vi "G_LCM.vi"() -> ()   [LabVIEW 2015]
panel:
  out "VISION_LANE_PT":T1={"hash"=5997167734802894298, "sys time"=0, "size"=0, "x"=[], "y"=[]} {"hash" format="%016x"}
  out "queue velo":refnum<queue>
  out "queue velo raw":refnum<queue>
  out "SLAM":T2={"hash"=8611666821338907869, "sys time"=0, "dt"=0.0, "x"=0.0, "y"=0.0, "speed"=0.0, "heading"=0.0, "yaw_rate"=0.0} {"hash" format="%016x"}
  out "VISION_STOPLINE":T3={"hash"=-9133130956553482184, "sys time"=0, "stopline_exist"=FALSE, "stopline_distance"=0.0} {"hash" format="%016x"}
  out "VISION_LANE":T4={"hash"=2187367745111948818, "sys time"=0, "left_lane_exist"=FALSE, "right_lane_exist"=FALSE, "left_lane_dot"=0.0, "right_lane_dot"=0.0} {"hash" format="%016x"}
  out "AVM":cluster{"hash":i64, "sys time":i64}={"hash"=-4935458055730020940, "sys time"=0} {"hash" format="%x"}
  out "queue ibeo":refnum<queue>
  out "CON_T 2":T5={"hash"=6240213546654873975, "sys time"=0, "Auto"=FALSE, "Run"=FALSE, "Solenoid"=FALSE, "T lim"=FALSE, "brk_enc"=0, "B PWM"=0, "T PWM"=0, "ref_vel"=0.0, "ref_bkr_enc"=0.0, "ref_apv"=0.0, "ref_steer"=0.0, "net address"=0} {"net address" format="%08x"; "hash" format="%016x"}
  out "VELO_384":T6={"hash"=-1208058655852198207, "sys time"=0, "Timestamp"=0, "Rot_ang"=[], "Ver_ang"=[], "Dist"=[], "Ver_off"=[], "Intensity"=[], "pos x"=0.0, "pos y"=0.0, "Heading"=0.0} {"hash" format="%016x"}
  out "VELO_RAW":T7={"hash"=6418264790525055119, "sys time"=0, "type"=0, "raw"=""} {"hash" format="%x"}
  out "ERROR_T":T8={"hash"=-3262420976274766845, "sys time"=0, "n"=0, "error"=[]} {"hash" format="%016x"}
  out "LCM Prius":T9={"connection ID"=refnum, "net address"=0, "port"=7667}
  out "ibeo":bool
  out "CON_INPUT_T 2":T10={"hash"=-1383086933477118758, "sys time"=0, "ref_vel"=0.0, "ref_steer"=0.0, "alert"=0} {"hash" format="%016x"}
  out "RGB_T":T11={"hash"=-8920902524919788889, "sys time"=0, "width"=0, "height"=0, "size"=0, "data"=[]} {"hash" format="%016x"}
  out "Mobileye name":string
  out "Mobileye_RAW_SNAP":T12={"hash"=-8920902524919788889, "sys time"=0, "size"=0, "data"=[]} {"hash" format="%016x"}
  out "car name":string
  out "CAN_CAR_RAW_T":T13={"hash"=-386282380061490012, "sys time"=0, "car time"=0, "ID"=0, "data"=[]} {"hash" format="%016x"}
  out "CAN_EYE_RAW_T":T14={"hash"=-386282380061490012, "sys time"=0, "mobileye time"=0, "ID"=0, "data"=[]} {"ID" format="%x"; "hash" format="%016x"}
  out "EURECAR_VISION":T15={"hash"=-7865610496642411282, "sys time"=0, "status"=0, "TS_num"=0, "TS_type"=[], "TS_loc_x"=[], "TS_loc_y"=[]} {"hash" format="%016x"}
  out "APP_GPS_DATA":T16={"hash"=3737605006820705978, "sys time"=0, "s_lat"=0.0, "s_lon"=0.0, "d_lat"=0.0, "d_lon"=0.0, "Message"=0} {"d_lon" format="%#_12g"; "d_lat" format="%#_12g"; "s_lon" format="%#_12g"; "s_lat" format="%#_12g"; "hash" format="%016x"}
  out "SDT_GPS_DATA":T17={"hash"=8129228807638357924, "sys time"=0, "lat"=0.0, "lon"=0.0} {"hash" format="%016x"}
  out "PATH_T":T18={"hash"=-968933064704923210, "sys time"=0, "n"=0, "pathxy"=[]} {"hash" format="%016x"}
  in  "recv data idx":string
  out "LANE_T":T19={"hash"=-8920902524919788889, "sys time"=0, "n"=0, "data1"=[], "data2"=[], "lat"=[], "lon"=[]} {"hash" format="%016x"}
  out "ALT_T":T20={"hash"=181950922177085156, "sys time"=0, "u time"=0, "alt"=0.0} {"hash" format="%016x"}
  out "CAN_T":T21={"hash"=4925705798588944810, "sys time"=0, "time"=0.0, "yaw_rate"=0.0, "mdps torque"=0.0, "mdps str_ang"=0.0, "VS_CAN"=0.0, "lat_accel"=0.0, "mcp"=0.0, "accel pedal value"=0.0, "tps"=0.0, "odometer"=0.0, "battery voltage"=0.0, "WHL_SPD_RR"=0.0, "WHL_SPD_RL"=0.0, "WHL_SPD_FR"=0.0, "WHL_SPD_FL"=0.0} {"time" format="%#_25g"; "hash" format="%016x"}
  out "VELO_PT_T":T22={"hash"=3444748642197318535, "sys time"=0, "Timestamp"=0, "Rotational angle"=[11547, 11564, 11580, 11596, 11614, 11630, 11647, 11663, 11678, 11696, 11714, 11730], "dist"=[[0, 0, 0, 0, 0, 0, 0, 0, 0, 0, 0, 0, 0, 0, 0, 0, 0, 0, 2933, 2909, 2901, 2913, 2913, 3042, 2913, 2924, 2867, 0, 0, 3082, 0, 4173], [0, 0, 0, 0, 0, 0, 0, 0, 0, 0, 0, 0, 0, 0, 0, 0, 0, 0, 2928, 2906, 2896, 2920, 2914, 3037, 2923, 2919, 2866, 3067, 4160, 4168, 4176, 4183], [0, 0, 0, 0, 0, 0, 0, 0, 0, 0, 0, 0, 0, 0, 0, 0, 0, 0, 2932, 2908, 2900, 2924, 2915, 3046, 2948, 2892, 0, 3056, 4173, 3080, 4176, 4182], [0, 0, 0, 0, 0, 0, 0, 0, 0, 0, 0, 0, 0, 0, 0, 0, 0, 0, 2917, 2916, 2898, 2921, 2926, 3049, 2926, 2890, 2869, 3063, 4175, 4177, 4185, 4181], [0, 0, 0, 0, 0, 0, 0, 0, 0, 0, 0, 0, 0, 0, 0, 0, 0, 0, 2932, 2895, 2917, 2923, 2920, 3056, 2902, 2894, 2873, 0, 3064, 4190, 4187, 4187], [0, 0, 0, 0, 0, 0, 0, 0, 0, 0, 0, 0, 0, 0, 0, 0, 0, 0, 2928, 2908, 2934, 2922, 2922, 3058, 2907, 2902, 2876, 0, 3071, 3087, 4190, 4195], [0, 0, 0, 0, 0, 0, 0, 0, 0, 0, 0, 0, 0, 0, 0, 0, 0, 0, 2921, 2910, 2917, 2920, 2915, 3061, 2903, 2909, 2882, 2984, 3076, 4179, 4197, 4197], [0, 0, 0, 0, 0, 0, 0, 0, 0, 0, 0, 0, 0, 0, 0, 0, 0, 0, 2956, 2909, 3073, 2933, 2944, 3064, 2923, 2914, 2884, 2986, 3083, 4186, 4202, 4204], [0, 0, 0, 0, 0, 0, 0, 0, 0, 0, 0, 0, 0, 0, 0, 0, 0, 0, 2933, 2919, 3070, 2902, 0, 3071, 2917, 2927, 2886, 2991, 3050, 4194, 4205, 4201], [0, 0, 0, 0, 0, 0, 0, 0, 0, 0, 0, 0, 0, 0, 0, 0, 0, 0, 2947, 2918, 3081, 0, 0, 3069, 2930, 2935, 2891, 2994, 0, 4196, 4211, 4216], [0, 0, 0, 0, 0, 0, 0, 0, 0, 0, 0, 0, 0, 0, 0, 0, 0, 0, 2943, 0, 3084, 0, 3048, 3072, 2942, 2929, 2892, 2999, 3049, 4193, 4213, 3113], [0, 0, 0, 0, 0, 0, 0, 0, 0, 0, 0, 0, 0, 0, 0, 0, 0, 0, 2938, 0, 3085, 3045, 3031, 3077, 2942, 2917, 2896, 2999, 3057, 4194, 4217, 3113]], "Intensity"=[[3, 1, 2, 5, 3, 4, 3, 1, 19, 11, 17, 13, 26, 10, 2, 1, 2, 2, 1, 2, 3, 0, 6, 3, 44, 40, 14, 1, 12, 1, 19, 2], [3, 1, 2, 5, 3, 4, 3, 1, 17, 11, 18, 13, 26, 12, 2, 1, 2, 2, 1, 3, 2, 0, 7, 3, 40, 19, 6, 0, 1, 1, 8, 3], [3, 1, 2, 5, 3, 4, 3, 1, 16, 11, 18, 15, 22, 10, 2, 1, 2, 2, 1, 3, 2, 0, 5, 3, 30, 18, 36, 0, 0, 0, 8, 2], [3, 1, 2, 5, 3, 4, 3, 1, 16, 11, 19, 13, 22, 12, 2, 1, 2, 2, 4, 1, 2, 0, 5, 3, 12, 31, 21, 0, 0, 1, 8, 2], [3, 1, 2, 5, 4, 4, 3, 1, 14, 10, 16, 12, 22, 12, 2, 1, 2, 2, 1, 2, 0, 0, 3, 3, 23, 35, 25, 33, 0, 0, 8, 2], [3, 1, 2, 3, 4, 4, 3, 1, 13, 8, 15, 11, 22, 10, 2, 1, 2, 2, 1, 2, 0, 1, 5, 3, 34, 9, 25, 49, 0, 0, 6, 2], [3, 1, 2, 3, 4, 4, 3, 1, 13, 8, 14, 9, 18, 12, 2, 1, 2, 2, 1, 1, 1, 0, 4, 3, 30, 21, 25, 30, 0, 1, 7, 2], [3, 1, 2, 5, 3, 4, 3, 1, 13, 7, 9, 8, 18, 10, 2, 1, 2, 2, 1, 1, 1, 0, 2, 3, 13, 25, 27, 33, 0, 2, 7, 2], [3, 1, 2, 3, 3, 4, 3, 1, 9, 5, 8, 6, 15, 8, 2, 1, 2, 2, 1, 2, 1, 0, 28, 3, 26, 14, 25, 39, 2, 2, 7, 2], [3, 1, 2, 3, 3, 3, 3, 1, 6, 5, 7, 5, 15, 8, 2, 1, 2, 2, 1, 0, 1, 1, 64, 3, 38, 15, 27, 44, 42, 2, 7, 1], [3, 1, 2, 3, 3, 3, 3, 1, 6, 5, 4, 5, 15, 8, 2, 1, 2, 2, 1, 2, 1, 1, 8, 3, 34, 15, 23, 42, 5, 2, 7, 0], [3, 1, 2, 5, 3, 3, 3, 1, 6, 5, 4, 5, 15, 8, 2, 1, 2, 2, 1, 2, 1, 0, 2, 3, 40, 18, 23, 42, 3, 2, 7, 0]], "pos_x"=0.0, "pos_y"=0.0, "pos_h"=0.0} {"hash" format="%x"}
  out "LCM 2 RIO":T9={"connection ID"=refnum, "net address"=0, "port"=7667}
  out "CON_INPUT_T":T23={"hash"=5270366413063349492, "sys time"=0, "ref_vel"=0.0, "ref_steer"=0.0} {"hash" format="%016x"}
  in  "recv data":string
  out "IBEO_2202_T":T24={"hash"=-5191723151767681935, "sys time"=0, "Header"={"Size of prev messages"=0, "Size of this messages"=8534, "Reserved"=0, "DeviceID"=0, "Data type"=8706, "NTP time"=30358766255088}, "Scan header"={"Scan number"=22632, "scanner status"=811, "Sync phase offset"=0, "Scan start time NTP"=30358508796168, "Scan end time NTP"=30358603880928, "Angle ticks per rotation"=11520, "Start angle"=0.8726646259971648, "End angle"=-0.8726646259971648, "Scan points"=849, "pos_x"=0.0, "pos_y"=0.0, "pos_h"=0.0, "Mounting position x"=3.5, "Mounting position y"=0.0, "Mounting position z"=0.45, "Reserved"=5}, "Scan points"=[{"flags"=0, "Echo"=0, "Radial distance"=20.2, "Horizontal angle"=0.8552113334772213, "Vertical angle"=-0.020943951023931952, "Echo pulse width"=92, "Reserved"=0}, {"flags"=0, "Echo"=0, "Radial distance"=20.05, "Horizontal angle"=0.8552113334772213, "Vertical angle"=-0.006981317007977317, "Echo pulse width"=48, "Reserved"=0}, {"flags"=0, "Echo"=0, "Radial distance"=20.21, "Horizontal angle"=0.8464846872172498, "Vertical angle"=-0.020943951023931952, "Echo pulse width"=80, "Reserved"=0}, {"flags"=0, "Echo"=0, "Radial distance"=20.03, "Horizontal angle"=0.8464846872172498, "Vertical angle"=-0.006981317007977317, "Echo pulse width"=120, "Reserved"=0}, {"flags"=0, "Echo"=0, "Radial distance"=20.400000000000002, "Horizontal angle"=0.8377580409572781, "Vertical angle"=-0.020943951023931952, "Echo pulse width"=136, "Reserved"=0}, {"flags"=0, "Echo"=0, "Radial distance"=20.080000000000002, "Horizontal angle"=0.8377580409572781, "Vertical angle"=-0.006981317007977317, "Echo pulse width"=132, "Reserved"=0}, {"flags"=0, "Echo"=0, "Radial distance"=20.67, "Horizontal angle"=0.8290313946973066, "Vertical angle"=-0.020943951023931952, "Echo pulse width"=124, "Reserved"=0}, {"flags"=0, "Echo"=0, "Radial distance"=20.37, "Horizontal angle"=0.8290313946973066, "Vertical angle"=-0.006981317007977317, "Echo pulse width"=144, "Reserved"=0}, {"flags"=5, "Echo"=0, "Radial distance"=20.830000000000002, "Horizontal angle"=0.8203047484373349, "Vertical angle"=-0.020943951023931952, "Echo pulse width"=72, "Reserved"=0}, {"flags"=4, "Echo"=1, "Radial distance"=21.87, "Horizontal angle"=0.8203047484373349, "Vertical angle"=-0.020943951023931952, "Echo pulse width"=124, "Reserved"=0}, {"flags"=4, "Echo"=0, "Radial distance"=21.88, "Horizontal angle"=0.8115781021773633, "Vertical angle"=-0.020943951023931952, "Echo pulse width"=132, "Reserved"=0}, {"flags"=4, "Echo"=0, "Radial distance"=21.78, "Horizontal angle"=0.8028514559173915, "Vertical angle"=-0.020943951023931952, "Echo pulse width"=156, "Reserved"=0}, {"flags"=4, "Echo"=0, "Radial distance"=21.76, "Horizontal angle"=0.7941248096574199, "Vertical angle"=-0.020943951023931952, "Echo pulse width"=176, "Reserved"=0}, {"flags"=1, "Echo"=0, "Radial distance"=23.37, "Horizontal angle"=0.7941248096574199, "Vertical angle"=-0.006981317007977317, "Echo pulse width"=100, "Reserved"=1}, {"flags"=0, "Echo"=1, "Radial distance"=48.230000000000004, "Horizontal angle"=0.7941248096574199, "Vertical angle"=-0.006981317007977317, "Echo pulse width"=120, "Reserved"=2}, {"flags"=4, "Echo"=0, "Radial distance"=21.76, "Horizontal angle"=0.7853981633974483, "Vertical angle"=-0.020943951023931952, "Echo pulse width"=172, "Reserved"=0}, {"flags"=1, "Echo"=0, "Radial distance"=23.25, "Horizontal angle"=0.7853981633974483, "Vertical angle"=-0.006981317007977317, "Echo pulse width"=144, "Reserved"=1}, {"flags"=0, "Echo"=1, "Radial distance"=48.02, "Horizontal angle"=0.7853981633974483, "Vertical angle"=-0.006981317007977317, "Echo pulse width"=108, "Reserved"=2}, {"flags"=0, "Echo"=0, "Radial distance"=16.740000000000002, "Horizontal angle"=0.7766715171374766, "Vertical angle"=-0.020943951023931952, "Echo pulse width"=156, "Reserved"=3}, {"flags"=0, "Echo"=0, "Radial distance"=16.77, "Horizontal angle"=0.7766715171374766, "Vertical angle"=-0.006981317007977317, "Echo pulse width"=152, "Reserved"=3}, {"flags"=5, "Echo"=0, "Radial distance"=5.44, "Horizontal angle"=0.767944870877505, "Vertical angle"=-0.020943951023931952, "Echo pulse width"=136, "Reserved"=0}, {"flags"=4, "Echo"=1, "Radial distance"=21.87, "Horizontal angle"=0.767944870877505, "Vertical angle"=-0.020943951023931952, "Echo pulse width"=164, "Reserved"=0}, {"flags"=1, "Echo"=0, "Radial distance"=23.17, "Horizontal angle"=0.767944870877505, "Vertical angle"=-0.006981317007977317, "Echo pulse width"=148, "Reserved"=1}, {"flags"=0, "Echo"=1, "Radial distance"=48.18, "Horizontal angle"=0.767944870877505, "Vertical angle"=-0.006981317007977317, "Echo pulse width"=108, "Reserved"=4}, {"flags"=4, "Echo"=0, "Radial distance"=22.03, "Horizontal angle"=0.7592182246175333, "Vertical angle"=-0.020943951023931952, "Echo pulse width"=164, "Reserved"=0}, {"flags"=0, "Echo"=0, "Radial distance"=23.3, "Horizontal angle"=0.7592182246175333, "Vertical angle"=-0.006981317007977317, "Echo pulse width"=168, "Reserved"=1}, {"flags"=5, "Echo"=0, "Radial distance"=5.21, "Horizontal angle"=0.7504915783575618, "Vertical angle"=-0.020943951023931952, "Echo pulse width"=144, "Reserved"=0}, {"flags"=4, "Echo"=1, "Radial distance"=22.27, "Horizontal angle"=0.7504915783575618, "Vertical angle"=-0.020943951023931952, "Echo pulse width"=164, "Reserved"=0}, {"flags"=0, "Echo"=0, "Radial distance"=23.34, "Horizontal angle"=0.7504915783575618, "Vertical angle"=-0.006981317007977317, "Echo pulse width"=172, "Reserved"=1}, {"flags"=5, "Echo"=0, "Radial distance"=20.36, "Horizontal angle"=0.74176493209759, "Vertical angle"=-0.020943951023931952, "Echo pulse width"=68, "Reserved"=0}, {"flags"=4, "Echo"=1, "Radial distance"=22.42, "Horizontal angle"=0.74176493209759, "Vertical angle"=-0.020943951023931952, "Echo pulse width"=152, "Reserved"=0}, {"flags"=0, "Echo"=0, "Radial distance"=23.38, "Horizontal angle"=0.74176493209759, "Vertical angle"=-0.006981317007977317, "Echo pulse width"=168, "Reserved"=1}, {"flags"=5, "Echo"=0, "Radial distance"=5.5600000000000005, "Horizontal angle"=0.7330382858376184, "Vertical angle"=-0.020943951023931952, "Echo pulse width"=168, "Reserved"=0}, {"flags"=4, "Echo"=1, "Radial distance"=22.62, "Horizontal angle"=0.7330382858376184, "Vertical angle"=-0.020943951023931952, "Echo pulse width"=152, "Reserved"=0}, {"flags"=1, "Echo"=0, "Radial distance"=23.37, "Horizontal angle"=0.7330382858376184, "Vertical angle"=-0.006981317007977317, "Echo pulse width"=156, "Reserved"=1}, {"flags"=0, "Echo"=1, "Radial distance"=48.21, "Horizontal angle"=0.7330382858376184, "Vertical angle"=-0.006981317007977317, "Echo pulse width"=72, "Reserved"=5}, {"flags"=5, "Echo"=0, "Radial distance"=5.58, "Horizontal angle"=0.7243116395776468, "Vertical angle"=-0.020943951023931952, "Echo pulse width"=136, "Reserved"=0}, {"flags"=5, "Echo"=1, "Radial distance"=20.88, "Horizontal angle"=0.7243116395776468, "Vertical angle"=-0.020943951023931952, "Echo pulse width"=64, "Reserved"=0}, {"flags"=4, "Echo"=2, "Radial distance"=22.77, "Horizontal angle"=0.7243116395776468, "Vertical angle"=-0.020943951023931952, "Echo pulse width"=148, "Reserved"=0}, {"flags"=0, "Echo"=0, "Radial distance"=23.62, "Horizontal angle"=0.7243116395776468, "Vertical angle"=-0.006981317007977317, "Echo pulse width"=172, "Reserved"=1}, {"flags"=5, "Echo"=0, "Radial distance"=5.63, "Horizontal angle"=0.7155849933176751, "Vertical angle"=-0.020943951023931952, "Echo pulse width"=196, "Reserved"=0}, {"flags"=4, "Echo"=1, "Radial distance"=22.69, "Horizontal angle"=0.7155849933176751, "Vertical angle"=-0.020943951023931952, "Echo pulse width"=212, "Reserved"=0}, {"flags"=0, "Echo"=0, "Radial distance"=23.82, "Horizontal angle"=0.7155849933176751, "Vertical angle"=-0.006981317007977317, "Echo pulse width"=160, "Reserved"=1}, {"flags"=5, "Echo"=0, "Radial distance"=5.67, "Horizontal angle"=0.7068583470577035, "Vertical angle"=-0.020943951023931952, "Echo pulse width"=172, "Reserved"=0}, {"flags"=4, "Echo"=1, "Radial distance"=23.16, "Horizontal angle"=0.7068583470577035, "Vertical angle"=-0.020943951023931952, "Echo pulse width"=176, "Reserved"=0}, {"flags"=0, "Echo"=0, "Radial distance"=23.62, "Horizontal angle"=0.7068583470577035, "Vertical angle"=-0.006981317007977317, "Echo pulse width"=164, "Reserved"=1}, {"flags"=5, "Echo"=0, "Radial distance"=5.53, "Horizontal angle"=0.6981317007977318, "Vertical angle"=-0.020943951023931952, "Echo pulse width"=208, "Reserved"=0}, {"flags"=0, "Echo"=1, "Radial distance"=23.35, "Horizontal angle"=0.6981317007977318, "Vertical angle"=-0.020943951023931952, "Echo pulse width"=160, "Reserved"=1}, {"flags"=0, "Echo"=0, "Radial distance"=23.650000000000002, "Horizontal angle"=0.6981317007977318, "Vertical angle"=-0.006981317007977317, "Echo pulse width"=148, "Reserved"=1}, {"flags"=5, "Echo"=0, "Radial distance"=5.55, "Horizontal angle"=0.6894050545377601, "Vertical angle"=-0.020943951023931952, "Echo pulse width"=192, "Reserved"=0}, {"flags"=0, "Echo"=1, "Radial distance"=23.55, "Horizontal angle"=0.6894050545377601, "Vertical angle"=-0.020943951023931952, "Echo pulse width"=160, "Reserved"=1}, {"flags"=0, "Echo"=0, "Radial distance"=23.62, "Horizontal angle"=0.6894050545377601, "Vertical angle"=-0.006981317007977317, "Echo pulse width"=160, "Reserved"=1}, {"flags"=5, "Echo"=0, "Radial distance"=5.5600000000000005, "Horizontal angle"=0.6806784082777886, "Vertical angle"=-0.020943951023931952, "Echo pulse width"=236, "Reserved"=0}, {"flags"=0, "Echo"=1, "Radial distance"=23.77, "Horizontal angle"=0.6806784082777886, "Vertical angle"=-0.020943951023931952, "Echo pulse width"=144, "Reserved"=1}, {"flags"=0, "Echo"=0, "Radial distance"=23.61, "Horizontal angle"=0.6806784082777886, "Vertical angle"=-0.006981317007977317, "Echo pulse width"=156, "Reserved"=1}, {"flags"=5, "Echo"=0, "Radial distance"=5.5200000000000005, "Horizontal angle"=0.6719517620178168, "Vertical angle"=-0.020943951023931952, "Echo pulse width"=220, "Reserved"=0}, {"flags"=4, "Echo"=1, "Radial distance"=24.17, "Horizontal angle"=0.6719517620178168, "Vertical angle"=-0.020943951023931952, "Echo pulse width"=148, "Reserved"=0}, {"flags"=0, "Echo"=0, "Radial distance"=23.66, "Horizontal angle"=0.6719517620178168, "Vertical angle"=-0.006981317007977317, "Echo pulse width"=164, "Reserved"=1}, {"flags"=5, "Echo"=0, "Radial distance"=5.67, "Horizontal angle"=0.6632251157578453, "Vertical angle"=-0.020943951023931952, "Echo pulse width"=224, "Reserved"=0}, {"flags"=4, "Echo"=1, "Radial distance"=24.45, "Horizontal angle"=0.6632251157578453, "Vertical angle"=-0.020943951023931952, "Echo pulse width"=148, "Reserved"=0}, {"flags"=1, "Echo"=0, "Radial distance"=32.230000000000004, "Horizontal angle"=0.6632251157578453, "Vertical angle"=-0.006981317007977317, "Echo pulse width"=40, "Reserved"=6}, {"flags"=0, "Echo"=1, "Radial distance"=35.42, "Horizontal angle"=0.6632251157578453, "Vertical angle"=-0.006981317007977317, "Echo pulse width"=164, "Reserved"=7}, {"flags"=5, "Echo"=0, "Radial distance"=5.63, "Horizontal angle"=0.6544984694978736, "Vertical angle"=-0.020943951023931952, "Echo pulse width"=208, "Reserved"=0}, {"flags"=4, "Echo"=1, "Radial distance"=24.73, "Horizontal angle"=0.6544984694978736, "Vertical angle"=-0.020943951023931952, "Echo pulse width"=144, "Reserved"=0}, {"flags"=0, "Echo"=0, "Radial distance"=35.14, "Horizontal angle"=0.6544984694978736, "Vertical angle"=-0.006981317007977317, "Echo pulse width"=164, "Reserved"=7}, {"flags"=5, "Echo"=0, "Radial distance"=5.64, "Horizontal angle"=0.6457718232379019, "Vertical angle"=-0.020943951023931952, "Echo pulse width"=244, "Reserved"=0}, {"flags"=4, "Echo"=1, "Radial distance"=25.04, "Horizontal angle"=0.6457718232379019, "Vertical angle"=-0.020943951023931952, "Echo pulse width"=132, "Reserved"=0}, {"flags"=0, "Echo"=0, "Radial distance"=35.01, "Horizontal angle"=0.6457718232379019, "Vertical angle"=-0.006981317007977317, "Echo pulse width"=156, "Reserved"=7}, {"flags"=5, "Echo"=0, "Radial distance"=5.71, "Horizontal angle"=0.6370451769779303, "Vertical angle"=-0.020943951023931952, "Echo pulse width"=264, "Reserved"=0}, {"flags"=4, "Echo"=1, "Radial distance"=25.6, "Horizontal angle"=0.6370451769779303, "Vertical angle"=-0.020943951023931952, "Echo pulse width"=132, "Reserved"=0}, {"flags"=1, "Echo"=0, "Radial distance"=32.68, "Horizontal angle"=0.6370451769779303, "Vertical angle"=-0.006981317007977317, "Echo pulse width"=56, "Reserved"=8}, {"flags"=0, "Echo"=1, "Radial distance"=34.86, "Horizontal angle"=0.6370451769779303, "Vertical angle"=-0.006981317007977317, "Echo pulse width"=160, "Reserved"=7}, {"flags"=5, "Echo"=0, "Radial distance"=5.63, "Horizontal angle"=0.6283185307179586, "Vertical angle"=-0.020943951023931952, "Echo pulse width"=296, "Reserved"=0}, {"flags"=4, "Echo"=1, "Radial distance"=25.84, "Horizontal angle"=0.6283185307179586, "Vertical angle"=-0.020943951023931952, "Echo pulse width"=92, "Reserved"=0}, {"flags"=5, "Echo"=0, "Radial distance"=7.54, "Horizontal angle"=0.6283185307179586, "Vertical angle"=-0.006981317007977317, "Echo pulse width"=168, "Reserved"=0}, {"flags"=0, "Echo"=1, "Radial distance"=34.87, "Horizontal angle"=0.6283185307179586, "Vertical angle"=-0.006981317007977317, "Echo pulse width"=124, "Reserved"=7}, {"flags"=4, "Echo"=0, "Radial distance"=5.67, "Horizontal angle"=0.619591884457987, "Vertical angle"=-0.020943951023931952, "Echo pulse width"=272, "Reserved"=0}, {"flags"=4, "Echo"=0, "Radial distance"=7.38, "Horizontal angle"=0.619591884457987, "Vertical angle"=-0.006981317007977317, "Echo pulse width"=204, "Reserved"=0}, {"flags"=4, "Echo"=0, "Radial distance"=5.67, "Horizontal angle"=0.6108652381980153, "Vertical angle"=-0.020943951023931952, "Echo pulse width"=284, "Reserved"=0}, {"flags"=0, "Echo"=0, "Radial distance"=7.33, "Horizontal angle"=0.6108652381980153, "Vertical angle"=-0.006981317007977317, "Echo pulse width"=224, "Reserved"=9}, {"flags"=0, "Echo"=0, "Radial distance"=7.21, "Horizontal angle"=0.6065019150680295, "Vertical angle"=0.00698131700797732, "Echo pulse width"=124, "Reserved"=9}, {"flags"=0, "Echo"=0, "Radial distance"=7.08, "Horizontal angle"=0.6065019150680295, "Vertical angle"=0.020943951023931963, "Echo pulse width"=120, "Reserved"=9}, {"flags"=4, "Echo"=0, "Radial distance"=5.79, "Horizontal angle"=0.6021385919380438, "Vertical angle"=-0.020943951023931952, "Echo pulse width"=248, "Reserved"=0}, {"flags"=0, "Echo"=0, "Radial distance"=7.09, "Horizontal angle"=0.6021385919380438, "Vertical angle"=-0.006981317007977317, "Echo pulse width"=232, "Reserved"=9}, {"flags"=0, "Echo"=0, "Radial distance"=7.24, "Horizontal angle"=0.5977752688080579, "Vertical angle"=0.00698131700797732, "Echo pulse width"=72, "Reserved"=9}, {"flags"=0, "Echo"=0, "Radial distance"=6.99, "Horizontal angle"=0.5977752688080579, "Vertical angle"=0.020943951023931963, "Echo pulse width"=60, "Reserved"=9}, {"flags"=4, "Echo"=0, "Radial distance"=5.75, "Horizontal angle"=0.593411945678072, "Vertical angle"=-0.020943951023931952, "Echo pulse width"=268, "Reserved"=0}, {"flags"=0, "Echo"=0, "Radial distance"=6.84, "Horizontal angle"=0.593411945678072, "Vertical angle"=-0.006981317007977317, "Echo pulse width"=284, "Reserved"=9}, {"flags"=0, "Echo"=0, "Radial distance"=7.140000000000001, "Horizontal angle"=0.5890486225480862, "Vertical angle"=0.00698131700797732, "Echo pulse width"=160, "Reserved"=9}, {"flags"=0, "Echo"=0, "Radial distance"=6.98, "Horizontal angle"=0.5890486225480862, "Vertical angle"=0.020943951023931963, "Echo pulse width"=144, "Reserved"=9}, {"flags"=4, "Echo"=0, "Radial distance"=5.79, "Horizontal angle"=0.5846852994181004, "Vertical angle"=-0.020943951023931952, "Echo pulse width"=236, "Reserved"=0}, {"flags"=0, "Echo"=0, "Radial distance"=6.95, "Horizontal angle"=0.5846852994181004, "Vertical angle"=-0.006981317007977317, "Echo pulse width"=264, "Reserved"=9}, {"flags"=0, "Echo"=0, "Radial distance"=7.03, "Horizontal angle"=0.5803219762881145, "Vertical angle"=0.00698131700797732, "Echo pulse width"=112, "Reserved"=9}, {"flags"=0, "Echo"=0, "Radial distance"=6.8, "Horizontal angle"=0.5803219762881145, "Vertical angle"=0.020943951023931963, "Echo pulse width"=104, "Reserved"=9}, {"flags"=4, "Echo"=0, "Radial distance"=5.67, "Horizontal angle"=0.5759586531581287, "Vertical angle"=-0.020943951023931952, "Echo pulse width"=268, "Reserved"=0}, {"flags"=0, "Echo"=0, "Radial distance"=6.76, "Horizontal angle"=0.5759586531581287, "Vertical angle"=-0.006981317007977317, "Echo pulse width"=288, "Reserved"=9}, {"flags"=0, "Echo"=0, "Radial distance"=7.0200000000000005, "Horizontal angle"=0.5715953300281429, "Vertical angle"=0.00698131700797732, "Echo pulse width"=168, "Reserved"=9}, {"flags"=0, "Echo"=0, "Radial distance"=6.91, "Horizontal angle"=0.5715953300281429, "Vertical angle"=0.020943951023931963, "Echo pulse width"=156, "Reserved"=9}, {"flags"=4, "Echo"=0, "Radial distance"=5.76, "Horizontal angle"=0.5672320068981571, "Vertical angle"=-0.020943951023931952, "Echo pulse width"=216, "Reserved"=0}, {"flags"=0, "Echo"=0, "Radial distance"=6.71, "Horizontal angle"=0.5672320068981571, "Vertical angle"=-0.006981317007977317, "Echo pulse width"=264, "Reserved"=9}, {"flags"=0, "Echo"=0, "Radial distance"=7.08, "Horizontal angle"=0.5628686837681712, "Vertical angle"=0.00698131700797732, "Echo pulse width"=136, "Reserved"=9}, {"flags"=0, "Echo"=0, "Radial distance"=6.8100000000000005, "Horizontal angle"=0.5628686837681712, "Vertical angle"=0.020943951023931963, "Echo pulse width"=112, "Reserved"=9}, {"flags"=4, "Echo"=0, "Radial distance"=5.79, "Horizontal angle"=0.5585053606381855, "Vertical angle"=-0.020943951023931952, "Echo pulse width"=248, "Reserved"=0}, {"flags"=0, "Echo"=0, "Radial distance"=6.6000000000000005, "Horizontal angle"=0.5585053606381855, "Vertical angle"=-0.006981317007977317, "Echo pulse width"=256, "Reserved"=9}, {"flags"=0, "Echo"=0, "Radial distance"=6.95, "Horizontal angle"=0.5541420375081997, "Vertical angle"=0.00698131700797732, "Echo pulse width"=176, "Reserved"=9}, {"flags"=0, "Echo"=0, "Radial distance"=6.75, "Horizontal angle"=0.5541420375081997, "Vertical angle"=0.020943951023931963, "Echo pulse width"=160, "Reserved"=9}, {"flags"=4, "Echo"=0, "Radial distance"=5.8100000000000005, "Horizontal angle"=0.5497787143782138, "Vertical angle"=-0.020943951023931952, "Echo pulse width"=204, "Reserved"=0}, {"flags"=0, "Echo"=0, "Radial distance"=6.61, "Horizontal angle"=0.5497787143782138, "Vertical angle"=-0.006981317007977317, "Echo pulse width"=224, "Reserved"=9}, {"flags"=0, "Echo"=0, "Radial distance"=6.88, "Horizontal angle"=0.5454153912482279, "Vertical angle"=0.00698131700797732, "Echo pulse width"=140, "Reserved"=9}, {"flags"=0, "Echo"=0, "Radial distance"=6.65, "Horizontal angle"=0.5454153912482279, "Vertical angle"=0.020943951023931963, "Echo pulse width"=124, "Reserved"=9}, {"flags"=4, "Echo"=0, "Radial distance"=5.8, "Horizontal angle"=0.5410520681182421, "Vertical angle"=-0.020943951023931952, "Echo pulse width"=232, "Reserved"=0}, {"flags"=0, "Echo"=0, "Radial distance"=6.65, "Horizontal angle"=0.5410520681182421, "Vertical angle"=-0.006981317007977317, "Echo pulse width"=232, "Reserved"=9}, {"flags"=0, "Echo"=0, "Radial distance"=6.91, "Horizontal angle"=0.5366887449882564, "Vertical angle"=0.00698131700797732, "Echo pulse width"=192, "Reserved"=9}, {"flags"=0, "Echo"=0, "Radial distance"=6.67, "Horizontal angle"=0.5366887449882564, "Vertical angle"=0.020943951023931963, "Echo pulse width"=160, "Reserved"=9}, {"flags"=4, "Echo"=0, "Radial distance"=5.91, "Horizontal angle"=0.5323254218582705, "Vertical angle"=-0.020943951023931952, "Echo pulse width"=196, "Reserved"=0}, {"flags"=0, "Echo"=0, "Radial distance"=6.7, "Horizontal angle"=0.5323254218582705, "Vertical angle"=-0.006981317007977317, "Echo pulse width"=200, "Reserved"=9}, {"flags"=0, "Echo"=0, "Radial distance"=6.72, "Horizontal angle"=0.5279620987282847, "Vertical angle"=0.00698131700797732, "Echo pulse width"=136, "Reserved"=9}, {"flags"=0, "Echo"=0, "Radial distance"=6.66, "Horizontal angle"=0.5279620987282847, "Vertical angle"=0.020943951023931963, "Echo pulse width"=144, "Reserved"=9}, {"flags"=4, "Echo"=0, "Radial distance"=5.91, "Horizontal angle"=0.5235987755982988, "Vertical angle"=-0.020943951023931952, "Echo pulse width"=224, "Reserved"=0}, {"flags"=0, "Echo"=0, "Radial distance"=6.72, "Horizontal angle"=0.5235987755982988, "Vertical angle"=-0.006981317007977317, "Echo pulse width"=220, "Reserved"=9}, {"flags"=0, "Echo"=0, "Radial distance"=6.87, "Horizontal angle"=0.519235452468313, "Vertical angle"=0.00698131700797732, "Echo pulse width"=180, "Reserved"=9}, {"flags"=0, "Echo"=0, "Radial distance"=6.68, "Horizontal angle"=0.519235452468313, "Vertical angle"=0.020943951023931963, "Echo pulse width"=180, "Reserved"=9}, {"flags"=4, "Echo"=0, "Radial distance"=6.03, "Horizontal angle"=0.5148721293383272, "Vertical angle"=-0.020943951023931952, "Echo pulse width"=192, "Reserved"=0}, {"flags"=0, "Echo"=0, "Radial distance"=6.68, "Horizontal angle"=0.5148721293383272, "Vertical angle"=-0.006981317007977317, "Echo pulse width"=208, "Reserved"=9}, {"flags"=0, "Echo"=0, "Radial distance"=7.01, "Horizontal angle"=0.5105088062083414, "Vertical angle"=0.00698131700797732, "Echo pulse width"=176, "Reserved"=9}, {"flags"=0, "Echo"=0, "Radial distance"=6.62, "Horizontal angle"=0.5105088062083414, "Vertical angle"=0.020943951023931963, "Echo pulse width"=148, "Reserved"=9}, {"flags"=4, "Echo"=0, "Radial distance"=5.99, "Horizontal angle"=0.5061454830783556, "Vertical angle"=-0.020943951023931952, "Echo pulse width"=216, "Reserved"=0}, {"flags"=0, "Echo"=0, "Radial distance"=6.6000000000000005, "Horizontal angle"=0.5061454830783556, "Vertical angle"=-0.006981317007977317, "Echo pulse width"=220, "Reserved"=9}, {"flags"=0, "Echo"=0, "Radial distance"=6.82, "Horizontal angle"=0.5017821599483697, "Vertical angle"=0.00698131700797732, "Echo pulse width"=200, "Reserved"=9}, {"flags"=0, "Echo"=0, "Radial distance"=6.640000000000001, "Horizontal angle"=0.5017821599483697, "Vertical angle"=0.020943951023931963, "Echo pulse width"=180, "Reserved"=9}, {"flags"=4, "Echo"=0, "Radial distance"=6.09, "Horizontal angle"=0.4974188368183839, "Vertical angle"=-0.020943951023931952, "Echo pulse width"=188, "Reserved"=0}, {"flags"=0, "Echo"=0, "Radial distance"=6.66, "Horizontal angle"=0.4974188368183839, "Vertical angle"=-0.006981317007977317, "Echo pulse width"=204, "Reserved"=9}, {"flags"=0, "Echo"=0, "Radial distance"=6.79, "Horizontal angle"=0.49305551368839806, "Vertical angle"=0.00698131700797732, "Echo pulse width"=160, "Reserved"=9}, {"flags"=0, "Echo"=0, "Radial distance"=6.59, "Horizontal angle"=0.49305551368839806, "Vertical angle"=0.020943951023931963, "Echo pulse width"=160, "Reserved"=9}, {"flags"=4, "Echo"=0, "Radial distance"=6.15, "Horizontal angle"=0.4886921905584123, "Vertical angle"=-0.020943951023931952, "Echo pulse width"=216, "Reserved"=0}, {"flags"=0, "Echo"=0, "Radial distance"=6.71, "Horizontal angle"=0.4886921905584123, "Vertical angle"=-0.006981317007977317, "Echo pulse width"=200, "Reserved"=9}, {"flags"=0, "Echo"=0, "Radial distance"=6.6000000000000005, "Horizontal angle"=0.48432886742842646, "Vertical angle"=0.00698131700797732, "Echo pulse width"=184, "Reserved"=9}, {"flags"=0, "Echo"=0, "Radial distance"=6.5200000000000005, "Horizontal angle"=0.48432886742842646, "Vertical angle"=0.020943951023931963, "Echo pulse width"=176, "Reserved"=9}, {"flags"=4, "Echo"=0, "Radial distance"=6.15, "Horizontal angle"=0.4799655442984406, "Vertical angle"=-0.020943951023931952, "Echo pulse width"=196, "Reserved"=0}, {"flags"=0, "Echo"=0, "Radial distance"=6.72, "Horizontal angle"=0.4799655442984406, "Vertical angle"=-0.006981317007977317, "Echo pulse width"=184, "Reserved"=9}, {"flags"=0, "Echo"=0, "Radial distance"=6.71, "Horizontal angle"=0.47560222116845474, "Vertical angle"=0.00698131700797732, "Echo pulse width"=184, "Reserved"=9}, {"flags"=0, "Echo"=0, "Radial distance"=6.63, "Horizontal angle"=0.47560222116845474, "Vertical angle"=0.020943951023931963, "Echo pulse width"=168, "Reserved"=9}, {"flags"=4, "Echo"=0, "Radial distance"=6.15, "Horizontal angle"=0.47123889803846897, "Vertical angle"=-0.020943951023931952, "Echo pulse width"=224, "Reserved"=0}, {"flags"=0, "Echo"=0, "Radial distance"=6.68, "Horizontal angle"=0.47123889803846897, "Vertical angle"=-0.006981317007977317, "Echo pulse width"=196, "Reserved"=9}, {"flags"=0, "Echo"=0, "Radial distance"=6.6000000000000005, "Horizontal angle"=0.46687557490848314, "Vertical angle"=0.00698131700797732, "Echo pulse width"=188, "Reserved"=9}, {"flags"=0, "Echo"=0, "Radial distance"=6.6000000000000005, "Horizontal angle"=0.46687557490848314, "Vertical angle"=0.020943951023931963, "Echo pulse width"=196, "Reserved"=9}, {"flags"=4, "Echo"=0, "Radial distance"=6.13, "Horizontal angle"=0.4625122517784973, "Vertical angle"=-0.020943951023931952, "Echo pulse width"=204, "Reserved"=0}, {"flags"=0, "Echo"=0, "Radial distance"=6.63, "Horizontal angle"=0.4625122517784973, "Vertical angle"=-0.006981317007977317, "Echo pulse width"=192, "Reserved"=9}, {"flags"=0, "Echo"=0, "Radial distance"=6.57, "Horizontal angle"=0.45814892864851153, "Vertical angle"=0.00698131700797732, "Echo pulse width"=172, "Reserved"=9}, {"flags"=0, "Echo"=0, "Radial distance"=6.63, "Horizontal angle"=0.45814892864851153, "Vertical angle"=0.020943951023931963, "Echo pulse width"=180, "Reserved"=9}, {"flags"=4, "Echo"=0, "Radial distance"=6.3100000000000005, "Horizontal angle"=0.45378560551852565, "Vertical angle"=-0.020943951023931952, "Echo pulse width"=220, "Reserved"=0}, {"flags"=0, "Echo"=0, "Radial distance"=6.67, "Horizontal angle"=0.45378560551852565, "Vertical angle"=-0.006981317007977317, "Echo pulse width"=200, "Reserved"=9}, {"flags"=0, "Echo"=0, "Radial distance"=6.63, "Horizontal angle"=0.4494222823885398, "Vertical angle"=0.00698131700797732, "Echo pulse width"=192, "Reserved"=9}, {"flags"=0, "Echo"=0, "Radial distance"=6.49, "Horizontal angle"=0.4494222823885398, "Vertical angle"=0.020943951023931963, "Echo pulse width"=184, "Reserved"=9}, {"flags"=4, "Echo"=0, "Radial distance"=6.2700000000000005, "Horizontal angle"=0.445058959258554, "Vertical angle"=-0.020943951023931952, "Echo pulse width"=196, "Reserved"=0}, {"flags"=0, "Echo"=0, "Radial distance"=6.59, "Horizontal angle"=0.445058959258554, "Vertical angle"=-0.006981317007977317, "Echo pulse width"=196, "Reserved"=9}, {"flags"=0, "Echo"=0, "Radial distance"=6.53, "Horizontal angle"=0.4406956361285682, "Vertical angle"=0.00698131700797732, "Echo pulse width"=172, "Reserved"=9}, {"flags"=0, "Echo"=0, "Radial distance"=6.51, "Horizontal angle"=0.4406956361285682, "Vertical angle"=0.020943951023931963, "Echo pulse width"=172, "Reserved"=9}, {"flags"=4, "Echo"=0, "Radial distance"=6.3500000000000005, "Horizontal angle"=0.4363323129985824, "Vertical angle"=-0.020943951023931952, "Echo pulse width"=220, "Reserved"=0}, {"flags"=0, "Echo"=0, "Radial distance"=6.67, "Horizontal angle"=0.4363323129985824, "Vertical angle"=-0.006981317007977317, "Echo pulse width"=204, "Reserved"=9}, {"flags"=0, "Echo"=0, "Radial distance"=6.5600000000000005, "Horizontal angle"=0.4319689898685966, "Vertical angle"=0.00698131700797732, "Echo pulse width"=188, "Reserved"=9}, {"flags"=0, "Echo"=0, "Radial distance"=6.5200000000000005, "Horizontal angle"=0.4319689898685966, "Vertical angle"=0.020943951023931963, "Echo pulse width"=192, "Reserved"=9}, {"flags"=0, "Echo"=0, "Radial distance"=6.390000000000001, "Horizontal angle"=0.42760566673861067, "Vertical angle"=-0.020943951023931952, "Echo pulse width"=192, "Reserved"=9}, {"flags"=0, "Echo"=0, "Radial distance"=6.71, "Horizontal angle"=0.42760566673861067, "Vertical angle"=-0.006981317007977317, "Echo pulse width"=192, "Reserved"=9}, {"flags"=0, "Echo"=0, "Radial distance"=6.49, "Horizontal angle"=0.4232423436086249, "Vertical angle"=0.00698131700797732, "Echo pulse width"=168, "Reserved"=9}, {"flags"=0, "Echo"=0, "Radial distance"=6.51, "Horizontal angle"=0.4232423436086249, "Vertical angle"=0.020943951023931963, "Echo pulse width"=168, "Reserved"=9}, {"flags"=0, "Echo"=0, "Radial distance"=6.41, "Horizontal angle"=0.41887902047863906, "Vertical angle"=-0.020943951023931952, "Echo pulse width"=212, "Reserved"=9}, {"flags"=0, "Echo"=0, "Radial distance"=6.76, "Horizontal angle"=0.41887902047863906, "Vertical angle"=-0.006981317007977317, "Echo pulse width"=216, "Reserved"=9}, {"flags"=0, "Echo"=0, "Radial distance"=6.66, "Horizontal angle"=0.4145156973486533, "Vertical angle"=0.00698131700797732, "Echo pulse width"=204, "Reserved"=9}, {"flags"=0, "Echo"=0, "Radial distance"=6.49, "Horizontal angle"=0.4145156973486533, "Vertical angle"=0.020943951023931963, "Echo pulse width"=188, "Reserved"=9}, {"flags"=0, "Echo"=0, "Radial distance"=6.47, "Horizontal angle"=0.41015237421866746, "Vertical angle"=-0.020943951023931952, "Echo pulse width"=180, "Reserved"=9}, {"flags"=0, "Echo"=0, "Radial distance"=6.71, "Horizontal angle"=0.41015237421866746, "Vertical angle"=-0.006981317007977317, "Echo pulse width"=192, "Reserved"=9}, {"flags"=0, "Echo"=0, "Radial distance"=6.69, "Horizontal angle"=0.40578905108868163, "Vertical angle"=0.00698131700797732, "Echo pulse width"=176, "Reserved"=9}, {"flags"=0, "Echo"=0, "Radial distance"=6.51, "Horizontal angle"=0.40578905108868163, "Vertical angle"=0.020943951023931963, "Echo pulse width"=176, "Reserved"=9}, {"flags"=0, "Echo"=0, "Radial distance"=6.53, "Horizontal angle"=0.40142572795869574, "Vertical angle"=-0.020943951023931952, "Echo pulse width"=208, "Reserved"=9}, {"flags"=0, "Echo"=0, "Radial distance"=6.71, "Horizontal angle"=0.40142572795869574, "Vertical angle"=-0.006981317007977317, "Echo pulse width"=200, "Reserved"=9}, {"flags"=0, "Echo"=0, "Radial distance"=6.79, "Horizontal angle"=0.39706240482870997, "Vertical angle"=0.00698131700797732, "Echo pulse width"=220, "Reserved"=9}, {"flags"=0, "Echo"=0, "Radial distance"=6.72, "Horizontal angle"=0.39706240482870997, "Vertical angle"=0.020943951023931963, "Echo pulse width"=220, "Reserved"=9}, {"flags"=0, "Echo"=0, "Radial distance"=6.61, "Horizontal angle"=0.39269908169872414, "Vertical angle"=-0.020943951023931952, "Echo pulse width"=184, "Reserved"=9}, {"flags"=0, "Echo"=0, "Radial distance"=6.74, "Horizontal angle"=0.39269908169872414, "Vertical angle"=-0.006981317007977317, "Echo pulse width"=176, "Reserved"=9}, {"flags"=0, "Echo"=0, "Radial distance"=6.69, "Horizontal angle"=0.3883357585687383, "Vertical angle"=0.00698131700797732, "Echo pulse width"=172, "Reserved"=9}, {"flags"=0, "Echo"=0, "Radial distance"=6.59, "Horizontal angle"=0.3883357585687383, "Vertical angle"=0.020943951023931963, "Echo pulse width"=160, "Reserved"=9}, {"flags"=0, "Echo"=0, "Radial distance"=6.63, "Horizontal angle"=0.3839724354387525, "Vertical angle"=-0.020943951023931952, "Echo pulse width"=216, "Reserved"=9}, {"flags"=0, "Echo"=0, "Radial distance"=6.74, "Horizontal angle"=0.3839724354387525, "Vertical angle"=-0.006981317007977317, "Echo pulse width"=208, "Reserved"=9}, {"flags"=0, "Echo"=0, "Radial distance"=6.84, "Horizontal angle"=0.37960911230876665, "Vertical angle"=0.00698131700797732, "Echo pulse width"=208, "Reserved"=9}, {"flags"=0, "Echo"=0, "Radial distance"=6.640000000000001, "Horizontal angle"=0.37960911230876665, "Vertical angle"=0.020943951023931963, "Echo pulse width"=200, "Reserved"=9}, {"flags"=0, "Echo"=0, "Radial distance"=6.67, "Horizontal angle"=0.3752457891787809, "Vertical angle"=-0.020943951023931952, "Echo pulse width"=180, "Reserved"=9}, {"flags"=0, "Echo"=0, "Radial distance"=6.67, "Horizontal angle"=0.3752457891787809, "Vertical angle"=-0.006981317007977317, "Echo pulse width"=196, "Reserved"=9}, {"flags"=0, "Echo"=0, "Radial distance"=6.69, "Horizontal angle"=0.370882466048795, "Vertical angle"=0.00698131700797732, "Echo pulse width"=172, "Reserved"=9}, {"flags"=0, "Echo"=0, "Radial distance"=6.67, "Horizontal angle"=0.370882466048795, "Vertical angle"=0.020943951023931963, "Echo pulse width"=172, "Reserved"=9}, {"flags"=0, "Echo"=0, "Radial distance"=6.84, "Horizontal angle"=0.3665191429188092, "Vertical angle"=-0.020943951023931952, "Echo pulse width"=236, "Reserved"=9}, {"flags"=0, "Echo"=0, "Radial distance"=6.84, "Horizontal angle"=0.3665191429188092, "Vertical angle"=-0.006981317007977317, "Echo pulse width"=276, "Reserved"=9}, {"flags"=0, "Echo"=0, "Radial distance"=6.95, "Horizontal angle"=0.3621558197888234, "Vertical angle"=0.00698131700797732, "Echo pulse width"=220, "Reserved"=9}, {"flags"=0, "Echo"=0, "Radial distance"=6.76, "Horizontal angle"=0.3621558197888234, "Vertical angle"=0.020943951023931963, "Echo pulse width"=196, "Reserved"=9}, {"flags"=0, "Echo"=0, "Radial distance"=6.87, "Horizontal angle"=0.35779249665883756, "Vertical angle"=-0.020943951023931952, "Echo pulse width"=192, "Reserved"=9}, {"flags"=0, "Echo"=0, "Radial distance"=7.05, "Horizontal angle"=0.35779249665883756, "Vertical angle"=-0.006981317007977317, "Echo pulse width"=236, "Reserved"=9}, {"flags"=0, "Echo"=0, "Radial distance"=6.8100000000000005, "Horizontal angle"=0.3534291735288517, "Vertical angle"=0.00698131700797732, "Echo pulse width"=168, "Reserved"=9}, {"flags"=0, "Echo"=0, "Radial distance"=6.79, "Horizontal angle"=0.3534291735288517, "Vertical angle"=0.020943951023931963, "Echo pulse width"=168, "Reserved"=9}, {"flags"=0, "Echo"=0, "Radial distance"=6.95, "Horizontal angle"=0.3490658503988659, "Vertical angle"=-0.020943951023931952, "Echo pulse width"=192, "Reserved"=9}, {"flags"=0, "Echo"=0, "Radial distance"=7.04, "Horizontal angle"=0.3490658503988659, "Vertical angle"=-0.006981317007977317, "Echo pulse width"=284, "Reserved"=9}, {"flags"=0, "Echo"=0, "Radial distance"=7.07, "Horizontal angle"=0.34470252726888007, "Vertical angle"=0.00698131700797732, "Echo pulse width"=252, "Reserved"=9}, {"flags"=0, "Echo"=0, "Radial distance"=6.98, "Horizontal angle"=0.34470252726888007, "Vertical angle"=0.020943951023931963, "Echo pulse width"=212, "Reserved"=9}, {"flags"=0, "Echo"=0, "Radial distance"=7.11, "Horizontal angle"=0.3403392041388943, "Vertical angle"=-0.020943951023931952, "Echo pulse width"=176, "Reserved"=9}, {"flags"=0, "Echo"=0, "Radial distance"=7.140000000000001, "Horizontal angle"=0.3403392041388943, "Vertical angle"=-0.006981317007977317, "Echo pulse width"=252, "Reserved"=9}, {"flags"=0, "Echo"=0, "Radial distance"=7.0200000000000005, "Horizontal angle"=0.3359758810089084, "Vertical angle"=0.00698131700797732, "Echo pulse width"=196, "Reserved"=9}, {"flags"=0, "Echo"=0, "Radial distance"=6.95, "Horizontal angle"=0.3359758810089084, "Vertical angle"=0.020943951023931963, "Echo pulse width"=176, "Reserved"=9}, {"flags"=0, "Echo"=0, "Radial distance"=7.23, "Horizontal angle"=0.33161255787892263, "Vertical angle"=-0.020943951023931952, "Echo pulse width"=268, "Reserved"=9}, {"flags"=0, "Echo"=0, "Radial distance"=7.28, "Horizontal angle"=0.33161255787892263, "Vertical angle"=-0.006981317007977317, "Echo pulse width"=284, "Reserved"=9}, {"flags"=0, "Echo"=0, "Radial distance"=7.2700000000000005, "Horizontal angle"=0.3272492347489368, "Vertical angle"=0.00698131700797732, "Echo pulse width"=276, "Reserved"=9}, {"flags"=0, "Echo"=0, "Radial distance"=7.16, "Horizontal angle"=0.3272492347489368, "Vertical angle"=0.020943951023931963, "Echo pulse width"=204, "Reserved"=9}, {"flags"=0, "Echo"=0, "Radial distance"=7.59, "Horizontal angle"=0.32288591161895097, "Vertical angle"=-0.020943951023931952, "Echo pulse width"=232, "Reserved"=9}, {"flags"=0, "Echo"=0, "Radial distance"=7.69, "Horizontal angle"=0.32288591161895097, "Vertical angle"=-0.006981317007977317, "Echo pulse width"=232, "Reserved"=9}, {"flags"=0, "Echo"=0, "Radial distance"=7.53, "Horizontal angle"=0.31852258848896514, "Vertical angle"=0.00698131700797732, "Echo pulse width"=172, "Reserved"=9}, {"flags"=0, "Echo"=0, "Radial distance"=7.41, "Horizontal angle"=0.31852258848896514, "Vertical angle"=0.020943951023931963, "Echo pulse width"=184, "Reserved"=9}, {"flags"=0, "Echo"=0, "Radial distance"=7.3500000000000005, "Horizontal angle"=0.3141592653589793, "Vertical angle"=-0.020943951023931952, "Echo pulse width"=300, "Reserved"=9}, {"flags"=0, "Echo"=0, "Radial distance"=7.68, "Horizontal angle"=0.3141592653589793, "Vertical angle"=-0.006981317007977317, "Echo pulse width"=264, "Reserved"=9}, {"flags"=0, "Echo"=0, "Radial distance"=7.58, "Horizontal angle"=0.3097959422289935, "Vertical angle"=0.00698131700797732, "Echo pulse width"=204, "Reserved"=9}, {"flags"=0, "Echo"=0, "Radial distance"=7.48, "Horizontal angle"=0.3097959422289935, "Vertical angle"=0.020943951023931963, "Echo pulse width"=192, "Reserved"=9}, {"flags"=0, "Echo"=0, "Radial distance"=7.47, "Horizontal angle"=0.30543261909900765, "Vertical angle"=-0.020943951023931952, "Echo pulse width"=260, "Reserved"=9}, {"flags"=0, "Echo"=0, "Radial distance"=7.8100000000000005, "Horizontal angle"=0.30543261909900765, "Vertical angle"=-0.006981317007977317, "Echo pulse width"=232, "Reserved"=9}, {"flags"=0, "Echo"=0, "Radial distance"=7.63, "Horizontal angle"=0.3010692959690219, "Vertical angle"=0.00698131700797732, "Echo pulse width"=164, "Reserved"=9}, {"flags"=0, "Echo"=0, "Radial distance"=7.59, "Horizontal angle"=0.3010692959690219, "Vertical angle"=0.020943951023931963, "Echo pulse width"=172, "Reserved"=9}, {"flags"=0, "Echo"=0, "Radial distance"=7.55, "Horizontal angle"=0.296705972839036, "Vertical angle"=-0.020943951023931952, "Echo pulse width"=300, "Reserved"=9}, {"flags"=0, "Echo"=0, "Radial distance"=7.96, "Horizontal angle"=0.296705972839036, "Vertical angle"=-0.006981317007977317, "Echo pulse width"=264, "Reserved"=9}, {"flags"=0, "Echo"=0, "Radial distance"=7.97, "Horizontal angle"=0.2923426497090502, "Vertical angle"=0.00698131700797732, "Echo pulse width"=236, "Reserved"=9}, {"flags"=0, "Echo"=0, "Radial distance"=7.82, "Horizontal angle"=0.2923426497090502, "Vertical angle"=0.020943951023931963, "Echo pulse width"=212, "Reserved"=9}, {"flags"=0, "Echo"=0, "Radial distance"=8.45, "Horizontal angle"=0.28797932657906433, "Vertical angle"=-0.020943951023931952, "Echo pulse width"=204, "Reserved"=9}, {"flags"=0, "Echo"=0, "Radial distance"=8.17, "Horizontal angle"=0.28797932657906433, "Vertical angle"=-0.006981317007977317, "Echo pulse width"=236, "Reserved"=9}, {"flags"=0, "Echo"=0, "Radial distance"=8.15, "Horizontal angle"=0.28361600344907856, "Vertical angle"=0.00698131700797732, "Echo pulse width"=184, "Reserved"=9}, {"flags"=0, "Echo"=0, "Radial distance"=7.95, "Horizontal angle"=0.28361600344907856, "Vertical angle"=0.020943951023931963, "Echo pulse width"=172, "Reserved"=9}, {"flags"=0, "Echo"=0, "Radial distance"=8.56, "Horizontal angle"=0.2792526803190927, "Vertical angle"=-0.020943951023931952, "Echo pulse width"=232, "Reserved"=9}, {"flags"=0, "Echo"=0, "Radial distance"=8.4, "Horizontal angle"=0.2792526803190927, "Vertical angle"=-0.006981317007977317, "Echo pulse width"=264, "Reserved"=9}, {"flags"=0, "Echo"=0, "Radial distance"=8.23, "Horizontal angle"=0.2748893571891069, "Vertical angle"=0.00698131700797732, "Echo pulse width"=192, "Reserved"=9}, {"flags"=0, "Echo"=0, "Radial distance"=8.2, "Horizontal angle"=0.2748893571891069, "Vertical angle"=0.020943951023931963, "Echo pulse width"=192, "Reserved"=9}, {"flags"=0, "Echo"=0, "Radial distance"=8.700000000000001, "Horizontal angle"=0.27052603405912107, "Vertical angle"=-0.020943951023931952, "Echo pulse width"=224, "Reserved"=9}, {"flags"=0, "Echo"=0, "Radial distance"=8.61, "Horizontal angle"=0.27052603405912107, "Vertical angle"=-0.006981317007977317, "Echo pulse width"=220, "Reserved"=9}, {"flags"=0, "Echo"=0, "Radial distance"=8.49, "Horizontal angle"=0.26616271092913524, "Vertical angle"=0.00698131700797732, "Echo pulse width"=176, "Reserved"=9}, {"flags"=0, "Echo"=0, "Radial distance"=8.43, "Horizontal angle"=0.26616271092913524, "Vertical angle"=0.020943951023931963, "Echo pulse width"=176, "Reserved"=9}, {"flags"=0, "Echo"=0, "Radial distance"=8.71, "Horizontal angle"=0.2617993877991494, "Vertical angle"=-0.020943951023931952, "Echo pulse width"=260, "Reserved"=9}, {"flags"=0, "Echo"=0, "Radial distance"=8.700000000000001, "Horizontal angle"=0.2617993877991494, "Vertical angle"=-0.006981317007977317, "Echo pulse width"=248, "Reserved"=9}, {"flags"=0, "Echo"=0, "Radial distance"=8.71, "Horizontal angle"=0.2574360646691636, "Vertical angle"=0.00698131700797732, "Echo pulse width"=196, "Reserved"=9}, {"flags"=0, "Echo"=0, "Radial distance"=8.68, "Horizontal angle"=0.2574360646691636, "Vertical angle"=0.020943951023931963, "Echo pulse width"=216, "Reserved"=9}, {"flags"=0, "Echo"=0, "Radial distance"=9.11, "Horizontal angle"=0.2530727415391778, "Vertical angle"=-0.020943951023931952, "Echo pulse width"=208, "Reserved"=9}, {"flags"=0, "Echo"=0, "Radial distance"=8.94, "Horizontal angle"=0.2530727415391778, "Vertical angle"=-0.006981317007977317, "Echo pulse width"=200, "Reserved"=9}, {"flags"=0, "Echo"=0, "Radial distance"=8.85, "Horizontal angle"=0.24870941840919195, "Vertical angle"=0.00698131700797732, "Echo pulse width"=176, "Reserved"=9}, {"flags"=0, "Echo"=0, "Radial distance"=8.870000000000001, "Horizontal angle"=0.24870941840919195, "Vertical angle"=0.020943951023931963, "Echo pulse width"=172, "Reserved"=9}, {"flags"=0, "Echo"=0, "Radial distance"=9.19, "Horizontal angle"=0.24434609527920614, "Vertical angle"=-0.020943951023931952, "Echo pulse width"=256, "Reserved"=9}, {"flags"=0, "Echo"=0, "Radial distance"=9.36, "Horizontal angle"=0.24434609527920614, "Vertical angle"=-0.006981317007977317, "Echo pulse width"=280, "Reserved"=9}, {"flags"=0, "Echo"=0, "Radial distance"=9.24, "Horizontal angle"=0.2399827721492203, "Vertical angle"=0.00698131700797732, "Echo pulse width"=208, "Reserved"=9}, {"flags"=0, "Echo"=0, "Radial distance"=9.200000000000001, "Horizontal angle"=0.2399827721492203, "Vertical angle"=0.020943951023931963, "Echo pulse width"=204, "Reserved"=9}, {"flags"=0, "Echo"=0, "Radial distance"=9.42, "Horizontal angle"=0.23561944901923448, "Vertical angle"=-0.020943951023931952, "Echo pulse width"=224, "Reserved"=9}, {"flags"=0, "Echo"=0, "Radial distance"=9.59, "Horizontal angle"=0.23561944901923448, "Vertical angle"=-0.006981317007977317, "Echo pulse width"=264, "Reserved"=9}, {"flags"=0, "Echo"=0, "Radial distance"=9.49, "Horizontal angle"=0.23125612588924865, "Vertical angle"=0.00698131700797732, "Echo pulse width"=176, "Reserved"=9}, {"flags"=0, "Echo"=0, "Radial distance"=9.35, "Horizontal angle"=0.23125612588924865, "Vertical angle"=0.020943951023931963, "Echo pulse width"=172, "Reserved"=9}, {"flags"=0, "Echo"=0, "Radial distance"=9.67, "Horizontal angle"=0.22689280275926282, "Vertical angle"=-0.020943951023931952, "Echo pulse width"=260, "Reserved"=9}, {"flags"=0, "Echo"=0, "Radial distance"=10.0, "Horizontal angle"=0.22689280275926282, "Vertical angle"=-0.006981317007977317, "Echo pulse width"=284, "Reserved"=9}, {"flags"=0, "Echo"=0, "Radial distance"=9.91, "Horizontal angle"=0.222529479629277, "Vertical angle"=0.00698131700797732, "Echo pulse width"=248, "Reserved"=9}, {"flags"=0, "Echo"=0, "Radial distance"=9.76, "Horizontal angle"=0.222529479629277, "Vertical angle"=0.020943951023931963, "Echo pulse width"=204, "Reserved"=9}, {"flags"=0, "Echo"=0, "Radial distance"=10.02, "Horizontal angle"=0.2181661564992912, "Vertical angle"=-0.020943951023931952, "Echo pulse width"=228, "Reserved"=9}, {"flags"=0, "Echo"=0, "Radial distance"=10.35, "Horizontal angle"=0.2181661564992912, "Vertical angle"=-0.006981317007977317, "Echo pulse width"=264, "Reserved"=9}, {"flags"=0, "Echo"=0, "Radial distance"=10.17, "Horizontal angle"=0.21380283336930533, "Vertical angle"=0.00698131700797732, "Echo pulse width"=180, "Reserved"=9}, {"flags"=0, "Echo"=0, "Radial distance"=10.07, "Horizontal angle"=0.21380283336930533, "Vertical angle"=0.020943951023931963, "Echo pulse width"=176, "Reserved"=9}, {"flags"=0, "Echo"=0, "Radial distance"=9.950000000000001, "Horizontal angle"=0.20943951023931953, "Vertical angle"=-0.020943951023931952, "Echo pulse width"=288, "Reserved"=9}, {"flags"=0, "Echo"=0, "Radial distance"=10.4, "Horizontal angle"=0.20943951023931953, "Vertical angle"=-0.006981317007977317, "Echo pulse width"=316, "Reserved"=9}, {"flags"=0, "Echo"=0, "Radial distance"=10.55, "Horizontal angle"=0.20507618710933373, "Vertical angle"=0.00698131700797732, "Echo pulse width"=268, "Reserved"=9}, {"flags"=0, "Echo"=0, "Radial distance"=10.32, "Horizontal angle"=0.20507618710933373, "Vertical angle"=0.020943951023931963, "Echo pulse width"=204, "Reserved"=9}, {"flags"=0, "Echo"=0, "Radial distance"=10.44, "Horizontal angle"=0.20071286397934787, "Vertical angle"=-0.020943951023931952, "Echo pulse width"=216, "Reserved"=9}, {"flags"=0, "Echo"=0, "Radial distance"=10.75, "Horizontal angle"=0.20071286397934787, "Vertical angle"=-0.006981317007977317, "Echo pulse width"=280, "Reserved"=9}, {"flags"=0, "Echo"=0, "Radial distance"=10.85, "Horizontal angle"=0.19634954084936207, "Vertical angle"=0.00698131700797732, "Echo pulse width"=176, "Reserved"=9}, {"flags"=0, "Echo"=0, "Radial distance"=10.8, "Horizontal angle"=0.19634954084936207, "Vertical angle"=0.020943951023931963, "Echo pulse width"=192, "Reserved"=9}, {"flags"=4, "Echo"=0, "Radial distance"=10.11, "Horizontal angle"=0.19198621771937624, "Vertical angle"=-0.020943951023931952, "Echo pulse width"=324, "Reserved"=0}, {"flags"=0, "Echo"=0, "Radial distance"=11.28, "Horizontal angle"=0.19198621771937624, "Vertical angle"=-0.006981317007977317, "Echo pulse width"=260, "Reserved"=9}, {"flags"=0, "Echo"=0, "Radial distance"=11.23, "Horizontal angle"=0.18762289458939044, "Vertical angle"=0.00698131700797732, "Echo pulse width"=220, "Reserved"=9}, {"flags"=0, "Echo"=0, "Radial distance"=11.120000000000001, "Horizontal angle"=0.18762289458939044, "Vertical angle"=0.020943951023931963, "Echo pulse width"=200, "Reserved"=9}, {"flags"=4, "Echo"=0, "Radial distance"=10.43, "Horizontal angle"=0.1832595714594046, "Vertical angle"=-0.020943951023931952, "Echo pulse width"=296, "Reserved"=0}, {"flags"=0, "Echo"=0, "Radial distance"=11.39, "Horizontal angle"=0.1832595714594046, "Vertical angle"=-0.006981317007977317, "Echo pulse width"=260, "Reserved"=9}, {"flags"=0, "Echo"=0, "Radial distance"=11.370000000000001, "Horizontal angle"=0.17889624832941878, "Vertical angle"=0.00698131700797732, "Echo pulse width"=172, "Reserved"=9}, {"flags"=0, "Echo"=0, "Radial distance"=11.51, "Horizontal angle"=0.17889624832941878, "Vertical angle"=0.020943951023931963, "Echo pulse width"=176, "Reserved"=9}, {"flags"=4, "Echo"=0, "Radial distance"=10.49, "Horizontal angle"=0.17453292519943295, "Vertical angle"=-0.020943951023931952, "Echo pulse width"=372, "Reserved"=0}, {"flags"=0, "Echo"=0, "Radial distance"=11.92, "Horizontal angle"=0.17453292519943295, "Vertical angle"=-0.006981317007977317, "Echo pulse width"=296, "Reserved"=9}, {"flags"=0, "Echo"=0, "Radial distance"=11.88, "Horizontal angle"=0.17016960206944715, "Vertical angle"=0.00698131700797732, "Echo pulse width"=208, "Reserved"=9}, {"flags"=0, "Echo"=0, "Radial distance"=12.040000000000001, "Horizontal angle"=0.17016960206944715, "Vertical angle"=0.020943951023931963, "Echo pulse width"=216, "Reserved"=9}, {"flags"=4, "Echo"=0, "Radial distance"=10.950000000000001, "Horizontal angle"=0.16580627893946132, "Vertical angle"=-0.020943951023931952, "Echo pulse width"=308, "Reserved"=0}, {"flags"=0, "Echo"=0, "Radial distance"=12.5, "Horizontal angle"=0.16580627893946132, "Vertical angle"=-0.006981317007977317, "Echo pulse width"=200, "Reserved"=9}, {"flags"=0, "Echo"=0, "Radial distance"=12.41, "Horizontal angle"=0.16144295580947549, "Vertical angle"=0.00698131700797732, "Echo pulse width"=172, "Reserved"=9}, {"flags"=0, "Echo"=0, "Radial distance"=12.71, "Horizontal angle"=0.16144295580947549, "Vertical angle"=0.020943951023931963, "Echo pulse width"=180, "Reserved"=9}, {"flags"=4, "Echo"=0, "Radial distance"=11.27, "Horizontal angle"=0.15707963267948966, "Vertical angle"=-0.020943951023931952, "Echo pulse width"=312, "Reserved"=0}, {"flags"=4, "Echo"=0, "Radial distance"=13.26, "Horizontal angle"=0.15707963267948966, "Vertical angle"=-0.006981317007977317, "Echo pulse width"=244, "Reserved"=0}, {"flags"=2, "Echo"=0, "Radial distance"=13.08, "Horizontal angle"=0.15271630954950383, "Vertical angle"=0.00698131700797732, "Echo pulse width"=212, "Reserved"=0}, {"flags"=3, "Echo"=0, "Radial distance"=13.27, "Horizontal angle"=0.15271630954950383, "Vertical angle"=0.020943951023931963, "Echo pulse width"=156, "Reserved"=0}, {"flags"=0, "Echo"=1, "Radial distance"=19.92, "Horizontal angle"=0.15271630954950383, "Vertical angle"=0.020943951023931963, "Echo pulse width"=176, "Reserved"=10}, {"flags"=4, "Echo"=0, "Radial distance"=11.790000000000001, "Horizontal angle"=0.148352986419518, "Vertical angle"=-0.020943951023931952, "Echo pulse width"=264, "Reserved"=0}, {"flags"=5, "Echo"=0, "Radial distance"=13.88, "Horizontal angle"=0.148352986419518, "Vertical angle"=-0.006981317007977317, "Echo pulse width"=168, "Reserved"=0}, {"flags"=5, "Echo"=1, "Radial distance"=15.94, "Horizontal angle"=0.148352986419518, "Vertical angle"=-0.006981317007977317, "Echo pulse width"=108, "Reserved"=0}, {"flags"=4, "Echo"=2, "Radial distance"=18.05, "Horizontal angle"=0.148352986419518, "Vertical angle"=-0.006981317007977317, "Echo pulse width"=340, "Reserved"=0}, {"flags"=0, "Echo"=0, "Radial distance"=19.580000000000002, "Horizontal angle"=0.14398966328953217, "Vertical angle"=0.00698131700797732, "Echo pulse width"=204, "Reserved"=10}, {"flags"=0, "Echo"=0, "Radial distance"=19.73, "Horizontal angle"=0.14398966328953217, "Vertical angle"=0.020943951023931963, "Echo pulse width"=188, "Reserved"=10}, {"flags"=4, "Echo"=0, "Radial distance"=12.19, "Horizontal angle"=0.13962634015954636, "Vertical angle"=-0.020943951023931952, "Echo pulse width"=296, "Reserved"=0}, {"flags"=3, "Echo"=0, "Radial distance"=13.52, "Horizontal angle"=0.13962634015954636, "Vertical angle"=-0.006981317007977317, "Echo pulse width"=128, "Reserved"=0}, {"flags"=5, "Echo"=1, "Radial distance"=15.610000000000001, "Horizontal angle"=0.13962634015954636, "Vertical angle"=-0.006981317007977317, "Echo pulse width"=392, "Reserved"=0}, {"flags"=0, "Echo"=2, "Radial distance"=19.61, "Horizontal angle"=0.13962634015954636, "Vertical angle"=-0.006981317007977317, "Echo pulse width"=148, "Reserved"=10}, {"flags"=0, "Echo"=0, "Radial distance"=19.56, "Horizontal angle"=0.13526301702956053, "Vertical angle"=0.00698131700797732, "Echo pulse width"=208, "Reserved"=10}, {"flags"=0, "Echo"=0, "Radial distance"=19.76, "Horizontal angle"=0.13526301702956053, "Vertical angle"=0.020943951023931963, "Echo pulse width"=192, "Reserved"=10}, {"flags"=4, "Echo"=0, "Radial distance"=12.83, "Horizontal angle"=0.1308996938995747, "Vertical angle"=-0.020943951023931952, "Echo pulse width"=288, "Reserved"=0}, {"flags"=5, "Echo"=0, "Radial distance"=14.97, "Horizontal angle"=0.1308996938995747, "Vertical angle"=-0.006981317007977317, "Echo pulse width"=400, "Reserved"=0}, {"flags"=0, "Echo"=1, "Radial distance"=19.35, "Horizontal angle"=0.1308996938995747, "Vertical angle"=-0.006981317007977317, "Echo pulse width"=204, "Reserved"=10}, {"flags"=0, "Echo"=0, "Radial distance"=19.59, "Horizontal angle"=0.1265363707695889, "Vertical angle"=0.00698131700797732, "Echo pulse width"=196, "Reserved"=10}, {"flags"=0, "Echo"=0, "Radial distance"=19.8, "Horizontal angle"=0.1265363707695889, "Vertical angle"=0.020943951023931963, "Echo pulse width"=200, "Reserved"=10}, {"flags"=4, "Echo"=0, "Radial distance"=13.39, "Horizontal angle"=0.12217304763960307, "Vertical angle"=-0.020943951023931952, "Echo pulse width"=292, "Reserved"=0}, {"flags"=5, "Echo"=0, "Radial distance"=15.700000000000001, "Horizontal angle"=0.12217304763960307, "Vertical angle"=-0.006981317007977317, "Echo pulse width"=172, "Reserved"=0}, {"flags"=4, "Echo"=1, "Radial distance"=17.69, "Horizontal angle"=0.12217304763960307, "Vertical angle"=-0.006981317007977317, "Echo pulse width"=380, "Reserved"=0}, {"flags"=0, "Echo"=0, "Radial distance"=19.75, "Horizontal angle"=0.11780972450961724, "Vertical angle"=0.00698131700797732, "Echo pulse width"=216, "Reserved"=10}, {"flags"=0, "Echo"=0, "Radial distance"=19.84, "Horizontal angle"=0.11780972450961724, "Vertical angle"=0.020943951023931963, "Echo pulse width"=200, "Reserved"=10}, {"flags"=5, "Echo"=0, "Radial distance"=13.99, "Horizontal angle"=0.11344640137963141, "Vertical angle"=-0.020943951023931952, "Echo pulse width"=152, "Reserved"=0}, {"flags"=4, "Echo"=1, "Radial distance"=15.35, "Horizontal angle"=0.11344640137963141, "Vertical angle"=-0.020943951023931952, "Echo pulse width"=120, "Reserved"=0}, {"flags"=4, "Echo"=0, "Radial distance"=16.45, "Horizontal angle"=0.11344640137963141, "Vertical angle"=-0.006981317007977317, "Echo pulse width"=500, "Reserved"=0}, {"flags"=0, "Echo"=0, "Radial distance"=19.71, "Horizontal angle"=0.1090830782496456, "Vertical angle"=0.00698131700797732, "Echo pulse width"=196, "Reserved"=10}, {"flags"=0, "Echo"=0, "Radial distance"=20.0, "Horizontal angle"=0.1090830782496456, "Vertical angle"=0.020943951023931963, "Echo pulse width"=200, "Reserved"=10}, {"flags"=4, "Echo"=0, "Radial distance"=14.72, "Horizontal angle"=0.10471975511965977, "Vertical angle"=-0.020943951023931952, "Echo pulse width"=172, "Reserved"=0}, {"flags"=4, "Echo"=0, "Radial distance"=17.25, "Horizontal angle"=0.10471975511965977, "Vertical angle"=-0.006981317007977317, "Echo pulse width"=420, "Reserved"=0}, {"flags"=0, "Echo"=0, "Radial distance"=19.72, "Horizontal angle"=0.10035643198967394, "Vertical angle"=0.00698131700797732, "Echo pulse width"=188, "Reserved"=10}, {"flags"=1, "Echo"=0, "Radial distance"=20.2, "Horizontal angle"=0.10035643198967394, "Vertical angle"=0.020943951023931963, "Echo pulse width"=204, "Reserved"=10}, {"flags"=0, "Echo"=1, "Radial distance"=22.21, "Horizontal angle"=0.10035643198967394, "Vertical angle"=0.020943951023931963, "Echo pulse width"=20, "Reserved"=11}, {"flags"=4, "Echo"=0, "Radial distance"=15.6, "Horizontal angle"=0.09599310885968812, "Vertical angle"=-0.020943951023931952, "Echo pulse width"=172, "Reserved"=0}, {"flags"=5, "Echo"=0, "Radial distance"=17.62, "Horizontal angle"=0.09599310885968812, "Vertical angle"=-0.006981317007977317, "Echo pulse width"=164, "Reserved"=0}, {"flags"=0, "Echo"=1, "Radial distance"=19.82, "Horizontal angle"=0.09599310885968812, "Vertical angle"=-0.006981317007977317, "Echo pulse width"=208, "Reserved"=10}, {"flags"=0, "Echo"=0, "Radial distance"=19.91, "Horizontal angle"=0.0916297857297023, "Vertical angle"=0.00698131700797732, "Echo pulse width"=192, "Reserved"=10}, {"flags"=0, "Echo"=0, "Radial distance"=20.52, "Horizontal angle"=0.0916297857297023, "Vertical angle"=0.020943951023931963, "Echo pulse width"=204, "Reserved"=10}, {"flags"=4, "Echo"=0, "Radial distance"=16.31, "Horizontal angle"=0.08726646259971647, "Vertical angle"=-0.020943951023931952, "Echo pulse width"=224, "Reserved"=0}, {"flags"=4, "Echo"=0, "Radial distance"=18.650000000000002, "Horizontal angle"=0.08726646259971647, "Vertical angle"=-0.006981317007977317, "Echo pulse width"=368, "Reserved"=0}, {"flags"=4, "Echo"=0, "Radial distance"=20.92, "Horizontal angle"=0.08290313946973066, "Vertical angle"=0.00698131700797732, "Echo pulse width"=184, "Reserved"=0}, {"flags"=4, "Echo"=0, "Radial distance"=21.46, "Horizontal angle"=0.08290313946973066, "Vertical angle"=0.020943951023931963, "Echo pulse width"=212, "Reserved"=0}, {"flags"=4, "Echo"=0, "Radial distance"=15.290000000000001, "Horizontal angle"=0.07853981633974483, "Vertical angle"=-0.020943951023931952, "Echo pulse width"=436, "Reserved"=0}, {"flags"=4, "Echo"=0, "Radial distance"=18.61, "Horizontal angle"=0.07853981633974483, "Vertical angle"=-0.006981317007977317, "Echo pulse width"=508, "Reserved"=0}, {"flags"=4, "Echo"=0, "Radial distance"=22.12, "Horizontal angle"=0.074176493209759, "Vertical angle"=0.00698131700797732, "Echo pulse width"=188, "Reserved"=0}, {"flags"=4, "Echo"=0, "Radial distance"=22.64, "Horizontal angle"=0.074176493209759, "Vertical angle"=0.020943951023931963, "Echo pulse width"=220, "Reserved"=0}, {"flags"=5, "Echo"=0, "Radial distance"=15.76, "Horizontal angle"=0.06981317007977318, "Vertical angle"=-0.020943951023931952, "Echo pulse width"=232, "Reserved"=0}, {"flags"=4, "Echo"=1, "Radial distance"=18.98, "Horizontal angle"=0.06981317007977318, "Vertical angle"=-0.020943951023931952, "Echo pulse width"=156, "Reserved"=0}, {"flags"=5, "Echo"=0, "Radial distance"=19.32, "Horizontal angle"=0.06981317007977318, "Vertical angle"=-0.006981317007977317, "Echo pulse width"=128, "Reserved"=0}, {"flags"=4, "Echo"=1, "Radial distance"=21.68, "Horizontal angle"=0.06981317007977318, "Vertical angle"=-0.006981317007977317, "Echo pulse width"=292, "Reserved"=0}, {"flags"=4, "Echo"=0, "Radial distance"=23.46, "Horizontal angle"=0.06544984694978735, "Vertical angle"=0.00698131700797732, "Echo pulse width"=200, "Reserved"=0}, {"flags"=4, "Echo"=0, "Radial distance"=24.44, "Horizontal angle"=0.06544984694978735, "Vertical angle"=0.020943951023931963, "Echo pulse width"=180, "Reserved"=0}, {"flags"=5, "Echo"=0, "Radial distance"=16.88, "Horizontal angle"=0.061086523819801536, "Vertical angle"=-0.020943951023931952, "Echo pulse width"=236, "Reserved"=0}, {"flags"=0, "Echo"=1, "Radial distance"=20.56, "Horizontal angle"=0.061086523819801536, "Vertical angle"=-0.020943951023931952, "Echo pulse width"=132, "Reserved"=10}, {"flags"=1, "Echo"=0, "Radial distance"=20.75, "Horizontal angle"=0.061086523819801536, "Vertical angle"=-0.006981317007977317, "Echo pulse width"=124, "Reserved"=10}, {"flags"=5, "Echo"=1, "Radial distance"=22.91, "Horizontal angle"=0.061086523819801536, "Vertical angle"=-0.006981317007977317, "Echo pulse width"=200, "Reserved"=0}, {"flags"=0, "Echo"=2, "Radial distance"=24.85, "Horizontal angle"=0.061086523819801536, "Vertical angle"=-0.006981317007977317, "Echo pulse width"=156, "Reserved"=12}, {"flags"=0, "Echo"=0, "Radial distance"=25.14, "Horizontal angle"=0.056723200689815706, "Vertical angle"=0.00698131700797732, "Echo pulse width"=204, "Reserved"=12}, {"flags"=0, "Echo"=0, "Radial distance"=26.37, "Horizontal angle"=0.056723200689815706, "Vertical angle"=0.020943951023931963, "Echo pulse width"=64, "Reserved"=13}, {"flags"=5, "Echo"=0, "Radial distance"=18.31, "Horizontal angle"=0.05235987755982988, "Vertical angle"=-0.020943951023931952, "Echo pulse width"=248, "Reserved"=0}, {"flags"=0, "Echo"=1, "Radial distance"=22.41, "Horizontal angle"=0.05235987755982988, "Vertical angle"=-0.020943951023931952, "Echo pulse width"=84, "Reserved"=14}, {"flags"=1, "Echo"=0, "Radial distance"=22.6, "Horizontal angle"=0.05235987755982988, "Vertical angle"=-0.006981317007977317, "Echo pulse width"=136, "Reserved"=14}, {"flags"=1, "Echo"=1, "Radial distance"=24.97, "Horizontal angle"=0.05235987755982988, "Vertical angle"=-0.006981317007977317, "Echo pulse width"=144, "Reserved"=12}, {"flags"=0, "Echo"=2, "Radial distance"=26.560000000000002, "Horizontal angle"=0.05235987755982988, "Vertical angle"=-0.006981317007977317, "Echo pulse width"=128, "Reserved"=13}, {"flags"=4, "Echo"=0, "Radial distance"=32.79, "Horizontal angle"=0.04799655442984406, "Vertical angle"=0.00698131700797732, "Echo pulse width"=176, "Reserved"=0}, {"flags"=4, "Echo"=0, "Radial distance"=20.11, "Horizontal angle"=0.04363323129985824, "Vertical angle"=-0.020943951023931952, "Echo pulse width"=264, "Reserved"=0}, {"flags"=5, "Echo"=0, "Radial distance"=24.76, "Horizontal angle"=0.04363323129985824, "Vertical angle"=-0.006981317007977317, "Echo pulse width"=132, "Reserved"=0}, {"flags"=5, "Echo"=1, "Radial distance"=28.05, "Horizontal angle"=0.04363323129985824, "Vertical angle"=-0.006981317007977317, "Echo pulse width"=224, "Reserved"=0}, {"flags"=4, "Echo"=2, "Radial distance"=31.12, "Horizontal angle"=0.04363323129985824, "Vertical angle"=-0.006981317007977317, "Echo pulse width"=92, "Reserved"=0}, {"flags"=4, "Echo"=0, "Radial distance"=32.99, "Horizontal angle"=0.039269908169872414, "Vertical angle"=0.00698131700797732, "Echo pulse width"=180, "Reserved"=0}, {"flags"=4, "Echo"=0, "Radial distance"=22.52, "Horizontal angle"=0.03490658503988659, "Vertical angle"=-0.020943951023931952, "Echo pulse width"=236, "Reserved"=0}, {"flags"=5, "Echo"=0, "Radial distance"=27.490000000000002, "Horizontal angle"=0.03490658503988659, "Vertical angle"=-0.006981317007977317, "Echo pulse width"=144, "Reserved"=0}, {"flags"=4, "Echo"=1, "Radial distance"=31.14, "Horizontal angle"=0.03490658503988659, "Vertical angle"=-0.006981317007977317, "Echo pulse width"=208, "Reserved"=0}, {"flags"=0, "Echo"=0, "Radial distance"=33.94, "Horizontal angle"=0.030543261909900768, "Vertical angle"=0.00698131700797732, "Echo pulse width"=200, "Reserved"=15}, {"flags"=4, "Echo"=0, "Radial distance"=24.73, "Horizontal angle"=0.02617993877991494, "Vertical angle"=-0.020943951023931952, "Echo pulse width"=80, "Reserved"=0}, {"flags"=5, "Echo"=0, "Radial distance"=30.580000000000002, "Horizontal angle"=0.02617993877991494, "Vertical angle"=-0.006981317007977317, "Echo pulse width"=168, "Reserved"=0}, {"flags"=1, "Echo"=1, "Radial distance"=34.27, "Horizontal angle"=0.02617993877991494, "Vertical angle"=-0.006981317007977317, "Echo pulse width"=112, "Reserved"=15}, {"flags"=4, "Echo"=2, "Radial distance"=36.050000000000004, "Horizontal angle"=0.02617993877991494, "Vertical angle"=-0.006981317007977317, "Echo pulse width"=76, "Reserved"=0}, {"flags"=4, "Echo"=0, "Radial distance"=37.57, "Horizontal angle"=0.02181661564992912, "Vertical angle"=0.00698131700797732, "Echo pulse width"=236, "Reserved"=0}, {"flags"=5, "Echo"=0, "Radial distance"=29.080000000000002, "Horizontal angle"=0.017453292519943295, "Vertical angle"=-0.006981317007977317, "Echo pulse width"=192, "Reserved"=0}, {"flags"=5, "Echo"=1, "Radial distance"=34.93, "Horizontal angle"=0.017453292519943295, "Vertical angle"=-0.006981317007977317, "Echo pulse width"=100, "Reserved"=0}, {"flags"=4, "Echo"=2, "Radial distance"=38.480000000000004, "Horizontal angle"=0.017453292519943295, "Vertical angle"=-0.006981317007977317, "Echo pulse width"=132, "Reserved"=0}, {"flags"=0, "Echo"=0, "Radial distance"=54.64, "Horizontal angle"=0.01308996938995747, "Vertical angle"=0.00698131700797732, "Echo pulse width"=188, "Reserved"=16}, {"flags"=0, "Echo"=0, "Radial distance"=54.18, "Horizontal angle"=0.01308996938995747, "Vertical angle"=0.020943951023931963, "Echo pulse width"=92, "Reserved"=16}, {"flags"=5, "Echo"=0, "Radial distance"=32.88, "Horizontal angle"=0.008726646259971648, "Vertical angle"=-0.006981317007977317, "Echo pulse width"=192, "Reserved"=0}, {"flags"=5, "Echo"=1, "Radial distance"=34.25, "Horizontal angle"=0.008726646259971648, "Vertical angle"=-0.006981317007977317, "Echo pulse width"=76, "Reserved"=0}, {"flags"=4, "Echo"=2, "Radial distance"=40.58, "Horizontal angle"=0.008726646259971648, "Vertical angle"=-0.006981317007977317, "Echo pulse width"=104, "Reserved"=0}, {"flags"=4, "Echo"=0, "Radial distance"=22.93, "Horizontal angle"=0.0, "Vertical angle"=-0.020943951023931952, "Echo pulse width"=84, "Reserved"=0}, {"flags"=4, "Echo"=0, "Radial distance"=22.61, "Horizontal angle"=-0.008726646259971648, "Vertical angle"=-0.020943951023931952, "Echo pulse width"=208, "Reserved"=0}, {"flags"=0, "Echo"=0, "Radial distance"=71.72, "Horizontal angle"=-0.01308996938995747, "Vertical angle"=0.00698131700797732, "Echo pulse width"=144, "Reserved"=17}, {"flags"=5, "Echo"=0, "Radial distance"=21.75, "Horizontal angle"=-0.017453292519943295, "Vertical angle"=-0.020943951023931952, "Echo pulse width"=188, "Reserved"=0}, {"flags"=4, "Echo"=1, "Radial distance"=23.55, "Horizontal angle"=-0.017453292519943295, "Vertical angle"=-0.020943951023931952, "Echo pulse width"=120, "Reserved"=0}, {"flags"=0, "Echo"=0, "Radial distance"=71.49, "Horizontal angle"=-0.017453292519943295, "Vertical angle"=-0.006981317007977317, "Echo pulse width"=52, "Reserved"=17}, {"flags"=5, "Echo"=0, "Radial distance"=21.03, "Horizontal angle"=-0.02617993877991494, "Vertical angle"=-0.020943951023931952, "Echo pulse width"=184, "Reserved"=0}, {"flags"=4, "Echo"=1, "Radial distance"=24.19, "Horizontal angle"=-0.02617993877991494, "Vertical angle"=-0.020943951023931952, "Echo pulse width"=112, "Reserved"=0}, {"flags"=0, "Echo"=0, "Radial distance"=58.050000000000004, "Horizontal angle"=-0.02617993877991494, "Vertical angle"=-0.006981317007977317, "Echo pulse width"=48, "Reserved"=18}, {"flags"=5, "Echo"=0, "Radial distance"=21.240000000000002, "Horizontal angle"=-0.03490658503988659, "Vertical angle"=-0.020943951023931952, "Echo pulse width"=168, "Reserved"=0}, {"flags"=4, "Echo"=1, "Radial distance"=24.47, "Horizontal angle"=-0.03490658503988659, "Vertical angle"=-0.020943951023931952, "Echo pulse width"=116, "Reserved"=0}, {"flags"=5, "Echo"=0, "Radial distance"=21.830000000000002, "Horizontal angle"=-0.04363323129985824, "Vertical angle"=-0.020943951023931952, "Echo pulse width"=164, "Reserved"=0}, {"flags"=4, "Echo"=1, "Radial distance"=23.71, "Horizontal angle"=-0.04363323129985824, "Vertical angle"=-0.020943951023931952, "Echo pulse width"=116, "Reserved"=0}, {"flags"=4, "Echo"=0, "Radial distance"=22.650000000000002, "Horizontal angle"=-0.05235987755982988, "Vertical angle"=-0.020943951023931952, "Echo pulse width"=212, "Reserved"=0}, {"flags"=0, "Echo"=0, "Radial distance"=229.02, "Horizontal angle"=-0.06544984694978735, "Vertical angle"=0.00698131700797732, "Echo pulse width"=128, "Reserved"=19}, {"flags"=0, "Echo"=0, "Radial distance"=188.3, "Horizontal angle"=-0.06544984694978735, "Vertical angle"=0.020943951023931963, "Echo pulse width"=144, "Reserved"=20}, {"flags"=1, "Echo"=0, "Radial distance"=38.07, "Horizontal angle"=-0.06981317007977318, "Vertical angle"=-0.006981317007977317, "Echo pulse width"=204, "Reserved"=21}, {"flags"=1, "Echo"=1, "Radial distance"=39.56, "Horizontal angle"=-0.06981317007977318, "Vertical angle"=-0.006981317007977317, "Echo pulse width"=88, "Reserved"=22}, {"flags"=0, "Echo"=2, "Radial distance"=57.84, "Horizontal angle"=-0.06981317007977318, "Vertical angle"=-0.006981317007977317, "Echo pulse width"=36, "Reserved"=23}, {"flags"=4, "Echo"=0, "Radial distance"=30.03, "Horizontal angle"=-0.07853981633974483, "Vertical angle"=-0.006981317007977317, "Echo pulse width"=200, "Reserved"=0}, {"flags"=4, "Echo"=0, "Radial distance"=21.91, "Horizontal angle"=-0.08726646259971647, "Vertical angle"=-0.020943951023931952, "Echo pulse width"=340, "Reserved"=0}, {"flags"=0, "Echo"=0, "Radial distance"=58.21, "Horizontal angle"=-0.08726646259971647, "Vertical angle"=-0.006981317007977317, "Echo pulse width"=52, "Reserved"=24}, {"flags"=0, "Echo"=0, "Radial distance"=88.99, "Horizontal angle"=-0.10035643198967394, "Vertical angle"=0.00698131700797732, "Echo pulse width"=76, "Reserved"=25}, {"flags"=4, "Echo"=0, "Radial distance"=15.52, "Horizontal angle"=-0.10471975511965977, "Vertical angle"=-0.020943951023931952, "Echo pulse width"=236, "Reserved"=0}, {"flags"=0, "Echo"=0, "Radial distance"=89.03, "Horizontal angle"=-0.1090830782496456, "Vertical angle"=0.00698131700797732, "Echo pulse width"=140, "Reserved"=25}, {"flags"=4, "Echo"=0, "Radial distance"=14.870000000000001, "Horizontal angle"=-0.11344640137963141, "Vertical angle"=-0.020943951023931952, "Echo pulse width"=76, "Reserved"=0}, {"flags"=0, "Echo"=0, "Radial distance"=287.03000000000003, "Horizontal angle"=-0.11780972450961724, "Vertical angle"=0.00698131700797732, "Echo pulse width"=140, "Reserved"=26}, {"flags"=4, "Echo"=0, "Radial distance"=22.91, "Horizontal angle"=-0.12217304763960307, "Vertical angle"=-0.020943951023931952, "Echo pulse width"=116, "Reserved"=0}, {"flags"=0, "Echo"=0, "Radial distance"=69.89, "Horizontal angle"=-0.1265363707695889, "Vertical angle"=0.020943951023931963, "Echo pulse width"=132, "Reserved"=27}, {"flags"=4, "Echo"=0, "Radial distance"=22.91, "Horizontal angle"=-0.1308996938995747, "Vertical angle"=-0.020943951023931952, "Echo pulse width"=252, "Reserved"=0}, {"flags"=0, "Echo"=0, "Radial distance"=153.20000000000002, "Horizontal angle"=-0.13526301702956053, "Vertical angle"=0.020943951023931963, "Echo pulse width"=48, "Reserved"=28}, {"flags"=5, "Echo"=0, "Radial distance"=22.1, "Horizontal angle"=-0.13962634015954636, "Vertical angle"=-0.020943951023931952, "Echo pulse width"=156, "Reserved"=0}, {"flags"=4, "Echo"=1, "Radial distance"=24.42, "Horizontal angle"=-0.13962634015954636, "Vertical angle"=-0.020943951023931952, "Echo pulse width"=152, "Reserved"=0}, {"flags"=4, "Echo"=0, "Radial distance"=47.07, "Horizontal angle"=-0.13962634015954636, "Vertical angle"=-0.006981317007977317, "Echo pulse width"=40, "Reserved"=0}, {"flags"=5, "Echo"=0, "Radial distance"=21.6, "Horizontal angle"=-0.148352986419518, "Vertical angle"=-0.020943951023931952, "Echo pulse width"=172, "Reserved"=0}, {"flags"=4, "Echo"=1, "Radial distance"=24.560000000000002, "Horizontal angle"=-0.148352986419518, "Vertical angle"=-0.020943951023931952, "Echo pulse width"=88, "Reserved"=0}, {"flags"=4, "Echo"=0, "Radial distance"=42.27, "Horizontal angle"=-0.148352986419518, "Vertical angle"=-0.006981317007977317, "Echo pulse width"=84, "Reserved"=0}, {"flags"=0, "Echo"=0, "Radial distance"=96.75, "Horizontal angle"=-0.15271630954950383, "Vertical angle"=0.00698131700797732, "Echo pulse width"=136, "Reserved"=29}, {"flags"=5, "Echo"=0, "Radial distance"=21.12, "Horizontal angle"=-0.15707963267948966, "Vertical angle"=-0.020943951023931952, "Echo pulse width"=176, "Reserved"=0}, {"flags"=4, "Echo"=1, "Radial distance"=24.02, "Horizontal angle"=-0.15707963267948966, "Vertical angle"=-0.020943951023931952, "Echo pulse width"=96, "Reserved"=0}, {"flags"=4, "Echo"=0, "Radial distance"=38.67, "Horizontal angle"=-0.15707963267948966, "Vertical angle"=-0.006981317007977317, "Echo pulse width"=120, "Reserved"=0}, {"flags"=0, "Echo"=0, "Radial distance"=84.31, "Horizontal angle"=-0.16144295580947549, "Vertical angle"=0.00698131700797732, "Echo pulse width"=104, "Reserved"=30}, {"flags"=5, "Echo"=0, "Radial distance"=21.52, "Horizontal angle"=-0.16580627893946132, "Vertical angle"=-0.020943951023931952, "Echo pulse width"=232, "Reserved"=0}, {"flags"=4, "Echo"=1, "Radial distance"=23.6, "Horizontal angle"=-0.16580627893946132, "Vertical angle"=-0.020943951023931952, "Echo pulse width"=92, "Reserved"=0}, {"flags"=5, "Echo"=0, "Radial distance"=30.400000000000002, "Horizontal angle"=-0.16580627893946132, "Vertical angle"=-0.006981317007977317, "Echo pulse width"=132, "Reserved"=0}, {"flags"=4, "Echo"=1, "Radial distance"=35.68, "Horizontal angle"=-0.16580627893946132, "Vertical angle"=-0.006981317007977317, "Echo pulse width"=128, "Reserved"=0}, {"flags"=1, "Echo"=0, "Radial distance"=74.71000000000001, "Horizontal angle"=-0.17016960206944715, "Vertical angle"=0.00698131700797732, "Echo pulse width"=104, "Reserved"=31}, {"flags"=0, "Echo"=1, "Radial distance"=76.92, "Horizontal angle"=-0.17016960206944715, "Vertical angle"=0.00698131700797732, "Echo pulse width"=148, "Reserved"=32}, {"flags"=0, "Echo"=0, "Radial distance"=76.97, "Horizontal angle"=-0.17016960206944715, "Vertical angle"=0.020943951023931963, "Echo pulse width"=128, "Reserved"=32}, {"flags"=4, "Echo"=0, "Radial distance"=22.63, "Horizontal angle"=-0.17453292519943295, "Vertical angle"=-0.020943951023931952, "Echo pulse width"=224, "Reserved"=0}, {"flags"=4, "Echo"=0, "Radial distance"=33.160000000000004, "Horizontal angle"=-0.17453292519943295, "Vertical angle"=-0.006981317007977317, "Echo pulse width"=128, "Reserved"=0}, {"flags"=0, "Echo"=0, "Radial distance"=70.54, "Horizontal angle"=-0.17889624832941878, "Vertical angle"=0.00698131700797732, "Echo pulse width"=128, "Reserved"=33}, {"flags"=4, "Echo"=0, "Radial distance"=31.080000000000002, "Horizontal angle"=-0.1832595714594046, "Vertical angle"=-0.006981317007977317, "Echo pulse width"=128, "Reserved"=0}, {"flags"=0, "Echo"=0, "Radial distance"=62.67, "Horizontal angle"=-0.18762289458939044, "Vertical angle"=0.00698131700797732, "Echo pulse width"=136, "Reserved"=34}, {"flags"=4, "Echo"=0, "Radial distance"=24.96, "Horizontal angle"=-0.19198621771937624, "Vertical angle"=-0.020943951023931952, "Echo pulse width"=136, "Reserved"=0}, {"flags"=4, "Echo"=0, "Radial distance"=29.32, "Horizontal angle"=-0.19198621771937624, "Vertical angle"=-0.006981317007977317, "Echo pulse width"=136, "Reserved"=0}, {"flags"=0, "Echo"=0, "Radial distance"=58.64, "Horizontal angle"=-0.19634954084936207, "Vertical angle"=0.00698131700797732, "Echo pulse width"=148, "Reserved"=35}, {"flags"=0, "Echo"=0, "Radial distance"=70.59, "Horizontal angle"=-0.19634954084936207, "Vertical angle"=0.020943951023931963, "Echo pulse width"=116, "Reserved"=36}, {"flags"=4, "Echo"=0, "Radial distance"=23.59, "Horizontal angle"=-0.20071286397934787, "Vertical angle"=-0.020943951023931952, "Echo pulse width"=160, "Reserved"=0}, {"flags"=4, "Echo"=0, "Radial distance"=27.68, "Horizontal angle"=-0.20071286397934787, "Vertical angle"=-0.006981317007977317, "Echo pulse width"=136, "Reserved"=0}, {"flags"=0, "Echo"=0, "Radial distance"=54.61, "Horizontal angle"=-0.20507618710933373, "Vertical angle"=0.00698131700797732, "Echo pulse width"=152, "Reserved"=37}, {"flags"=0, "Echo"=0, "Radial distance"=94.06, "Horizontal angle"=-0.20507618710933373, "Vertical angle"=0.020943951023931963, "Echo pulse width"=108, "Reserved"=38}, {"flags"=4, "Echo"=0, "Radial distance"=22.32, "Horizontal angle"=-0.20943951023931953, "Vertical angle"=-0.020943951023931952, "Echo pulse width"=172, "Reserved"=0}, {"flags"=4, "Echo"=0, "Radial distance"=26.16, "Horizontal angle"=-0.20943951023931953, "Vertical angle"=-0.006981317007977317, "Echo pulse width"=140, "Reserved"=0}, {"flags"=5, "Echo"=0, "Radial distance"=49.84, "Horizontal angle"=-0.21380283336930533, "Vertical angle"=0.00698131700797732, "Echo pulse width"=148, "Reserved"=0}, {"flags"=0, "Echo"=1, "Radial distance"=54.76, "Horizontal angle"=-0.21380283336930533, "Vertical angle"=0.00698131700797732, "Echo pulse width"=56, "Reserved"=37}, {"flags"=1, "Echo"=0, "Radial distance"=58.45, "Horizontal angle"=-0.21380283336930533, "Vertical angle"=0.020943951023931963, "Echo pulse width"=32, "Reserved"=39}, {"flags"=0, "Echo"=1, "Radial distance"=62.25, "Horizontal angle"=-0.21380283336930533, "Vertical angle"=0.020943951023931963, "Echo pulse width"=64, "Reserved"=40}, {"flags"=4, "Echo"=0, "Radial distance"=21.150000000000002, "Horizontal angle"=-0.2181661564992912, "Vertical angle"=-0.020943951023931952, "Echo pulse width"=164, "Reserved"=0}, {"flags"=5, "Echo"=0, "Radial distance"=24.97, "Horizontal angle"=-0.2181661564992912, "Vertical angle"=-0.006981317007977317, "Echo pulse width"=144, "Reserved"=0}, {"flags"=4, "Echo"=1, "Radial distance"=26.35, "Horizontal angle"=-0.2181661564992912, "Vertical angle"=-0.006981317007977317, "Echo pulse width"=64, "Reserved"=0}, {"flags"=4, "Echo"=0, "Radial distance"=49.5, "Horizontal angle"=-0.222529479629277, "Vertical angle"=0.00698131700797732, "Echo pulse width"=160, "Reserved"=0}, {"flags"=0, "Echo"=0, "Radial distance"=93.9, "Horizontal angle"=-0.222529479629277, "Vertical angle"=0.020943951023931963, "Echo pulse width"=92, "Reserved"=41}, {"flags"=5, "Echo"=0, "Radial distance"=20.13, "Horizontal angle"=-0.22689280275926282, "Vertical angle"=-0.020943951023931952, "Echo pulse width"=148, "Reserved"=0}, {"flags"=4, "Echo"=1, "Radial distance"=22.12, "Horizontal angle"=-0.22689280275926282, "Vertical angle"=-0.020943951023931952, "Echo pulse width"=136, "Reserved"=0}, {"flags"=5, "Echo"=0, "Radial distance"=23.72, "Horizontal angle"=-0.22689280275926282, "Vertical angle"=-0.006981317007977317, "Echo pulse width"=136, "Reserved"=0}, {"flags"=4, "Echo"=1, "Radial distance"=25.01, "Horizontal angle"=-0.22689280275926282, "Vertical angle"=-0.006981317007977317, "Echo pulse width"=100, "Reserved"=0}, {"flags"=4, "Echo"=0, "Radial distance"=44.88, "Horizontal angle"=-0.23125612588924865, "Vertical angle"=0.00698131700797732, "Echo pulse width"=148, "Reserved"=0}, {"flags"=0, "Echo"=0, "Radial distance"=63.27, "Horizontal angle"=-0.23125612588924865, "Vertical angle"=0.020943951023931963, "Echo pulse width"=112, "Reserved"=42}, {"flags"=5, "Echo"=0, "Radial distance"=19.240000000000002, "Horizontal angle"=-0.23561944901923448, "Vertical angle"=-0.020943951023931952, "Echo pulse width"=168, "Reserved"=0}, {"flags"=0, "Echo"=1, "Radial distance"=22.32, "Horizontal angle"=-0.23561944901923448, "Vertical angle"=-0.020943951023931952, "Echo pulse width"=176, "Reserved"=43}, {"flags"=4, "Echo"=0, "Radial distance"=23.06, "Horizontal angle"=-0.23561944901923448, "Vertical angle"=-0.006981317007977317, "Echo pulse width"=244, "Reserved"=0}, {"flags"=4, "Echo"=0, "Radial distance"=44.5, "Horizontal angle"=-0.2399827721492203, "Vertical angle"=0.00698131700797732, "Echo pulse width"=160, "Reserved"=0}, {"flags"=0, "Echo"=0, "Radial distance"=74.82000000000001, "Horizontal angle"=-0.2399827721492203, "Vertical angle"=0.020943951023931963, "Echo pulse width"=84, "Reserved"=44}, {"flags"=5, "Echo"=0, "Radial distance"=18.48, "Horizontal angle"=-0.24434609527920614, "Vertical angle"=-0.020943951023931952, "Echo pulse width"=176, "Reserved"=0}, {"flags"=0, "Echo"=1, "Radial distance"=21.59, "Horizontal angle"=-0.24434609527920614, "Vertical angle"=-0.020943951023931952, "Echo pulse width"=116, "Reserved"=43}, {"flags"=0, "Echo"=0, "Radial distance"=22.1, "Horizontal angle"=-0.24434609527920614, "Vertical angle"=-0.006981317007977317, "Echo pulse width"=248, "Reserved"=43}, {"flags"=1, "Echo"=0, "Radial distance"=39.93, "Horizontal angle"=-0.24870941840919195, "Vertical angle"=0.00698131700797732, "Echo pulse width"=156, "Reserved"=45}, {"flags"=0, "Echo"=1, "Radial distance"=44.6, "Horizontal angle"=-0.24870941840919195, "Vertical angle"=0.00698131700797732, "Echo pulse width"=84, "Reserved"=46}, {"flags"=0, "Echo"=0, "Radial distance"=95.45, "Horizontal angle"=-0.24870941840919195, "Vertical angle"=0.020943951023931963, "Echo pulse width"=76, "Reserved"=47}, {"flags"=5, "Echo"=0, "Radial distance"=17.68, "Horizontal angle"=-0.2530727415391778, "Vertical angle"=-0.020943951023931952, "Echo pulse width"=176, "Reserved"=0}, {"flags"=0, "Echo"=1, "Radial distance"=20.39, "Horizontal angle"=-0.2530727415391778, "Vertical angle"=-0.020943951023931952, "Echo pulse width"=196, "Reserved"=48}, {"flags"=0, "Echo"=0, "Radial distance"=21.32, "Horizontal angle"=-0.2530727415391778, "Vertical angle"=-0.006981317007977317, "Echo pulse width"=264, "Reserved"=43}, {"flags"=0, "Echo"=0, "Radial distance"=39.7, "Horizontal angle"=-0.2574360646691636, "Vertical angle"=0.00698131700797732, "Echo pulse width"=168, "Reserved"=45}, {"flags"=0, "Echo"=0, "Radial distance"=39.83, "Horizontal angle"=-0.2574360646691636, "Vertical angle"=0.020943951023931963, "Echo pulse width"=116, "Reserved"=45}, {"flags"=5, "Echo"=0, "Radial distance"=17.03, "Horizontal angle"=-0.2617993877991494, "Vertical angle"=-0.020943951023931952, "Echo pulse width"=192, "Reserved"=0}, {"flags"=4, "Echo"=1, "Radial distance"=19.43, "Horizontal angle"=-0.2617993877991494, "Vertical angle"=-0.020943951023931952, "Echo pulse width"=220, "Reserved"=0}, {"flags"=1, "Echo"=0, "Radial distance"=20.57, "Horizontal angle"=-0.2617993877991494, "Vertical angle"=-0.006981317007977317, "Echo pulse width"=232, "Reserved"=48}, {"flags"=4, "Echo"=1, "Radial distance"=22.67, "Horizontal angle"=-0.2617993877991494, "Vertical angle"=-0.006981317007977317, "Echo pulse width"=120, "Reserved"=0}, {"flags"=0, "Echo"=0, "Radial distance"=39.62, "Horizontal angle"=-0.26616271092913524, "Vertical angle"=0.00698131700797732, "Echo pulse width"=168, "Reserved"=45}, {"flags"=0, "Echo"=0, "Radial distance"=39.83, "Horizontal angle"=-0.26616271092913524, "Vertical angle"=0.020943951023931963, "Echo pulse width"=116, "Reserved"=45}, {"flags"=4, "Echo"=0, "Radial distance"=16.53, "Horizontal angle"=-0.27052603405912107, "Vertical angle"=-0.020943951023931952, "Echo pulse width"=440, "Reserved"=0}, {"flags"=5, "Echo"=0, "Radial distance"=20.080000000000002, "Horizontal angle"=-0.27052603405912107, "Vertical angle"=-0.006981317007977317, "Echo pulse width"=260, "Reserved"=0}, {"flags"=4, "Echo"=1, "Radial distance"=22.47, "Horizontal angle"=-0.27052603405912107, "Vertical angle"=-0.006981317007977317, "Echo pulse width"=64, "Reserved"=0}, {"flags"=0, "Echo"=0, "Radial distance"=39.9, "Horizontal angle"=-0.2748893571891069, "Vertical angle"=0.00698131700797732, "Echo pulse width"=172, "Reserved"=45}, {"flags"=0, "Echo"=0, "Radial distance"=95.94, "Horizontal angle"=-0.2748893571891069, "Vertical angle"=0.020943951023931963, "Echo pulse width"=92, "Reserved"=49}, {"flags"=4, "Echo"=0, "Radial distance"=16.05, "Horizontal angle"=-0.2792526803190927, "Vertical angle"=-0.020943951023931952, "Echo pulse width"=424, "Reserved"=0}, {"flags"=5, "Echo"=0, "Radial distance"=19.42, "Horizontal angle"=-0.2792526803190927, "Vertical angle"=-0.006981317007977317, "Echo pulse width"=160, "Reserved"=0}, {"flags"=5, "Echo"=1, "Radial distance"=20.650000000000002, "Horizontal angle"=-0.2792526803190927, "Vertical angle"=-0.006981317007977317, "Echo pulse width"=76, "Reserved"=0}, {"flags"=4, "Echo"=2, "Radial distance"=22.6, "Horizontal angle"=-0.2792526803190927, "Vertical angle"=-0.006981317007977317, "Echo pulse width"=60, "Reserved"=0}, {"flags"=0, "Echo"=0, "Radial distance"=34.82, "Horizontal angle"=-0.28361600344907856, "Vertical angle"=0.00698131700797732, "Echo pulse width"=172, "Reserved"=50}, {"flags"=1, "Echo"=0, "Radial distance"=35.06, "Horizontal angle"=-0.28361600344907856, "Vertical angle"=0.020943951023931963, "Echo pulse width"=148, "Reserved"=50}, {"flags"=0, "Echo"=1, "Radial distance"=59.39, "Horizontal angle"=-0.28361600344907856, "Vertical angle"=0.020943951023931963, "Echo pulse width"=96, "Reserved"=51}, {"flags"=4, "Echo"=0, "Radial distance"=15.81, "Horizontal angle"=-0.28797932657906433, "Vertical angle"=-0.020943951023931952, "Echo pulse width"=392, "Reserved"=0}, {"flags"=5, "Echo"=0, "Radial distance"=19.1, "Horizontal angle"=-0.28797932657906433, "Vertical angle"=-0.006981317007977317, "Echo pulse width"=208, "Reserved"=0}, {"flags"=5, "Echo"=1, "Radial distance"=20.830000000000002, "Horizontal angle"=-0.28797932657906433, "Vertical angle"=-0.006981317007977317, "Echo pulse width"=40, "Reserved"=0}, {"flags"=4, "Echo"=2, "Radial distance"=22.11, "Horizontal angle"=-0.28797932657906433, "Vertical angle"=-0.006981317007977317, "Echo pulse width"=84, "Reserved"=0}, {"flags"=0, "Echo"=0, "Radial distance"=34.79, "Horizontal angle"=-0.2923426497090502, "Vertical angle"=0.00698131700797732, "Echo pulse width"=176, "Reserved"=50}, {"flags"=1, "Echo"=0, "Radial distance"=34.99, "Horizontal angle"=-0.2923426497090502, "Vertical angle"=0.020943951023931963, "Echo pulse width"=160, "Reserved"=50}, {"flags"=0, "Echo"=1, "Radial distance"=94.31, "Horizontal angle"=-0.2923426497090502, "Vertical angle"=0.020943951023931963, "Echo pulse width"=12, "Reserved"=52}, {"flags"=4, "Echo"=0, "Radial distance"=16.43, "Horizontal angle"=-0.296705972839036, "Vertical angle"=-0.020943951023931952, "Echo pulse width"=268, "Reserved"=0}, {"flags"=5, "Echo"=0, "Radial distance"=18.740000000000002, "Horizontal angle"=-0.296705972839036, "Vertical angle"=-0.006981317007977317, "Echo pulse width"=244, "Reserved"=0}, {"flags"=4, "Echo"=1, "Radial distance"=21.62, "Horizontal angle"=-0.296705972839036, "Vertical angle"=-0.006981317007977317, "Echo pulse width"=168, "Reserved"=0}, {"flags"=4, "Echo"=0, "Radial distance"=34.03, "Horizontal angle"=-0.3010692959690219, "Vertical angle"=0.00698131700797732, "Echo pulse width"=264, "Reserved"=0}, {"flags"=0, "Echo"=0, "Radial distance"=34.9, "Horizontal angle"=-0.3010692959690219, "Vertical angle"=0.020943951023931963, "Echo pulse width"=148, "Reserved"=50}, {"flags"=4, "Echo"=0, "Radial distance"=16.35, "Horizontal angle"=-0.30543261909900765, "Vertical angle"=-0.020943951023931952, "Echo pulse width"=216, "Reserved"=0}, {"flags"=5, "Echo"=0, "Radial distance"=18.28, "Horizontal angle"=-0.30543261909900765, "Vertical angle"=-0.006981317007977317, "Echo pulse width"=296, "Reserved"=0}, {"flags"=5, "Echo"=1, "Radial distance"=21.87, "Horizontal angle"=-0.30543261909900765, "Vertical angle"=-0.006981317007977317, "Echo pulse width"=124, "Reserved"=0}, {"flags"=4, "Echo"=2, "Radial distance"=25.73, "Horizontal angle"=-0.30543261909900765, "Vertical angle"=-0.006981317007977317, "Echo pulse width"=76, "Reserved"=0}, {"flags"=5, "Echo"=0, "Radial distance"=33.47, "Horizontal angle"=-0.3097959422289935, "Vertical angle"=0.00698131700797732, "Echo pulse width"=192, "Reserved"=0}, {"flags"=0, "Echo"=1, "Radial distance"=35.18, "Horizontal angle"=-0.3097959422289935, "Vertical angle"=0.00698131700797732, "Echo pulse width"=132, "Reserved"=50}, {"flags"=0, "Echo"=0, "Radial distance"=81.47, "Horizontal angle"=-0.3097959422289935, "Vertical angle"=0.020943951023931963, "Echo pulse width"=96, "Reserved"=53}, {"flags"=4, "Echo"=0, "Radial distance"=16.080000000000002, "Horizontal angle"=-0.3141592653589793, "Vertical angle"=-0.020943951023931952, "Echo pulse width"=180, "Reserved"=0}, {"flags"=5, "Echo"=0, "Radial distance"=18.080000000000002, "Horizontal angle"=-0.3141592653589793, "Vertical angle"=-0.006981317007977317, "Echo pulse width"=272, "Reserved"=0}, {"flags"=5, "Echo"=1, "Radial distance"=21.150000000000002, "Horizontal angle"=-0.3141592653589793, "Vertical angle"=-0.006981317007977317, "Echo pulse width"=112, "Reserved"=0}, {"flags"=4, "Echo"=2, "Radial distance"=31.16, "Horizontal angle"=-0.3141592653589793, "Vertical angle"=-0.006981317007977317, "Echo pulse width"=88, "Reserved"=0}, {"flags"=1, "Echo"=0, "Radial distance"=30.3, "Horizontal angle"=-0.31852258848896514, "Vertical angle"=0.00698131700797732, "Echo pulse width"=172, "Reserved"=54}, {"flags"=4, "Echo"=1, "Radial distance"=33.27, "Horizontal angle"=-0.31852258848896514, "Vertical angle"=0.00698131700797732, "Echo pulse width"=104, "Reserved"=0}, {"flags"=1, "Echo"=0, "Radial distance"=30.21, "Horizontal angle"=-0.31852258848896514, "Vertical angle"=0.020943951023931963, "Echo pulse width"=136, "Reserved"=54}, {"flags"=5, "Echo"=1, "Radial distance"=34.26, "Horizontal angle"=-0.31852258848896514, "Vertical angle"=0.020943951023931963, "Echo pulse width"=80, "Reserved"=0}, {"flags"=0, "Echo"=2, "Radial distance"=83.43, "Horizontal angle"=-0.31852258848896514, "Vertical angle"=0.020943951023931963, "Echo pulse width"=112, "Reserved"=55}, {"flags"=4, "Echo"=0, "Radial distance"=15.67, "Horizontal angle"=-0.32288591161895097, "Vertical angle"=-0.020943951023931952, "Echo pulse width"=184, "Reserved"=0}, {"flags"=5, "Echo"=0, "Radial distance"=17.68, "Horizontal angle"=-0.32288591161895097, "Vertical angle"=-0.006981317007977317, "Echo pulse width"=312, "Reserved"=0}, {"flags"=5, "Echo"=1, "Radial distance"=20.95, "Horizontal angle"=-0.32288591161895097, "Vertical angle"=-0.006981317007977317, "Echo pulse width"=80, "Reserved"=0}, {"flags"=4, "Echo"=2, "Radial distance"=24.71, "Horizontal angle"=-0.32288591161895097, "Vertical angle"=-0.006981317007977317, "Echo pulse width"=84, "Reserved"=0}, {"flags"=0, "Echo"=0, "Radial distance"=30.07, "Horizontal angle"=-0.3272492347489368, "Vertical angle"=0.00698131700797732, "Echo pulse width"=180, "Reserved"=54}, {"flags"=1, "Echo"=0, "Radial distance"=30.080000000000002, "Horizontal angle"=-0.3272492347489368, "Vertical angle"=0.020943951023931963, "Echo pulse width"=168, "Reserved"=54}, {"flags"=0, "Echo"=1, "Radial distance"=63.910000000000004, "Horizontal angle"=-0.3272492347489368, "Vertical angle"=0.020943951023931963, "Echo pulse width"=112, "Reserved"=56}, {"flags"=4, "Echo"=0, "Radial distance"=15.31, "Horizontal angle"=-0.33161255787892263, "Vertical angle"=-0.020943951023931952, "Echo pulse width"=192, "Reserved"=0}, {"flags"=5, "Echo"=0, "Radial distance"=17.8, "Horizontal angle"=-0.33161255787892263, "Vertical angle"=-0.006981317007977317, "Echo pulse width"=292, "Reserved"=0}, {"flags"=5, "Echo"=1, "Radial distance"=20.87, "Horizontal angle"=-0.33161255787892263, "Vertical angle"=-0.006981317007977317, "Echo pulse width"=44, "Reserved"=0}, {"flags"=4, "Echo"=2, "Radial distance"=24.88, "Horizontal angle"=-0.33161255787892263, "Vertical angle"=-0.006981317007977317, "Echo pulse width"=92, "Reserved"=0}, {"flags"=0, "Echo"=0, "Radial distance"=29.98, "Horizontal angle"=-0.3359758810089084, "Vertical angle"=0.00698131700797732, "Echo pulse width"=172, "Reserved"=54}, {"flags"=1, "Echo"=0, "Radial distance"=30.04, "Horizontal angle"=-0.3359758810089084, "Vertical angle"=0.020943951023931963, "Echo pulse width"=172, "Reserved"=54}, {"flags"=0, "Echo"=1, "Radial distance"=82.82000000000001, "Horizontal angle"=-0.3359758810089084, "Vertical angle"=0.020943951023931963, "Echo pulse width"=104, "Reserved"=57}, {"flags"=4, "Echo"=0, "Radial distance"=14.93, "Horizontal angle"=-0.3403392041388943, "Vertical angle"=-0.020943951023931952, "Echo pulse width"=208, "Reserved"=0}, {"flags"=5, "Echo"=0, "Radial distance"=17.44, "Horizontal angle"=-0.3403392041388943, "Vertical angle"=-0.006981317007977317, "Echo pulse width"=312, "Reserved"=0}, {"flags"=5, "Echo"=1, "Radial distance"=24.6, "Horizontal angle"=-0.3403392041388943, "Vertical angle"=-0.006981317007977317, "Echo pulse width"=36, "Reserved"=0}, {"flags"=4, "Echo"=2, "Radial distance"=28.55, "Horizontal angle"=-0.3403392041388943, "Vertical angle"=-0.006981317007977317, "Echo pulse width"=120, "Reserved"=0}, {"flags"=0, "Echo"=0, "Radial distance"=30.11, "Horizontal angle"=-0.34470252726888007, "Vertical angle"=0.00698131700797732, "Echo pulse width"=176, "Reserved"=54}, {"flags"=0, "Echo"=0, "Radial distance"=30.11, "Horizontal angle"=-0.34470252726888007, "Vertical angle"=0.020943951023931963, "Echo pulse width"=160, "Reserved"=54}, {"flags"=4, "Echo"=0, "Radial distance"=14.55, "Horizontal angle"=-0.3490658503988659, "Vertical angle"=-0.020943951023931952, "Echo pulse width"=228, "Reserved"=0}, {"flags"=5, "Echo"=0, "Radial distance"=16.85, "Horizontal angle"=-0.3490658503988659, "Vertical angle"=-0.006981317007977317, "Echo pulse width"=336, "Reserved"=0}, {"flags"=4, "Echo"=1, "Radial distance"=27.68, "Horizontal angle"=-0.3490658503988659, "Vertical angle"=-0.006981317007977317, "Echo pulse width"=128, "Reserved"=0}, {"flags"=1, "Echo"=0, "Radial distance"=30.38, "Horizontal angle"=-0.3534291735288517, "Vertical angle"=0.00698131700797732, "Echo pulse width"=164, "Reserved"=54}, {"flags"=4, "Echo"=1, "Radial distance"=31.77, "Horizontal angle"=-0.3534291735288517, "Vertical angle"=0.00698131700797732, "Echo pulse width"=88, "Reserved"=0}, {"flags"=1, "Echo"=0, "Radial distance"=30.43, "Horizontal angle"=-0.3534291735288517, "Vertical angle"=0.020943951023931963, "Echo pulse width"=116, "Reserved"=54}, {"flags"=0, "Echo"=1, "Radial distance"=84.26, "Horizontal angle"=-0.3534291735288517, "Vertical angle"=0.020943951023931963, "Echo pulse width"=92, "Reserved"=58}, {"flags"=4, "Echo"=0, "Radial distance"=14.200000000000001, "Horizontal angle"=-0.35779249665883756, "Vertical angle"=-0.020943951023931952, "Echo pulse width"=220, "Reserved"=0}, {"flags"=5, "Echo"=0, "Radial distance"=16.81, "Horizontal angle"=-0.35779249665883756, "Vertical angle"=-0.006981317007977317, "Echo pulse width"=388, "Reserved"=0}, {"flags"=0, "Echo"=1, "Radial distance"=26.76, "Horizontal angle"=-0.35779249665883756, "Vertical angle"=-0.006981317007977317, "Echo pulse width"=132, "Reserved"=59}, {"flags"=1, "Echo"=0, "Radial distance"=27.01, "Horizontal angle"=-0.3621558197888234, "Vertical angle"=0.00698131700797732, "Echo pulse width"=120, "Reserved"=59}, {"flags"=4, "Echo"=1, "Radial distance"=31.62, "Horizontal angle"=-0.3621558197888234, "Vertical angle"=0.00698131700797732, "Echo pulse width"=132, "Reserved"=0}, {"flags"=4, "Echo"=0, "Radial distance"=13.790000000000001, "Horizontal angle"=-0.3665191429188092, "Vertical angle"=-0.020943951023931952, "Echo pulse width"=248, "Reserved"=0}, {"flags"=5, "Echo"=0, "Radial distance"=16.73, "Horizontal angle"=-0.3665191429188092, "Vertical angle"=-0.006981317007977317, "Echo pulse width"=360, "Reserved"=0}, {"flags"=4, "Echo"=1, "Radial distance"=26.240000000000002, "Horizontal angle"=-0.3665191429188092, "Vertical angle"=-0.006981317007977317, "Echo pulse width"=128, "Reserved"=0}, {"flags"=0, "Echo"=0, "Radial distance"=25.43, "Horizontal angle"=-0.370882466048795, "Vertical angle"=0.00698131700797732, "Echo pulse width"=192, "Reserved"=60}, {"flags"=1, "Echo"=0, "Radial distance"=25.310000000000002, "Horizontal angle"=-0.370882466048795, "Vertical angle"=0.020943951023931963, "Echo pulse width"=160, "Reserved"=60}, {"flags"=0, "Echo"=1, "Radial distance"=95.93, "Horizontal angle"=-0.370882466048795, "Vertical angle"=0.020943951023931963, "Echo pulse width"=36, "Reserved"=61}, {"flags"=4, "Echo"=0, "Radial distance"=13.51, "Horizontal angle"=-0.3752457891787809, "Vertical angle"=-0.020943951023931952, "Echo pulse width"=240, "Reserved"=0}, {"flags"=5, "Echo"=0, "Radial distance"=16.41, "Horizontal angle"=-0.3752457891787809, "Vertical angle"=-0.006981317007977317, "Echo pulse width"=364, "Reserved"=0}, {"flags"=0, "Echo"=1, "Radial distance"=25.55, "Horizontal angle"=-0.3752457891787809, "Vertical angle"=-0.006981317007977317, "Echo pulse width"=124, "Reserved"=60}, {"flags"=0, "Echo"=0, "Radial distance"=25.19, "Horizontal angle"=-0.37960911230876665, "Vertical angle"=0.00698131700797732, "Echo pulse width"=180, "Reserved"=60}, {"flags"=1, "Echo"=0, "Radial distance"=25.21, "Horizontal angle"=-0.37960911230876665, "Vertical angle"=0.020943951023931963, "Echo pulse width"=184, "Reserved"=60}, {"flags"=0, "Echo"=1, "Radial distance"=29.01, "Horizontal angle"=-0.37960911230876665, "Vertical angle"=0.020943951023931963, "Echo pulse width"=136, "Reserved"=62}, {"flags"=4, "Echo"=0, "Radial distance"=13.11, "Horizontal angle"=-0.3839724354387525, "Vertical angle"=-0.020943951023931952, "Echo pulse width"=272, "Reserved"=0}, {"flags"=5, "Echo"=0, "Radial distance"=16.09, "Horizontal angle"=-0.3839724354387525, "Vertical angle"=-0.006981317007977317, "Echo pulse width"=372, "Reserved"=0}, {"flags"=0, "Echo"=1, "Radial distance"=24.76, "Horizontal angle"=-0.3839724354387525, "Vertical angle"=-0.006981317007977317, "Echo pulse width"=136, "Reserved"=60}, {"flags"=0, "Echo"=0, "Radial distance"=25.11, "Horizontal angle"=-0.3883357585687383, "Vertical angle"=0.00698131700797732, "Echo pulse width"=176, "Reserved"=60}, {"flags"=1, "Echo"=0, "Radial distance"=25.13, "Horizontal angle"=-0.3883357585687383, "Vertical angle"=0.020943951023931963, "Echo pulse width"=188, "Reserved"=60}, {"flags"=0, "Echo"=1, "Radial distance"=29.09, "Horizontal angle"=-0.3883357585687383, "Vertical angle"=0.020943951023931963, "Echo pulse width"=136, "Reserved"=62}, {"flags"=4, "Echo"=0, "Radial distance"=12.91, "Horizontal angle"=-0.39269908169872414, "Vertical angle"=-0.020943951023931952, "Echo pulse width"=276, "Reserved"=0}, {"flags"=5, "Echo"=0, "Radial distance"=15.88, "Horizontal angle"=-0.39269908169872414, "Vertical angle"=-0.006981317007977317, "Echo pulse width"=216, "Reserved"=0}, {"flags"=5, "Echo"=1, "Radial distance"=18.09, "Horizontal angle"=-0.39269908169872414, "Vertical angle"=-0.006981317007977317, "Echo pulse width"=152, "Reserved"=0}, {"flags"=4, "Echo"=2, "Radial distance"=24.32, "Horizontal angle"=-0.39269908169872414, "Vertical angle"=-0.006981317007977317, "Echo pulse width"=136, "Reserved"=0}, {"flags"=0, "Echo"=0, "Radial distance"=25.150000000000002, "Horizontal angle"=-0.39706240482870997, "Vertical angle"=0.00698131700797732, "Echo pulse width"=192, "Reserved"=60}, {"flags"=1, "Echo"=0, "Radial distance"=25.17, "Horizontal angle"=-0.39706240482870997, "Vertical angle"=0.020943951023931963, "Echo pulse width"=184, "Reserved"=60}, {"flags"=0, "Echo"=1, "Radial distance"=29.14, "Horizontal angle"=-0.39706240482870997, "Vertical angle"=0.020943951023931963, "Echo pulse width"=144, "Reserved"=62}, {"flags"=4, "Echo"=0, "Radial distance"=12.55, "Horizontal angle"=-0.40142572795869574, "Vertical angle"=-0.020943951023931952, "Echo pulse width"=300, "Reserved"=0}, {"flags"=5, "Echo"=0, "Radial distance"=15.780000000000001, "Horizontal angle"=-0.40142572795869574, "Vertical angle"=-0.006981317007977317, "Echo pulse width"=212, "Reserved"=0}, {"flags"=5, "Echo"=1, "Radial distance"=17.85, "Horizontal angle"=-0.40142572795869574, "Vertical angle"=-0.006981317007977317, "Echo pulse width"=148, "Reserved"=0}, {"flags"=4, "Echo"=2, "Radial distance"=23.85, "Horizontal angle"=-0.40142572795869574, "Vertical angle"=-0.006981317007977317, "Echo pulse width"=144, "Reserved"=0}, {"flags"=0, "Echo"=0, "Radial distance"=25.19, "Horizontal angle"=-0.40578905108868163, "Vertical angle"=0.00698131700797732, "Echo pulse width"=196, "Reserved"=60}, {"flags"=0, "Echo"=0, "Radial distance"=25.44, "Horizontal angle"=-0.40578905108868163, "Vertical angle"=0.020943951023931963, "Echo pulse width"=288, "Reserved"=60}, {"flags"=4, "Echo"=0, "Radial distance"=12.31, "Horizontal angle"=-0.41015237421866746, "Vertical angle"=-0.020943951023931952, "Echo pulse width"=304, "Reserved"=0}, {"flags"=5, "Echo"=0, "Radial distance"=15.530000000000001, "Horizontal angle"=-0.41015237421866746, "Vertical angle"=-0.006981317007977317, "Echo pulse width"=232, "Reserved"=0}, {"flags"=5, "Echo"=1, "Radial distance"=18.35, "Horizontal angle"=-0.41015237421866746, "Vertical angle"=-0.006981317007977317, "Echo pulse width"=204, "Reserved"=0}, {"flags"=4, "Echo"=2, "Radial distance"=23.41, "Horizontal angle"=-0.41015237421866746, "Vertical angle"=-0.006981317007977317, "Echo pulse width"=152, "Reserved"=0}, {"flags"=1, "Echo"=0, "Radial distance"=25.150000000000002, "Horizontal angle"=-0.4145156973486533, "Vertical angle"=0.00698131700797732, "Echo pulse width"=284, "Reserved"=60}, {"flags"=4, "Echo"=1, "Radial distance"=42.410000000000004, "Horizontal angle"=-0.4145156973486533, "Vertical angle"=0.00698131700797732, "Echo pulse width"=156, "Reserved"=0}, {"flags"=1, "Echo"=0, "Radial distance"=61.690000000000005, "Horizontal angle"=-0.4145156973486533, "Vertical angle"=0.020943951023931963, "Echo pulse width"=64, "Reserved"=63}, {"flags"=0, "Echo"=1, "Radial distance"=83.67, "Horizontal angle"=-0.4145156973486533, "Vertical angle"=0.020943951023931963, "Echo pulse width"=100, "Reserved"=64}, {"flags"=4, "Echo"=0, "Radial distance"=12.030000000000001, "Horizontal angle"=-0.41887902047863906, "Vertical angle"=-0.020943951023931952, "Echo pulse width"=260, "Reserved"=0}, {"flags"=5, "Echo"=0, "Radial distance"=15.24, "Horizontal angle"=-0.41887902047863906, "Vertical angle"=-0.006981317007977317, "Echo pulse width"=256, "Reserved"=0}, {"flags"=5, "Echo"=1, "Radial distance"=18.18, "Horizontal angle"=-0.41887902047863906, "Vertical angle"=-0.006981317007977317, "Echo pulse width"=212, "Reserved"=0}, {"flags"=4, "Echo"=2, "Radial distance"=22.73, "Horizontal angle"=-0.41887902047863906, "Vertical angle"=-0.006981317007977317, "Echo pulse width"=144, "Reserved"=0}, {"flags"=5, "Echo"=0, "Radial distance"=25.150000000000002, "Horizontal angle"=-0.4232423436086249, "Vertical angle"=0.00698131700797732, "Echo pulse width"=260, "Reserved"=0}, {"flags"=5, "Echo"=1, "Radial distance"=29.25, "Horizontal angle"=-0.4232423436086249, "Vertical angle"=0.00698131700797732, "Echo pulse width"=92, "Reserved"=0}, {"flags"=4, "Echo"=2, "Radial distance"=42.46, "Horizontal angle"=-0.4232423436086249, "Vertical angle"=0.00698131700797732, "Echo pulse width"=164, "Reserved"=0}, {"flags"=4, "Echo"=0, "Radial distance"=44.550000000000004, "Horizontal angle"=-0.4232423436086249, "Vertical angle"=0.020943951023931963, "Echo pulse width"=164, "Reserved"=0}, {"flags"=4, "Echo"=0, "Radial distance"=11.86, "Horizontal angle"=-0.42760566673861067, "Vertical angle"=-0.020943951023931952, "Echo pulse width"=224, "Reserved"=0}, {"flags"=5, "Echo"=0, "Radial distance"=15.120000000000001, "Horizontal angle"=-0.42760566673861067, "Vertical angle"=-0.006981317007977317, "Echo pulse width"=276, "Reserved"=0}, {"flags"=5, "Echo"=1, "Radial distance"=18.28, "Horizontal angle"=-0.42760566673861067, "Vertical angle"=-0.006981317007977317, "Echo pulse width"=136, "Reserved"=0}, {"flags"=4, "Echo"=2, "Radial distance"=22.29, "Horizontal angle"=-0.42760566673861067, "Vertical angle"=-0.006981317007977317, "Echo pulse width"=148, "Reserved"=0}, {"flags"=5, "Echo"=0, "Radial distance"=24.990000000000002, "Horizontal angle"=-0.4319689898685966, "Vertical angle"=0.00698131700797732, "Echo pulse width"=256, "Reserved"=0}, {"flags"=5, "Echo"=1, "Radial distance"=32.85, "Horizontal angle"=-0.4319689898685966, "Vertical angle"=0.00698131700797732, "Echo pulse width"=92, "Reserved"=0}, {"flags"=4, "Echo"=2, "Radial distance"=42.54, "Horizontal angle"=-0.4319689898685966, "Vertical angle"=0.00698131700797732, "Echo pulse width"=160, "Reserved"=0}, {"flags"=4, "Echo"=0, "Radial distance"=11.55, "Horizontal angle"=-0.4363323129985824, "Vertical angle"=-0.020943951023931952, "Echo pulse width"=260, "Reserved"=0}, {"flags"=0, "Echo"=0, "Radial distance"=12.5, "Horizontal angle"=-0.4363323129985824, "Vertical angle"=-0.006981317007977317, "Echo pulse width"=160, "Reserved"=65}, {"flags"=0, "Echo"=0, "Radial distance"=12.450000000000001, "Horizontal angle"=-0.4406956361285682, "Vertical angle"=0.00698131700797732, "Echo pulse width"=156, "Reserved"=65}, {"flags"=0, "Echo"=0, "Radial distance"=12.47, "Horizontal angle"=-0.4406956361285682, "Vertical angle"=0.020943951023931963, "Echo pulse width"=160, "Reserved"=65}, {"flags"=4, "Echo"=0, "Radial distance"=11.51, "Horizontal angle"=-0.445058959258554, "Vertical angle"=-0.020943951023931952, "Echo pulse width"=248, "Reserved"=0}, {"flags"=0, "Echo"=0, "Radial distance"=12.48, "Horizontal angle"=-0.445058959258554, "Vertical angle"=-0.006981317007977317, "Echo pulse width"=148, "Reserved"=65}, {"flags"=0, "Echo"=0, "Radial distance"=12.5, "Horizontal angle"=-0.4494222823885398, "Vertical angle"=0.00698131700797732, "Echo pulse width"=96, "Reserved"=65}, {"flags"=0, "Echo"=0, "Radial distance"=12.44, "Horizontal angle"=-0.4494222823885398, "Vertical angle"=0.020943951023931963, "Echo pulse width"=104, "Reserved"=65}, {"flags"=4, "Echo"=0, "Radial distance"=11.15, "Horizontal angle"=-0.45378560551852565, "Vertical angle"=-0.020943951023931952, "Echo pulse width"=308, "Reserved"=0}, {"flags"=1, "Echo"=0, "Radial distance"=12.6, "Horizontal angle"=-0.45378560551852565, "Vertical angle"=-0.006981317007977317, "Echo pulse width"=128, "Reserved"=65}, {"flags"=5, "Echo"=1, "Radial distance"=15.76, "Horizontal angle"=-0.45378560551852565, "Vertical angle"=-0.006981317007977317, "Echo pulse width"=272, "Reserved"=0}, {"flags"=4, "Echo"=2, "Radial distance"=18.59, "Horizontal angle"=-0.45378560551852565, "Vertical angle"=-0.006981317007977317, "Echo pulse width"=124, "Reserved"=0}, {"flags"=0, "Echo"=0, "Radial distance"=20.79, "Horizontal angle"=-0.45814892864851153, "Vertical angle"=0.00698131700797732, "Echo pulse width"=192, "Reserved"=66}, {"flags"=0, "Echo"=0, "Radial distance"=20.57, "Horizontal angle"=-0.45814892864851153, "Vertical angle"=0.020943951023931963, "Echo pulse width"=184, "Reserved"=66}, {"flags"=4, "Echo"=0, "Radial distance"=11.15, "Horizontal angle"=-0.4625122517784973, "Vertical angle"=-0.020943951023931952, "Echo pulse width"=288, "Reserved"=0}, {"flags"=5, "Echo"=0, "Radial distance"=14.96, "Horizontal angle"=-0.4625122517784973, "Vertical angle"=-0.006981317007977317, "Echo pulse width"=288, "Reserved"=0}, {"flags"=5, "Echo"=1, "Radial distance"=18.31, "Horizontal angle"=-0.4625122517784973, "Vertical angle"=-0.006981317007977317, "Echo pulse width"=80, "Reserved"=0}, {"flags"=0, "Echo"=2, "Radial distance"=20.45, "Horizontal angle"=-0.4625122517784973, "Vertical angle"=-0.006981317007977317, "Echo pulse width"=144, "Reserved"=66}, {"flags"=0, "Echo"=0, "Radial distance"=20.6, "Horizontal angle"=-0.46687557490848314, "Vertical angle"=0.00698131700797732, "Echo pulse width"=184, "Reserved"=66}, {"flags"=0, "Echo"=0, "Radial distance"=20.400000000000002, "Horizontal angle"=-0.46687557490848314, "Vertical angle"=0.020943951023931963, "Echo pulse width"=180, "Reserved"=66}, {"flags"=4, "Echo"=0, "Radial distance"=10.89, "Horizontal angle"=-0.47123889803846897, "Vertical angle"=-0.020943951023931952, "Echo pulse width"=348, "Reserved"=0}, {"flags"=5, "Echo"=0, "Radial distance"=14.290000000000001, "Horizontal angle"=-0.47123889803846897, "Vertical angle"=-0.006981317007977317, "Echo pulse width"=344, "Reserved"=0}, {"flags"=5, "Echo"=1, "Radial distance"=18.11, "Horizontal angle"=-0.47123889803846897, "Vertical angle"=-0.006981317007977317, "Echo pulse width"=64, "Reserved"=0}, {"flags"=4, "Echo"=2, "Radial distance"=20.09, "Horizontal angle"=-0.47123889803846897, "Vertical angle"=-0.006981317007977317, "Echo pulse width"=152, "Reserved"=0}, {"flags"=0, "Echo"=0, "Radial distance"=20.48, "Horizontal angle"=-0.47560222116845474, "Vertical angle"=0.00698131700797732, "Echo pulse width"=184, "Reserved"=66}, {"flags"=0, "Echo"=0, "Radial distance"=20.400000000000002, "Horizontal angle"=-0.47560222116845474, "Vertical angle"=0.020943951023931963, "Echo pulse width"=180, "Reserved"=66}, {"flags"=4, "Echo"=0, "Radial distance"=10.950000000000001, "Horizontal angle"=-0.4799655442984406, "Vertical angle"=-0.020943951023931952, "Echo pulse width"=288, "Reserved"=0}, {"flags"=5, "Echo"=0, "Radial distance"=14.88, "Horizontal angle"=-0.4799655442984406, "Vertical angle"=-0.006981317007977317, "Echo pulse width"=280, "Reserved"=0}, {"flags"=5, "Echo"=1, "Radial distance"=16.87, "Horizontal angle"=-0.4799655442984406, "Vertical angle"=-0.006981317007977317, "Echo pulse width"=44, "Reserved"=0}, {"flags"=4, "Echo"=2, "Radial distance"=17.93, "Horizontal angle"=-0.4799655442984406, "Vertical angle"=-0.006981317007977317, "Echo pulse width"=48, "Reserved"=0}, {"flags"=0, "Echo"=0, "Radial distance"=20.5, "Horizontal angle"=-0.48432886742842646, "Vertical angle"=0.00698131700797732, "Echo pulse width"=200, "Reserved"=66}, {"flags"=0, "Echo"=0, "Radial distance"=20.400000000000002, "Horizontal angle"=-0.48432886742842646, "Vertical angle"=0.020943951023931963, "Echo pulse width"=180, "Reserved"=66}, {"flags"=4, "Echo"=0, "Radial distance"=10.69, "Horizontal angle"=-0.4886921905584123, "Vertical angle"=-0.020943951023931952, "Echo pulse width"=344, "Reserved"=0}, {"flags"=5, "Echo"=0, "Radial distance"=14.09, "Horizontal angle"=-0.4886921905584123, "Vertical angle"=-0.006981317007977317, "Echo pulse width"=404, "Reserved"=0}, {"flags"=4, "Echo"=1, "Radial distance"=19.37, "Horizontal angle"=-0.4886921905584123, "Vertical angle"=-0.006981317007977317, "Echo pulse width"=152, "Reserved"=0}, {"flags"=0, "Echo"=0, "Radial distance"=20.38, "Horizontal angle"=-0.49305551368839806, "Vertical angle"=0.00698131700797732, "Echo pulse width"=240, "Reserved"=66}, {"flags"=0, "Echo"=0, "Radial distance"=20.52, "Horizontal angle"=-0.49305551368839806, "Vertical angle"=0.020943951023931963, "Echo pulse width"=176, "Reserved"=66}, {"flags"=4, "Echo"=0, "Radial distance"=10.790000000000001, "Horizontal angle"=-0.4974188368183839, "Vertical angle"=-0.020943951023931952, "Echo pulse width"=288, "Reserved"=0}, {"flags"=5, "Echo"=0, "Radial distance"=14.55, "Horizontal angle"=-0.4974188368183839, "Vertical angle"=-0.006981317007977317, "Echo pulse width"=328, "Reserved"=0}, {"flags"=4, "Echo"=1, "Radial distance"=19.01, "Horizontal angle"=-0.4974188368183839, "Vertical angle"=-0.006981317007977317, "Echo pulse width"=156, "Reserved"=0}, {"flags"=5, "Echo"=0, "Radial distance"=20.11, "Horizontal angle"=-0.5017821599483697, "Vertical angle"=0.00698131700797732, "Echo pulse width"=344, "Reserved"=0}, {"flags"=5, "Echo"=1, "Radial distance"=24.560000000000002, "Horizontal angle"=-0.5017821599483697, "Vertical angle"=0.00698131700797732, "Echo pulse width"=80, "Reserved"=0}, {"flags"=4, "Echo"=2, "Radial distance"=30.28, "Horizontal angle"=-0.5017821599483697, "Vertical angle"=0.00698131700797732, "Echo pulse width"=188, "Reserved"=0}, {"flags"=5, "Echo"=0, "Radial distance"=20.84, "Horizontal angle"=-0.5017821599483697, "Vertical angle"=0.020943951023931963, "Echo pulse width"=168, "Reserved"=0}, {"flags"=5, "Echo"=1, "Radial distance"=31.61, "Horizontal angle"=-0.5017821599483697, "Vertical angle"=0.020943951023931963, "Echo pulse width"=76, "Reserved"=0}, {"flags"=4, "Echo"=2, "Radial distance"=33.15, "Horizontal angle"=-0.5017821599483697, "Vertical angle"=0.020943951023931963, "Echo pulse width"=112, "Reserved"=0}, {"flags"=4, "Echo"=0, "Radial distance"=10.53, "Horizontal angle"=-0.5061454830783556, "Vertical angle"=-0.020943951023931952, "Echo pulse width"=344, "Reserved"=0}, {"flags"=5, "Echo"=0, "Radial distance"=13.85, "Horizontal angle"=-0.5061454830783556, "Vertical angle"=-0.006981317007977317, "Echo pulse width"=452, "Reserved"=0}, {"flags"=4, "Echo"=1, "Radial distance"=18.650000000000002, "Horizontal angle"=-0.5061454830783556, "Vertical angle"=-0.006981317007977317, "Echo pulse width"=156, "Reserved"=0}, {"flags"=5, "Echo"=0, "Radial distance"=19.55, "Horizontal angle"=-0.5105088062083414, "Vertical angle"=0.00698131700797732, "Echo pulse width"=176, "Reserved"=0}, {"flags"=5, "Echo"=1, "Radial distance"=21.330000000000002, "Horizontal angle"=-0.5105088062083414, "Vertical angle"=0.00698131700797732, "Echo pulse width"=88, "Reserved"=0}, {"flags"=4, "Echo"=2, "Radial distance"=23.81, "Horizontal angle"=-0.5105088062083414, "Vertical angle"=0.00698131700797732, "Echo pulse width"=120, "Reserved"=0}, {"flags"=4, "Echo"=0, "Radial distance"=31.68, "Horizontal angle"=-0.5105088062083414, "Vertical angle"=0.020943951023931963, "Echo pulse width"=220, "Reserved"=0}, {"flags"=4, "Echo"=0, "Radial distance"=10.51, "Horizontal angle"=-0.5148721293383272, "Vertical angle"=-0.020943951023931952, "Echo pulse width"=288, "Reserved"=0}, {"flags"=5, "Echo"=0, "Radial distance"=14.280000000000001, "Horizontal angle"=-0.5148721293383272, "Vertical angle"=-0.006981317007977317, "Echo pulse width"=364, "Reserved"=0}, {"flags"=4, "Echo"=1, "Radial distance"=18.37, "Horizontal angle"=-0.5148721293383272, "Vertical angle"=-0.006981317007977317, "Echo pulse width"=148, "Reserved"=0}, {"flags"=5, "Echo"=0, "Radial distance"=19.23, "Horizontal angle"=-0.519235452468313, "Vertical angle"=0.00698131700797732, "Echo pulse width"=192, "Reserved"=0}, {"flags"=5, "Echo"=1, "Radial distance"=23.71, "Horizontal angle"=-0.519235452468313, "Vertical angle"=0.00698131700797732, "Echo pulse width"=140, "Reserved"=0}, {"flags"=4, "Echo"=2, "Radial distance"=30.400000000000002, "Horizontal angle"=-0.519235452468313, "Vertical angle"=0.00698131700797732, "Echo pulse width"=188, "Reserved"=0}, {"flags"=4, "Echo"=0, "Radial distance"=31.64, "Horizontal angle"=-0.519235452468313, "Vertical angle"=0.020943951023931963, "Echo pulse width"=216, "Reserved"=0}, {"flags"=4, "Echo"=0, "Radial distance"=10.31, "Horizontal angle"=-0.5235987755982988, "Vertical angle"=-0.020943951023931952, "Echo pulse width"=340, "Reserved"=0}, {"flags"=5, "Echo"=0, "Radial distance"=13.57, "Horizontal angle"=-0.5235987755982988, "Vertical angle"=-0.006981317007977317, "Echo pulse width"=428, "Reserved"=0}, {"flags"=4, "Echo"=1, "Radial distance"=18.05, "Horizontal angle"=-0.5235987755982988, "Vertical angle"=-0.006981317007977317, "Echo pulse width"=156, "Reserved"=0}, {"flags"=5, "Echo"=0, "Radial distance"=18.88, "Horizontal angle"=-0.5279620987282847, "Vertical angle"=0.00698131700797732, "Echo pulse width"=228, "Reserved"=0}, {"flags"=5, "Echo"=1, "Radial distance"=23.35, "Horizontal angle"=-0.5279620987282847, "Vertical angle"=0.00698131700797732, "Echo pulse width"=104, "Reserved"=0}, {"flags"=4, "Echo"=2, "Radial distance"=30.34, "Horizontal angle"=-0.5279620987282847, "Vertical angle"=0.00698131700797732, "Echo pulse width"=204, "Reserved"=0}, {"flags"=4, "Echo"=0, "Radial distance"=31.66, "Horizontal angle"=-0.5279620987282847, "Vertical angle"=0.020943951023931963, "Echo pulse width"=212, "Reserved"=0}, {"flags"=4, "Echo"=0, "Radial distance"=10.39, "Horizontal angle"=-0.5323254218582705, "Vertical angle"=-0.020943951023931952, "Echo pulse width"=288, "Reserved"=0}, {"flags"=5, "Echo"=0, "Radial distance"=14.51, "Horizontal angle"=-0.5323254218582705, "Vertical angle"=-0.006981317007977317, "Echo pulse width"=316, "Reserved"=0}, {"flags"=4, "Echo"=1, "Radial distance"=17.66, "Horizontal angle"=-0.5323254218582705, "Vertical angle"=-0.006981317007977317, "Echo pulse width"=164, "Reserved"=0}, {"flags"=5, "Echo"=0, "Radial distance"=18.67, "Horizontal angle"=-0.5366887449882564, "Vertical angle"=0.00698131700797732, "Echo pulse width"=248, "Reserved"=0}, {"flags"=4, "Echo"=1, "Radial distance"=30.51, "Horizontal angle"=-0.5366887449882564, "Vertical angle"=0.00698131700797732, "Echo pulse width"=176, "Reserved"=0}, {"flags"=5, "Echo"=0, "Radial distance"=31.76, "Horizontal angle"=-0.5366887449882564, "Vertical angle"=0.020943951023931963, "Echo pulse width"=200, "Reserved"=0}, {"flags"=4, "Echo"=1, "Radial distance"=41.42, "Horizontal angle"=-0.5366887449882564, "Vertical angle"=0.020943951023931963, "Echo pulse width"=84, "Reserved"=0}, {"flags"=4, "Echo"=0, "Radial distance"=10.13, "Horizontal angle"=-0.5410520681182421, "Vertical angle"=-0.020943951023931952, "Echo pulse width"=348, "Reserved"=0}, {"flags"=4, "Echo"=0, "Radial distance"=13.49, "Horizontal angle"=-0.5410520681182421, "Vertical angle"=-0.006981317007977317, "Echo pulse width"=576, "Reserved"=0}, {"flags"=5, "Echo"=0, "Radial distance"=18.43, "Horizontal angle"=-0.5454153912482279, "Vertical angle"=0.00698131700797732, "Echo pulse width"=252, "Reserved"=0}, {"flags"=4, "Echo"=1, "Radial distance"=30.55, "Horizontal angle"=-0.5454153912482279, "Vertical angle"=0.00698131700797732, "Echo pulse width"=176, "Reserved"=0}, {"flags"=5, "Echo"=0, "Radial distance"=31.92, "Horizontal angle"=-0.5454153912482279, "Vertical angle"=0.020943951023931963, "Echo pulse width"=204, "Reserved"=0}, {"flags"=4, "Echo"=1, "Radial distance"=41.480000000000004, "Horizontal angle"=-0.5454153912482279, "Vertical angle"=0.020943951023931963, "Echo pulse width"=124, "Reserved"=0}, {"flags"=4, "Echo"=0, "Radial distance"=10.19, "Horizontal angle"=-0.5497787143782138, "Vertical angle"=-0.020943951023931952, "Echo pulse width"=296, "Reserved"=0}, {"flags"=4, "Echo"=0, "Radial distance"=14.120000000000001, "Horizontal angle"=-0.5497787143782138, "Vertical angle"=-0.006981317007977317, "Echo pulse width"=480, "Reserved"=0}, {"flags"=5, "Echo"=0, "Radial distance"=18.31, "Horizontal angle"=-0.5541420375081997, "Vertical angle"=0.00698131700797732, "Echo pulse width"=252, "Reserved"=0}, {"flags"=4, "Echo"=1, "Radial distance"=30.84, "Horizontal angle"=-0.5541420375081997, "Vertical angle"=0.00698131700797732, "Echo pulse width"=148, "Reserved"=0}, {"flags"=5, "Echo"=0, "Radial distance"=32.19, "Horizontal angle"=-0.5541420375081997, "Vertical angle"=0.020943951023931963, "Echo pulse width"=156, "Reserved"=0}, {"flags"=4, "Echo"=1, "Radial distance"=40.42, "Horizontal angle"=-0.5541420375081997, "Vertical angle"=0.020943951023931963, "Echo pulse width"=108, "Reserved"=0}, {"flags"=4, "Echo"=0, "Radial distance"=10.01, "Horizontal angle"=-0.5585053606381855, "Vertical angle"=-0.020943951023931952, "Echo pulse width"=344, "Reserved"=0}, {"flags"=5, "Echo"=0, "Radial distance"=13.17, "Horizontal angle"=-0.5585053606381855, "Vertical angle"=-0.006981317007977317, "Echo pulse width"=380, "Reserved"=0}, {"flags"=4, "Echo"=1, "Radial distance"=16.94, "Horizontal angle"=-0.5585053606381855, "Vertical angle"=-0.006981317007977317, "Echo pulse width"=160, "Reserved"=0}, {"flags"=4, "Echo"=0, "Radial distance"=16.67, "Horizontal angle"=-0.5628686837681712, "Vertical angle"=0.00698131700797732, "Echo pulse width"=364, "Reserved"=0}, {"flags"=0, "Echo"=0, "Radial distance"=16.37, "Horizontal angle"=-0.5628686837681712, "Vertical angle"=0.020943951023931963, "Echo pulse width"=188, "Reserved"=67}, {"flags"=4, "Echo"=0, "Radial distance"=10.19, "Horizontal angle"=-0.5672320068981571, "Vertical angle"=-0.020943951023931952, "Echo pulse width"=284, "Reserved"=0}, {"flags"=4, "Echo"=0, "Radial distance"=13.64, "Horizontal angle"=-0.5672320068981571, "Vertical angle"=-0.006981317007977317, "Echo pulse width"=476, "Reserved"=0}, {"flags"=0, "Echo"=0, "Radial distance"=16.39, "Horizontal angle"=-0.5715953300281429, "Vertical angle"=0.00698131700797732, "Echo pulse width"=196, "Reserved"=67}, {"flags"=0, "Echo"=0, "Radial distance"=16.17, "Horizontal angle"=-0.5715953300281429, "Vertical angle"=0.020943951023931963, "Echo pulse width"=188, "Reserved"=67}, {"flags"=4, "Echo"=0, "Radial distance"=9.99, "Horizontal angle"=-0.5759586531581287, "Vertical angle"=-0.020943951023931952, "Echo pulse width"=336, "Reserved"=0}, {"flags"=5, "Echo"=0, "Radial distance"=13.05, "Horizontal angle"=-0.5759586531581287, "Vertical angle"=-0.006981317007977317, "Echo pulse width"=336, "Reserved"=0}, {"flags"=0, "Echo"=1, "Radial distance"=16.38, "Horizontal angle"=-0.5759586531581287, "Vertical angle"=-0.006981317007977317, "Echo pulse width"=160, "Reserved"=67}, {"flags"=0, "Echo"=0, "Radial distance"=16.23, "Horizontal angle"=-0.5803219762881145, "Vertical angle"=0.00698131700797732, "Echo pulse width"=192, "Reserved"=67}, {"flags"=0, "Echo"=0, "Radial distance"=16.01, "Horizontal angle"=-0.5803219762881145, "Vertical angle"=0.020943951023931963, "Echo pulse width"=184, "Reserved"=67}, {"flags"=4, "Echo"=0, "Radial distance"=9.99, "Horizontal angle"=-0.5846852994181004, "Vertical angle"=-0.020943951023931952, "Echo pulse width"=288, "Reserved"=0}, {"flags"=4, "Echo"=0, "Radial distance"=13.32, "Horizontal angle"=-0.5846852994181004, "Vertical angle"=-0.006981317007977317, "Echo pulse width"=460, "Reserved"=0}, {"flags"=0, "Echo"=0, "Radial distance"=16.240000000000002, "Horizontal angle"=-0.5890486225480862, "Vertical angle"=0.00698131700797732, "Echo pulse width"=188, "Reserved"=67}, {"flags"=0, "Echo"=0, "Radial distance"=15.97, "Horizontal angle"=-0.5890486225480862, "Vertical angle"=0.020943951023931963, "Echo pulse width"=188, "Reserved"=67}, {"flags"=4, "Echo"=0, "Radial distance"=9.77, "Horizontal angle"=-0.593411945678072, "Vertical angle"=-0.020943951023931952, "Echo pulse width"=344, "Reserved"=0}, {"flags"=4, "Echo"=0, "Radial distance"=12.81, "Horizontal angle"=-0.593411945678072, "Vertical angle"=-0.006981317007977317, "Echo pulse width"=492, "Reserved"=0}, {"flags"=0, "Echo"=0, "Radial distance"=16.16, "Horizontal angle"=-0.5977752688080579, "Vertical angle"=0.00698131700797732, "Echo pulse width"=184, "Reserved"=67}, {"flags"=0, "Echo"=0, "Radial distance"=15.97, "Horizontal angle"=-0.5977752688080579, "Vertical angle"=0.020943951023931963, "Echo pulse width"=188, "Reserved"=67}, {"flags"=4, "Echo"=0, "Radial distance"=9.83, "Horizontal angle"=-0.6021385919380438, "Vertical angle"=-0.020943951023931952, "Echo pulse width"=284, "Reserved"=0}, {"flags"=4, "Echo"=0, "Radial distance"=12.96, "Horizontal angle"=-0.6021385919380438, "Vertical angle"=-0.006981317007977317, "Echo pulse width"=456, "Reserved"=0}, {"flags"=0, "Echo"=0, "Radial distance"=16.23, "Horizontal angle"=-0.6065019150680295, "Vertical angle"=0.00698131700797732, "Echo pulse width"=192, "Reserved"=67}, {"flags"=0, "Echo"=0, "Radial distance"=16.05, "Horizontal angle"=-0.6065019150680295, "Vertical angle"=0.020943951023931963, "Echo pulse width"=188, "Reserved"=67}, {"flags"=4, "Echo"=0, "Radial distance"=9.67, "Horizontal angle"=-0.6108652381980153, "Vertical angle"=-0.020943951023931952, "Echo pulse width"=340, "Reserved"=0}, {"flags"=4, "Echo"=0, "Radial distance"=12.69, "Horizontal angle"=-0.6108652381980153, "Vertical angle"=-0.006981317007977317, "Echo pulse width"=480, "Reserved"=0}, {"flags"=0, "Echo"=0, "Radial distance"=16.240000000000002, "Horizontal angle"=-0.6152285613280012, "Vertical angle"=0.00698131700797732, "Echo pulse width"=188, "Reserved"=67}, {"flags"=0, "Echo"=0, "Radial distance"=16.04, "Horizontal angle"=-0.6152285613280012, "Vertical angle"=0.020943951023931963, "Echo pulse width"=180, "Reserved"=67}, {"flags"=4, "Echo"=0, "Radial distance"=9.790000000000001, "Horizontal angle"=-0.619591884457987, "Vertical angle"=-0.020943951023931952, "Echo pulse width"=284, "Reserved"=0}, {"flags"=4, "Echo"=0, "Radial distance"=12.84, "Horizontal angle"=-0.619591884457987, "Vertical angle"=-0.006981317007977317, "Echo pulse width"=440, "Reserved"=0}, {"flags"=0, "Echo"=0, "Radial distance"=16.39, "Horizontal angle"=-0.6239552075879727, "Vertical angle"=0.00698131700797732, "Echo pulse width"=192, "Reserved"=67}, {"flags"=0, "Echo"=0, "Radial distance"=16.17, "Horizontal angle"=-0.6239552075879727, "Vertical angle"=0.020943951023931963, "Echo pulse width"=184, "Reserved"=67}, {"flags"=4, "Echo"=0, "Radial distance"=9.59, "Horizontal angle"=-0.6283185307179586, "Vertical angle"=-0.020943951023931952, "Echo pulse width"=340, "Reserved"=0}, {"flags"=4, "Echo"=0, "Radial distance"=12.61, "Horizontal angle"=-0.6283185307179586, "Vertical angle"=-0.006981317007977317, "Echo pulse width"=468, "Reserved"=0}, {"flags"=5, "Echo"=0, "Radial distance"=17.150000000000002, "Horizontal angle"=-0.6326818538479445, "Vertical angle"=0.00698131700797732, "Echo pulse width"=380, "Reserved"=0}, {"flags"=4, "Echo"=1, "Radial distance"=26.13, "Horizontal angle"=-0.6326818538479445, "Vertical angle"=0.00698131700797732, "Echo pulse width"=88, "Reserved"=0}, {"flags"=0, "Echo"=0, "Radial distance"=16.36, "Horizontal angle"=-0.6326818538479445, "Vertical angle"=0.020943951023931963, "Echo pulse width"=180, "Reserved"=67}, {"flags"=4, "Echo"=0, "Radial distance"=9.67, "Horizontal angle"=-0.6370451769779303, "Vertical angle"=-0.020943951023931952, "Echo pulse width"=300, "Reserved"=0}, {"flags"=4, "Echo"=0, "Radial distance"=12.72, "Horizontal angle"=-0.6370451769779303, "Vertical angle"=-0.006981317007977317, "Echo pulse width"=432, "Reserved"=0}, {"flags"=5, "Echo"=0, "Radial distance"=16.990000000000002, "Horizontal angle"=-0.6414085001079161, "Vertical angle"=0.00698131700797732, "Echo pulse width"=288, "Reserved"=0}, {"flags"=4, "Echo"=1, "Radial distance"=25.72, "Horizontal angle"=-0.6414085001079161, "Vertical angle"=0.00698131700797732, "Echo pulse width"=60, "Reserved"=0}, {"flags"=4, "Echo"=0, "Radial distance"=9.450000000000001, "Horizontal angle"=-0.6457718232379019, "Vertical angle"=-0.020943951023931952, "Echo pulse width"=352, "Reserved"=0}, {"flags"=4, "Echo"=0, "Radial distance"=12.49, "Horizontal angle"=-0.6457718232379019, "Vertical angle"=-0.006981317007977317, "Echo pulse width"=456, "Reserved"=0}, {"flags"=5, "Echo"=0, "Radial distance"=16.87, "Horizontal angle"=-0.6501351463678877, "Vertical angle"=0.00698131700797732, "Echo pulse width"=384, "Reserved"=0}, {"flags"=5, "Echo"=1, "Radial distance"=25.48, "Horizontal angle"=-0.6501351463678877, "Vertical angle"=0.00698131700797732, "Echo pulse width"=68, "Reserved"=0}, {"flags"=4, "Echo"=2, "Radial distance"=26.84, "Horizontal angle"=-0.6501351463678877, "Vertical angle"=0.00698131700797732, "Echo pulse width"=84, "Reserved"=0}, {"flags"=4, "Echo"=0, "Radial distance"=9.55, "Horizontal angle"=-0.6544984694978736, "Vertical angle"=-0.020943951023931952, "Echo pulse width"=300, "Reserved"=0}, {"flags"=4, "Echo"=0, "Radial distance"=12.64, "Horizontal angle"=-0.6544984694978736, "Vertical angle"=-0.006981317007977317, "Echo pulse width"=424, "Reserved"=0}, {"flags"=4, "Echo"=0, "Radial distance"=16.55, "Horizontal angle"=-0.6588617926278594, "Vertical angle"=0.00698131700797732, "Echo pulse width"=424, "Reserved"=0}, {"flags"=4, "Echo"=0, "Radial distance"=9.33, "Horizontal angle"=-0.6632251157578453, "Vertical angle"=-0.020943951023931952, "Echo pulse width"=352, "Reserved"=0}, {"flags"=4, "Echo"=0, "Radial distance"=12.290000000000001, "Horizontal angle"=-0.6632251157578453, "Vertical angle"=-0.006981317007977317, "Echo pulse width"=448, "Reserved"=0}, {"flags"=4, "Echo"=0, "Radial distance"=16.55, "Horizontal angle"=-0.667588438887831, "Vertical angle"=0.00698131700797732, "Echo pulse width"=396, "Reserved"=0}, {"flags"=0, "Echo"=0, "Radial distance"=76.51, "Horizontal angle"=-0.667588438887831, "Vertical angle"=0.020943951023931963, "Echo pulse width"=96, "Reserved"=68}, {"flags"=4, "Echo"=0, "Radial distance"=9.47, "Horizontal angle"=-0.6719517620178168, "Vertical angle"=-0.020943951023931952, "Echo pulse width"=296, "Reserved"=0}, {"flags"=4, "Echo"=0, "Radial distance"=12.48, "Horizontal angle"=-0.6719517620178168, "Vertical angle"=-0.006981317007977317, "Echo pulse width"=396, "Reserved"=0}, {"flags"=4, "Echo"=0, "Radial distance"=16.31, "Horizontal angle"=-0.6763150851478027, "Vertical angle"=0.00698131700797732, "Echo pulse width"=388, "Reserved"=0}, {"flags"=0, "Echo"=0, "Radial distance"=84.49, "Horizontal angle"=-0.6763150851478027, "Vertical angle"=0.020943951023931963, "Echo pulse width"=72, "Reserved"=69}, {"flags"=4, "Echo"=0, "Radial distance"=9.290000000000001, "Horizontal angle"=-0.6806784082777886, "Vertical angle"=-0.020943951023931952, "Echo pulse width"=344, "Reserved"=0}, {"flags"=4, "Echo"=0, "Radial distance"=12.25, "Horizontal angle"=-0.6806784082777886, "Vertical angle"=-0.006981317007977317, "Echo pulse width"=424, "Reserved"=0}, {"flags"=4, "Echo"=0, "Radial distance"=15.99, "Horizontal angle"=-0.6850417314077744, "Vertical angle"=0.00698131700797732, "Echo pulse width"=432, "Reserved"=0}, {"flags"=4, "Echo"=0, "Radial distance"=9.35, "Horizontal angle"=-0.6894050545377601, "Vertical angle"=-0.020943951023931952, "Echo pulse width"=296, "Reserved"=0}, {"flags"=4, "Echo"=0, "Radial distance"=12.48, "Horizontal angle"=-0.6894050545377601, "Vertical angle"=-0.006981317007977317, "Echo pulse width"=380, "Reserved"=0}, {"flags"=5, "Echo"=0, "Radial distance"=15.870000000000001, "Horizontal angle"=-0.6937683776677459, "Vertical angle"=0.00698131700797732, "Echo pulse width"=400, "Reserved"=0}, {"flags"=4, "Echo"=1, "Radial distance"=21.39, "Horizontal angle"=-0.6937683776677459, "Vertical angle"=0.00698131700797732, "Echo pulse width"=108, "Reserved"=0}, {"flags"=4, "Echo"=0, "Radial distance"=9.19, "Horizontal angle"=-0.6981317007977318, "Vertical angle"=-0.020943951023931952, "Echo pulse width"=332, "Reserved"=0}, {"flags"=4, "Echo"=0, "Radial distance"=12.09, "Horizontal angle"=-0.6981317007977318, "Vertical angle"=-0.006981317007977317, "Echo pulse width"=416, "Reserved"=0}, {"flags"=4, "Echo"=0, "Radial distance"=15.75, "Horizontal angle"=-0.7024950239277177, "Vertical angle"=0.00698131700797732, "Echo pulse width"=412, "Reserved"=0}, {"flags"=4, "Echo"=0, "Radial distance"=9.19, "Horizontal angle"=-0.7068583470577035, "Vertical angle"=-0.020943951023931952, "Echo pulse width"=292, "Reserved"=0}, {"flags"=4, "Echo"=0, "Radial distance"=12.24, "Horizontal angle"=-0.7068583470577035, "Vertical angle"=-0.006981317007977317, "Echo pulse width"=372, "Reserved"=0}, {"flags"=5, "Echo"=0, "Radial distance"=15.67, "Horizontal angle"=-0.7112216701876892, "Vertical angle"=0.00698131700797732, "Echo pulse width"=384, "Reserved"=0}, {"flags"=5, "Echo"=1, "Radial distance"=21.22, "Horizontal angle"=-0.7112216701876892, "Vertical angle"=0.00698131700797732, "Echo pulse width"=36, "Reserved"=0}, {"flags"=4, "Echo"=2, "Radial distance"=25.09, "Horizontal angle"=-0.7112216701876892, "Vertical angle"=0.00698131700797732, "Echo pulse width"=112, "Reserved"=0}, {"flags"=4, "Echo"=0, "Radial distance"=9.07, "Horizontal angle"=-0.7155849933176751, "Vertical angle"=-0.020943951023931952, "Echo pulse width"=332, "Reserved"=0}, {"flags"=4, "Echo"=0, "Radial distance"=11.85, "Horizontal angle"=-0.7155849933176751, "Vertical angle"=-0.006981317007977317, "Echo pulse width"=412, "Reserved"=0}, {"flags"=5, "Echo"=0, "Radial distance"=15.39, "Horizontal angle"=-0.7199483164476609, "Vertical angle"=0.00698131700797732, "Echo pulse width"=352, "Reserved"=0}, {"flags"=4, "Echo"=1, "Radial distance"=24.77, "Horizontal angle"=-0.7199483164476609, "Vertical angle"=0.00698131700797732, "Echo pulse width"=156, "Reserved"=0}, {"flags"=4, "Echo"=0, "Radial distance"=25.89, "Horizontal angle"=-0.7199483164476609, "Vertical angle"=0.020943951023931963, "Echo pulse width"=72, "Reserved"=0}, {"flags"=4, "Echo"=0, "Radial distance"=9.07, "Horizontal angle"=-0.7243116395776468, "Vertical angle"=-0.020943951023931952, "Echo pulse width"=288, "Reserved"=0}, {"flags"=4, "Echo"=0, "Radial distance"=12.120000000000001, "Horizontal angle"=-0.7243116395776468, "Vertical angle"=-0.006981317007977317, "Echo pulse width"=360, "Reserved"=0}, {"flags"=5, "Echo"=0, "Radial distance"=15.11, "Horizontal angle"=-0.7286749627076325, "Vertical angle"=0.00698131700797732, "Echo pulse width"=376, "Reserved"=0}, {"flags"=5, "Echo"=1, "Radial distance"=21.26, "Horizontal angle"=-0.7286749627076325, "Vertical angle"=0.00698131700797732, "Echo pulse width"=36, "Reserved"=0}, {"flags"=4, "Echo"=2, "Radial distance"=24.35, "Horizontal angle"=-0.7286749627076325, "Vertical angle"=0.00698131700797732, "Echo pulse width"=136, "Reserved"=0}, {"flags"=4, "Echo"=0, "Radial distance"=25.76, "Horizontal angle"=-0.7286749627076325, "Vertical angle"=0.020943951023931963, "Echo pulse width"=192, "Reserved"=0}, {"flags"=4, "Echo"=0, "Radial distance"=8.950000000000001, "Horizontal angle"=-0.7330382858376184, "Vertical angle"=-0.020943951023931952, "Echo pulse width"=332, "Reserved"=0}, {"flags"=4, "Echo"=0, "Radial distance"=11.85, "Horizontal angle"=-0.7330382858376184, "Vertical angle"=-0.006981317007977317, "Echo pulse width"=392, "Reserved"=0}, {"flags"=5, "Echo"=0, "Radial distance"=15.15, "Horizontal angle"=-0.7374016089676042, "Vertical angle"=0.00698131700797732, "Echo pulse width"=368, "Reserved"=0}, {"flags"=5, "Echo"=1, "Radial distance"=19.61, "Horizontal angle"=-0.7374016089676042, "Vertical angle"=0.00698131700797732, "Echo pulse width"=92, "Reserved"=0}, {"flags"=4, "Echo"=2, "Radial distance"=24.13, "Horizontal angle"=-0.7374016089676042, "Vertical angle"=0.00698131700797732, "Echo pulse width"=124, "Reserved"=0}, {"flags"=4, "Echo"=0, "Radial distance"=25.240000000000002, "Horizontal angle"=-0.7374016089676042, "Vertical angle"=0.020943951023931963, "Echo pulse width"=252, "Reserved"=0}, {"flags"=4, "Echo"=0, "Radial distance"=8.950000000000001, "Horizontal angle"=-0.74176493209759, "Vertical angle"=-0.020943951023931952, "Echo pulse width"=284, "Reserved"=0}, {"flags"=4, "Echo"=0, "Radial distance"=11.92, "Horizontal angle"=-0.74176493209759, "Vertical angle"=-0.006981317007977317, "Echo pulse width"=348, "Reserved"=0}, {"flags"=5, "Echo"=0, "Radial distance"=14.870000000000001, "Horizontal angle"=-0.7461282552275759, "Vertical angle"=0.00698131700797732, "Echo pulse width"=376, "Reserved"=0}, {"flags"=5, "Echo"=1, "Radial distance"=19.37, "Horizontal angle"=-0.7461282552275759, "Vertical angle"=0.00698131700797732, "Echo pulse width"=124, "Reserved"=0}, {"flags"=4, "Echo"=2, "Radial distance"=23.97, "Horizontal angle"=-0.7461282552275759, "Vertical angle"=0.00698131700797732, "Echo pulse width"=120, "Reserved"=0}, {"flags"=4, "Echo"=0, "Radial distance"=24.92, "Horizontal angle"=-0.7461282552275759, "Vertical angle"=0.020943951023931963, "Echo pulse width"=276, "Reserved"=0}, {"flags"=4, "Echo"=0, "Radial distance"=8.83, "Horizontal angle"=-0.7504915783575618, "Vertical angle"=-0.020943951023931952, "Echo pulse width"=324, "Reserved"=0}, {"flags"=4, "Echo"=0, "Radial distance"=11.65, "Horizontal angle"=-0.7504915783575618, "Vertical angle"=-0.006981317007977317, "Echo pulse width"=368, "Reserved"=0}, {"flags"=5, "Echo"=0, "Radial distance"=14.790000000000001, "Horizontal angle"=-0.7548549014875475, "Vertical angle"=0.00698131700797732, "Echo pulse width"=392, "Reserved"=0}, {"flags"=5, "Echo"=1, "Radial distance"=19.07, "Horizontal angle"=-0.7548549014875475, "Vertical angle"=0.00698131700797732, "Echo pulse width"=104, "Reserved"=0}, {"flags"=4, "Echo"=2, "Radial distance"=23.75, "Horizontal angle"=-0.7548549014875475, "Vertical angle"=0.00698131700797732, "Echo pulse width"=108, "Reserved"=0}, {"flags"=4, "Echo"=0, "Radial distance"=24.63, "Horizontal angle"=-0.7548549014875475, "Vertical angle"=0.020943951023931963, "Echo pulse width"=236, "Reserved"=0}, {"flags"=4, "Echo"=0, "Radial distance"=8.870000000000001, "Horizontal angle"=-0.7592182246175333, "Vertical angle"=-0.020943951023931952, "Echo pulse width"=280, "Reserved"=0}, {"flags"=4, "Echo"=0, "Radial distance"=11.790000000000001, "Horizontal angle"=-0.7592182246175333, "Vertical angle"=-0.006981317007977317, "Echo pulse width"=296, "Reserved"=0}, {"flags"=5, "Echo"=0, "Radial distance"=14.64, "Horizontal angle"=-0.7635815477475192, "Vertical angle"=0.00698131700797732, "Echo pulse width"=352, "Reserved"=0}, {"flags"=5, "Echo"=1, "Radial distance"=19.36, "Horizontal angle"=-0.7635815477475192, "Vertical angle"=0.00698131700797732, "Echo pulse width"=208, "Reserved"=0}, {"flags"=4, "Echo"=2, "Radial distance"=23.62, "Horizontal angle"=-0.7635815477475192, "Vertical angle"=0.00698131700797732, "Echo pulse width"=100, "Reserved"=0}, {"flags"=1, "Echo"=0, "Radial distance"=12.46, "Horizontal angle"=-0.7635815477475192, "Vertical angle"=0.020943951023931963, "Echo pulse width"=140, "Reserved"=70}, {"flags"=4, "Echo"=1, "Radial distance"=24.11, "Horizontal angle"=-0.7635815477475192, "Vertical angle"=0.020943951023931963, "Echo pulse width"=160, "Reserved"=0}, {"flags"=4, "Echo"=0, "Radial distance"=8.71, "Horizontal angle"=-0.767944870877505, "Vertical angle"=-0.020943951023931952, "Echo pulse width"=328, "Reserved"=0}, {"flags"=4, "Echo"=0, "Radial distance"=11.48, "Horizontal angle"=-0.767944870877505, "Vertical angle"=-0.006981317007977317, "Echo pulse width"=320, "Reserved"=0}, {"flags"=1, "Echo"=0, "Radial distance"=12.43, "Horizontal angle"=-0.7723081940074907, "Vertical angle"=0.00698131700797732, "Echo pulse width"=196, "Reserved"=70}, {"flags"=4, "Echo"=1, "Radial distance"=16.14, "Horizontal angle"=-0.7723081940074907, "Vertical angle"=0.00698131700797732, "Echo pulse width"=100, "Reserved"=0}, {"flags"=0, "Echo"=0, "Radial distance"=12.25, "Horizontal angle"=-0.7723081940074907, "Vertical angle"=0.020943951023931963, "Echo pulse width"=188, "Reserved"=70}, {"flags"=4, "Echo"=0, "Radial distance"=8.870000000000001, "Horizontal angle"=-0.7766715171374766, "Vertical angle"=-0.020943951023931952, "Echo pulse width"=276, "Reserved"=0}, {"flags"=4, "Echo"=0, "Radial distance"=11.790000000000001, "Horizontal angle"=-0.7766715171374766, "Vertical angle"=-0.006981317007977317, "Echo pulse width"=256, "Reserved"=0}, {"flags"=0, "Echo"=0, "Radial distance"=12.33, "Horizontal angle"=-0.7810348402674625, "Vertical angle"=0.00698131700797732, "Echo pulse width"=168, "Reserved"=70}, {"flags"=0, "Echo"=0, "Radial distance"=12.15, "Horizontal angle"=-0.7810348402674625, "Vertical angle"=0.020943951023931963, "Echo pulse width"=164, "Reserved"=70}, {"flags"=4, "Echo"=0, "Radial distance"=8.59, "Horizontal angle"=-0.7853981633974483, "Vertical angle"=-0.020943951023931952, "Echo pulse width"=332, "Reserved"=0}, {"flags"=4, "Echo"=0, "Radial distance"=11.32, "Horizontal angle"=-0.7853981633974483, "Vertical angle"=-0.006981317007977317, "Echo pulse width"=304, "Reserved"=0}, {"flags"=0, "Echo"=0, "Radial distance"=12.27, "Horizontal angle"=-0.789761486527434, "Vertical angle"=0.00698131700797732, "Echo pulse width"=192, "Reserved"=70}, {"flags"=0, "Echo"=0, "Radial distance"=12.08, "Horizontal angle"=-0.789761486527434, "Vertical angle"=0.020943951023931963, "Echo pulse width"=192, "Reserved"=70}, {"flags"=4, "Echo"=0, "Radial distance"=8.67, "Horizontal angle"=-0.7941248096574199, "Vertical angle"=-0.020943951023931952, "Echo pulse width"=276, "Reserved"=0}, {"flags"=4, "Echo"=0, "Radial distance"=11.5, "Horizontal angle"=-0.7941248096574199, "Vertical angle"=-0.006981317007977317, "Echo pulse width"=248, "Reserved"=0}, {"flags"=0, "Echo"=0, "Radial distance"=12.15, "Horizontal angle"=-0.7984881327874057, "Vertical angle"=0.00698131700797732, "Echo pulse width"=164, "Reserved"=70}, {"flags"=0, "Echo"=0, "Radial distance"=11.99, "Horizontal angle"=-0.7984881327874057, "Vertical angle"=0.020943951023931963, "Echo pulse width"=168, "Reserved"=70}, {"flags"=4, "Echo"=0, "Radial distance"=8.47, "Horizontal angle"=-0.8028514559173915, "Vertical angle"=-0.020943951023931952, "Echo pulse width"=324, "Reserved"=0}, {"flags"=4, "Echo"=0, "Radial distance"=11.16, "Horizontal angle"=-0.8028514559173915, "Vertical angle"=-0.006981317007977317, "Echo pulse width"=284, "Reserved"=0}, {"flags"=0, "Echo"=0, "Radial distance"=12.11, "Horizontal angle"=-0.8072147790473774, "Vertical angle"=0.00698131700797732, "Echo pulse width"=192, "Reserved"=70}, {"flags"=0, "Echo"=0, "Radial distance"=11.89, "Horizontal angle"=-0.8072147790473774, "Vertical angle"=0.020943951023931963, "Echo pulse width"=188, "Reserved"=70}, {"flags"=4, "Echo"=0, "Radial distance"=8.63, "Horizontal angle"=-0.8115781021773633, "Vertical angle"=-0.020943951023931952, "Echo pulse width"=276, "Reserved"=0}, {"flags"=4, "Echo"=0, "Radial distance"=11.33, "Horizontal angle"=-0.8115781021773633, "Vertical angle"=-0.006981317007977317, "Echo pulse width"=236, "Reserved"=0}, {"flags"=0, "Echo"=0, "Radial distance"=12.07, "Horizontal angle"=-0.8159414253073491, "Vertical angle"=0.00698131700797732, "Echo pulse width"=164, "Reserved"=70}, {"flags"=0, "Echo"=0, "Radial distance"=11.870000000000001, "Horizontal angle"=-0.8159414253073491, "Vertical angle"=0.020943951023931963, "Echo pulse width"=160, "Reserved"=70}, {"flags"=4, "Echo"=0, "Radial distance"=8.47, "Horizontal angle"=-0.8203047484373349, "Vertical angle"=-0.020943951023931952, "Echo pulse width"=312, "Reserved"=0}, {"flags"=4, "Echo"=0, "Radial distance"=11.120000000000001, "Horizontal angle"=-0.8203047484373349, "Vertical angle"=-0.006981317007977317, "Echo pulse width"=264, "Reserved"=0}, {"flags"=0, "Echo"=0, "Radial distance"=11.96, "Horizontal angle"=-0.8246680715673207, "Vertical angle"=0.00698131700797732, "Echo pulse width"=184, "Reserved"=70}, {"flags"=0, "Echo"=0, "Radial distance"=11.92, "Horizontal angle"=-0.8246680715673207, "Vertical angle"=0.020943951023931963, "Echo pulse width"=200, "Reserved"=70}, {"flags"=4, "Echo"=0, "Radial distance"=8.59, "Horizontal angle"=-0.8290313946973066, "Vertical angle"=-0.020943951023931952, "Echo pulse width"=264, "Reserved"=0}, {"flags"=4, "Echo"=0, "Radial distance"=11.33, "Horizontal angle"=-0.8290313946973066, "Vertical angle"=-0.006981317007977317, "Echo pulse width"=220, "Reserved"=0}, {"flags"=0, "Echo"=0, "Radial distance"=12.030000000000001, "Horizontal angle"=-0.8333947178272924, "Vertical angle"=0.00698131700797732, "Echo pulse width"=164, "Reserved"=70}, {"flags"=0, "Echo"=0, "Radial distance"=11.870000000000001, "Horizontal angle"=-0.8333947178272924, "Vertical angle"=0.020943951023931963, "Echo pulse width"=160, "Reserved"=70}, {"flags"=4, "Echo"=0, "Radial distance"=8.43, "Horizontal angle"=-0.8377580409572781, "Vertical angle"=-0.020943951023931952, "Echo pulse width"=304, "Reserved"=0}, {"flags"=4, "Echo"=0, "Radial distance"=11.0, "Horizontal angle"=-0.8377580409572781, "Vertical angle"=-0.006981317007977317, "Echo pulse width"=256, "Reserved"=0}, {"flags"=0, "Echo"=0, "Radial distance"=12.040000000000001, "Horizontal angle"=-0.842121364087264, "Vertical angle"=0.00698131700797732, "Echo pulse width"=184, "Reserved"=70}, {"flags"=0, "Echo"=0, "Radial distance"=11.89, "Horizontal angle"=-0.842121364087264, "Vertical angle"=0.020943951023931963, "Echo pulse width"=188, "Reserved"=70}, {"flags"=4, "Echo"=0, "Radial distance"=8.51, "Horizontal angle"=-0.8464846872172498, "Vertical angle"=-0.020943951023931952, "Echo pulse width"=256, "Reserved"=0}, {"flags"=4, "Echo"=0, "Radial distance"=11.24, "Horizontal angle"=-0.8464846872172498, "Vertical angle"=-0.006981317007977317, "Echo pulse width"=212, "Reserved"=0}, {"flags"=0, "Echo"=0, "Radial distance"=12.09, "Horizontal angle"=-0.8508480103472356, "Vertical angle"=0.00698131700797732, "Echo pulse width"=168, "Reserved"=70}, {"flags"=0, "Echo"=0, "Radial distance"=11.91, "Horizontal angle"=-0.8508480103472356, "Vertical angle"=0.020943951023931963, "Echo pulse width"=164, "Reserved"=70}, {"flags"=4, "Echo"=0, "Radial distance"=8.31, "Horizontal angle"=-0.8552113334772213, "Vertical angle"=-0.020943951023931952, "Echo pulse width"=308, "Reserved"=0}, {"flags"=4, "Echo"=0, "Radial distance"=10.84, "Horizontal angle"=-0.8552113334772213, "Vertical angle"=-0.006981317007977317, "Echo pulse width"=264, "Reserved"=0}, {"flags"=0, "Echo"=0, "Radial distance"=12.14, "Horizontal angle"=-0.8595746566072073, "Vertical angle"=0.00698131700797732, "Echo pulse width"=200, "Reserved"=70}, {"flags"=0, "Echo"=0, "Radial distance"=11.97, "Horizontal angle"=-0.8595746566072073, "Vertical angle"=0.020943951023931963, "Echo pulse width"=184, "Reserved"=70}, {"flags"=4, "Echo"=0, "Radial distance"=8.51, "Horizontal angle"=-0.8639379797371932, "Vertical angle"=-0.020943951023931952, "Echo pulse width"=240, "Reserved"=0}, {"flags"=4, "Echo"=0, "Radial distance"=11.34, "Horizontal angle"=-0.8639379797371932, "Vertical angle"=-0.006981317007977317, "Echo pulse width"=176, "Reserved"=0}, {"flags"=0, "Echo"=0, "Radial distance"=12.290000000000001, "Horizontal angle"=-0.868301302867179, "Vertical angle"=0.00698131700797732, "Echo pulse width"=176, "Reserved"=70}, {"flags"=0, "Echo"=0, "Radial distance"=12.19, "Horizontal angle"=-0.868301302867179, "Vertical angle"=0.020943951023931963, "Echo pulse width"=160, "Reserved"=70}]} {"hash" format="%016x"}
  out "GGA_2":T25={"hash"=1114363806672425932, "sys time"=0, "time"=0.0, "x"=0.0, "y"=0.0, "h"=0.0, "numSV"=0, "postype"=0, "lag"=0, "hordev"=0.0, "lat"=0.0, "lon"=0.0, "hgt"=0.0, "map_idx"=0} {"hash" format="%016x"}
  out "RMC_2":T26={"hash"=2469426948741950939, "sys time"=0, "time"=0.0, "speed"=0.0, "heading"=0.0, "lat"=0.0, "lon"=0.0} {"hash" format="%016x"}
  out "CON_T":T27={"hash"=4999688090526594712, "sys time"=0, "Auto"=FALSE, "Run"=FALSE, "Solenoid"=FALSE, "T lim"=FALSE, "brk_enc"=0, "B PWM"=0, "T PWM"=0, "ref_vel"=0.0, "ref_bkr_enc"=0.0, "ref_apv"=0.0, "ref_steer"=0.0} {"hash" format="%016x"}
  out "EYE_RAW_T":T28={"hash"=-8920902524919788889, "sys time"=0, "mobileye"=[]} {"hash" format="%016x"}
  out "POS_T":T2={"hash"=8611666821338907869, "sys time"=0, "dt"=0.0, "x"=0.0, "y"=0.0, "speed"=0.0, "heading"=0.0, "yaw_rate"=0.0} {"hash" format="%016x"}
  out "GGA_1":T25={"hash"=1114363806672425932, "sys time"=0, "time"=0.0, "x"=0.0, "y"=0.0, "h"=0.0, "numSV"=0, "postype"=0, "lag"=0, "hordev"=0.0, "lat"=0.0, "lon"=0.0, "hgt"=0.0, "map_idx"=0} {"hash" format="%016x"}
  out "RMC_1":T26={"hash"=2469426948741950939, "sys time"=0, "time"=0.0, "speed"=0.0, "heading"=0.0, "lat"=0.0, "lon"=0.0} {"hash" format="%016x"}
  out "LCM":T9={"connection ID"=refnum, "net address"=0, "port"=7667}
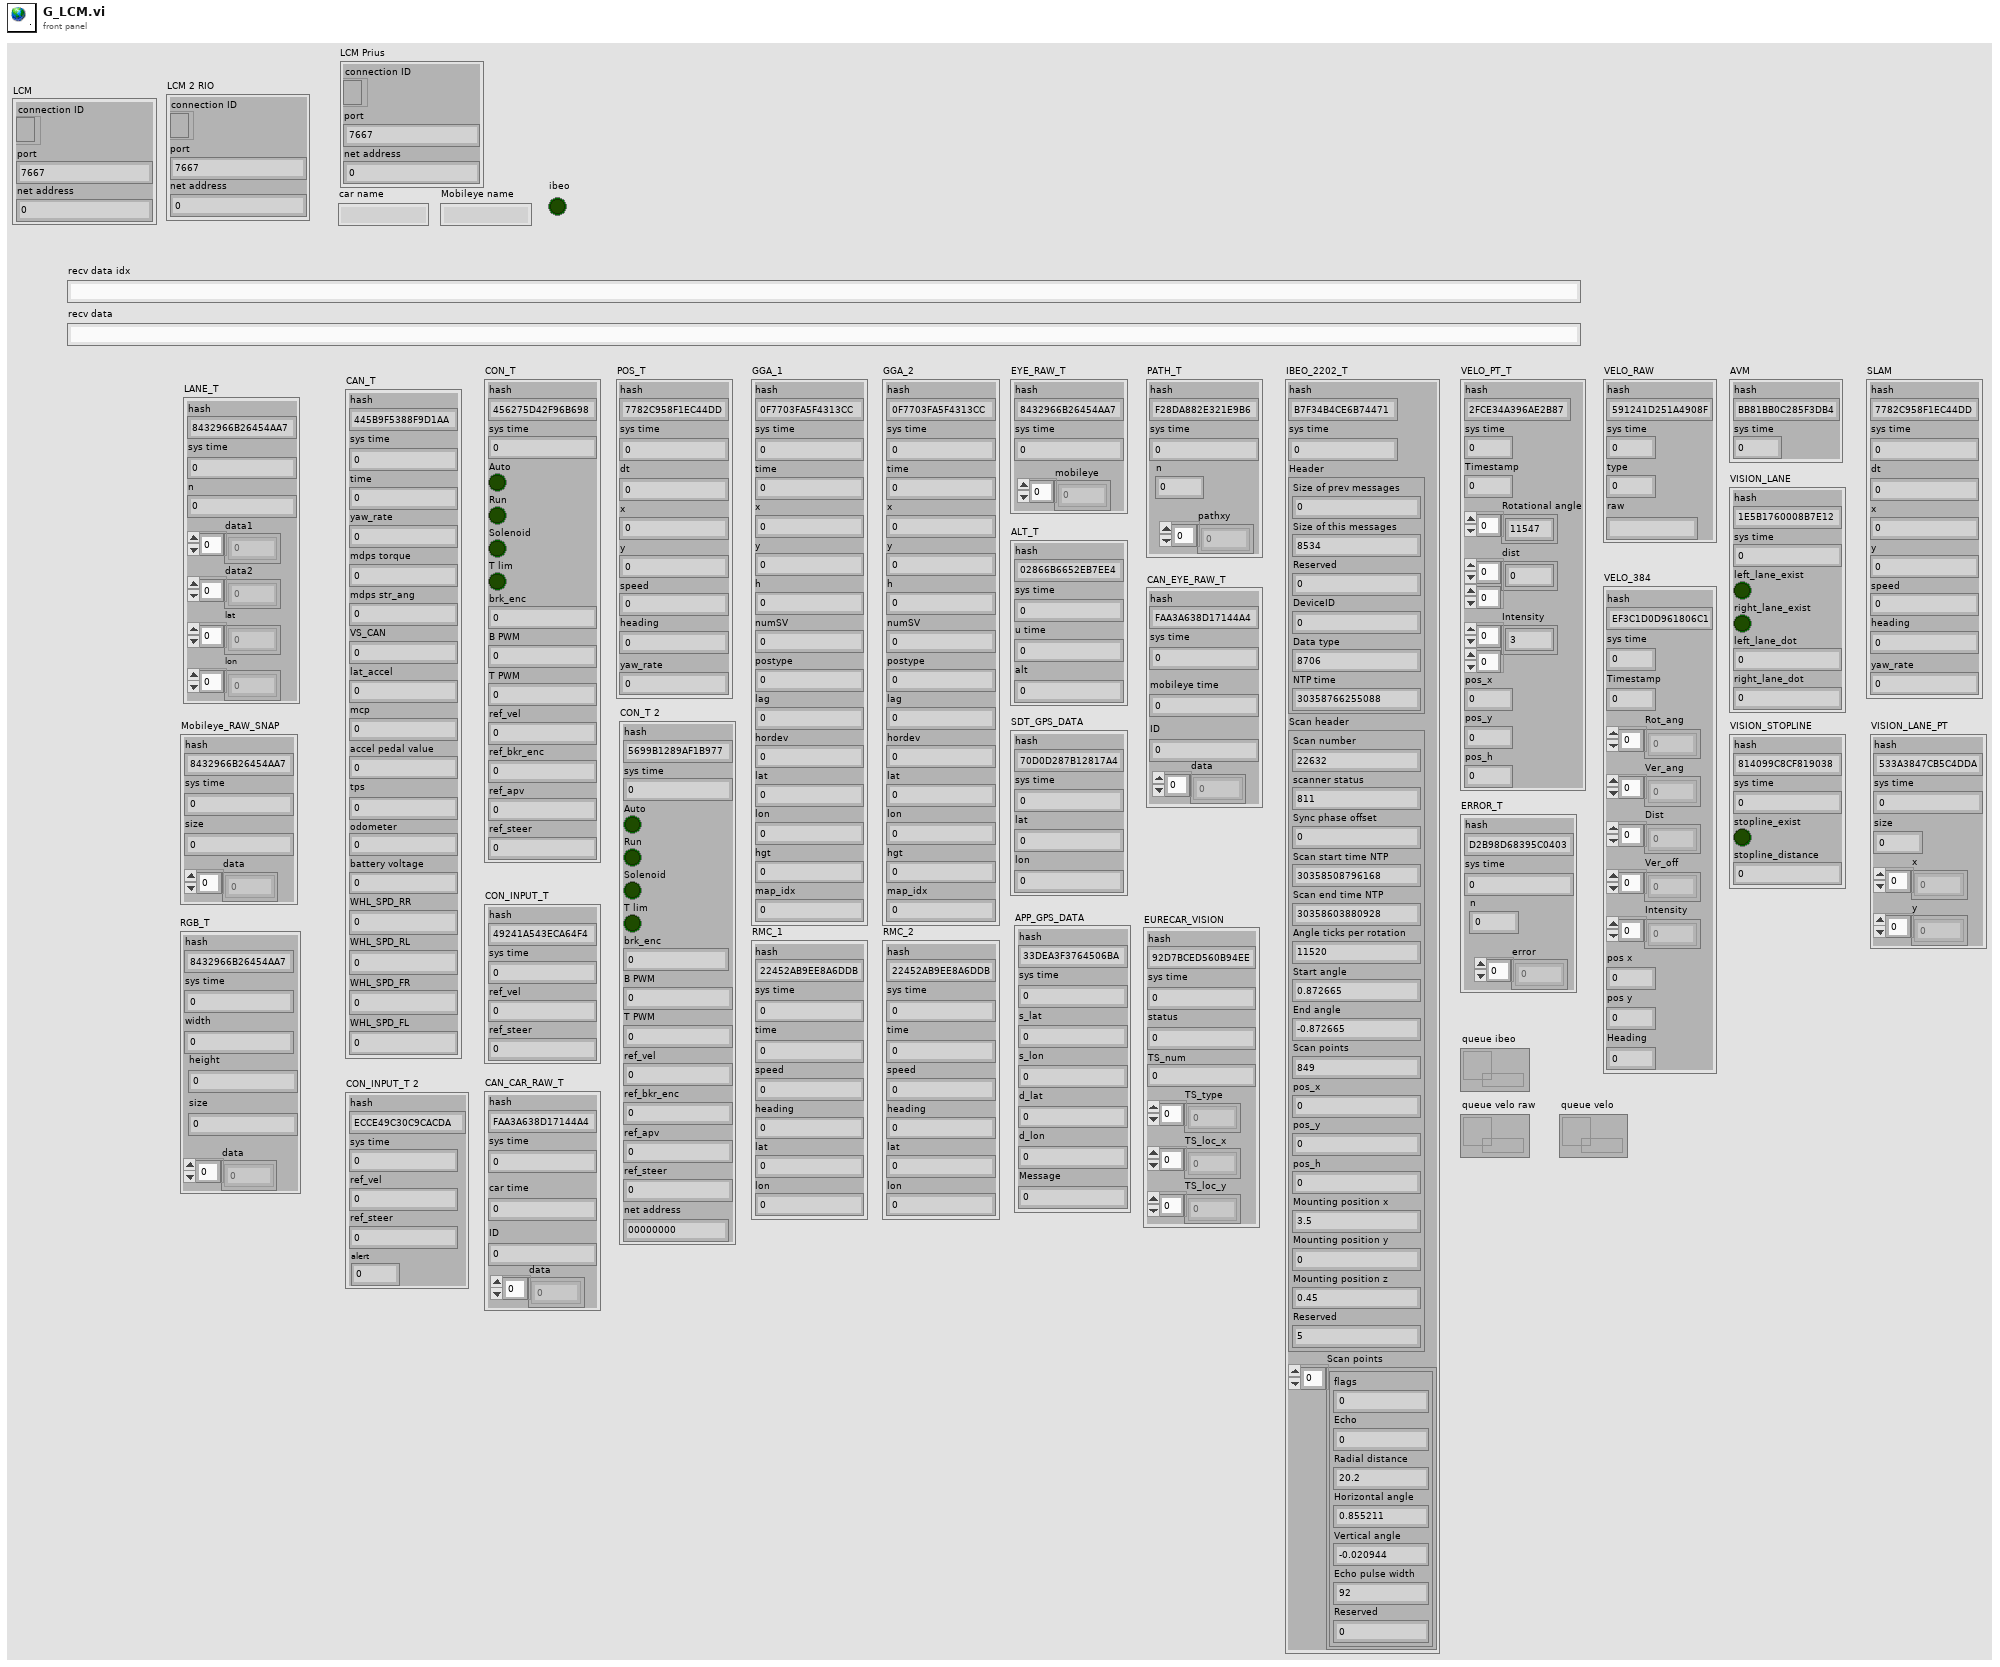
[diagram p1: front panel]
types:
  T1 = cluster{"hash":i64, "sys time":i64, "size":i64, "x":dbl[], "y":dbl[]}
  T2 = cluster{"hash":i64, "sys time":i64, "dt":dbl, "x":dbl, "y":dbl, "speed":dbl, "heading":dbl, "yaw_rate":dbl}
  T3 = cluster{"hash":i64, "sys time":i64, "stopline_exist":bool, "stopline_distance":dbl}
  T4 = cluster{"hash":i64, "sys time":i64, "left_lane_exist":bool, "right_lane_exist":bool, "left_lane_dot":dbl, "right_lane_dot":dbl}
  T5 = cluster{"hash":i64, "sys time":i64, "Auto":bool, "Run":bool, "Solenoid":bool, "T lim":bool, "brk_enc":u8, "B PWM":u16, "T PWM":u16, "ref_vel":dbl, "ref_bkr_enc":dbl, "ref_apv":dbl, "ref_steer":dbl, "net address":u32}
  T6 = cluster{"hash":i64, "sys time":i64, "Timestamp":u32, "Rot_ang":dbl[], "Ver_ang":dbl[], "Dist":dbl[], "Ver_off":dbl[], "Intensity":u8[], "pos x":dbl, "pos y":dbl, "Heading":dbl}
  T7 = cluster{"hash":i64, "sys time":i64, "type":u8, "raw":string}
  T8 = cluster{"hash":i64, "sys time":i64, "n":i32, "error":i32[]}
  T9 = cluster{"connection ID":refnum<k16>, "net address":u32, "port":u16}
  T10 = cluster{"hash":i64, "sys time":i64, "ref_vel":dbl, "ref_steer":dbl, "alert":u8}
  T11 = cluster{"hash":i64, "sys time":i64, "width":i32, "height":i32, "size":i32, "data":i32[]}
  T12 = cluster{"hash":i64, "sys time":i64, "size":i32, "data":u8[]}
  T13 = cluster{"hash":i64, "sys time":i64, "car time":u32, "ID":u32, "data":u8[]}
  T14 = cluster{"hash":i64, "sys time":i64, "mobileye time":u32, "ID":u32, "data":u8[]}
  T15 = cluster{"hash":i64, "sys time":i64, "status":i32, "TS_num":i32, "TS_type":i32[], "TS_loc_x":dbl[], "TS_loc_y":dbl[]}
  T16 = cluster{"hash":i64, "sys time":i64, "s_lat":dbl, "s_lon":dbl, "d_lat":dbl, "d_lon":dbl, "Message":i64}
  T17 = cluster{"hash":i64, "sys time":i64, "lat":dbl, "lon":dbl}
  T18 = cluster{"hash":i64, "sys time":i64, "n":u32, "pathxy":dbl[]}
  T19 = cluster{"hash":i64, "sys time":i64, "n":i32, "data1":dbl[], "data2":dbl[], "lat":dbl[], "lon":dbl[]}
  T20 = cluster{"hash":i64, "sys time":i64, "u time":i64, "alt":dbl}
  T21 = cluster{"hash":i64, "sys time":i64, "time":dbl, "yaw_rate":dbl, "mdps torque":dbl, "mdps str_ang":dbl, "VS_CAN":dbl, "lat_accel":dbl, "mcp":dbl, "accel pedal value":dbl, "tps":dbl, "odometer":dbl, "battery voltage":dbl, "WHL_SPD_RR":dbl, "WHL_SPD_RL":dbl, "WHL_SPD_FR":dbl, "WHL_SPD_FL":dbl}
  T22 = cluster{"hash":i64, "sys time":i64, "Timestamp":u32, "Rotational angle":u16[], "dist":u16[][], "Intensity":u8[][], "pos_x":dbl, "pos_y":dbl, "pos_h":dbl}
  T23 = cluster{"hash":i64, "sys time":i64, "ref_vel":dbl, "ref_steer":dbl}
  T24 = cluster{"hash":i64, "sys time":i64, "Header":cluster{"Size of prev messages":u32, "Size of this messages":u32, "Reserved":u8, "DeviceID":u8, "Data type":u16, "NTP time":u64}, "Scan header":cluster{"Scan number":u16, "scanner status":u16, "Sync phase offset":u16, "Scan start time NTP":u64, "Scan end time NTP":u64, "Angle ticks per rotation":u16, "Start angle":dbl, "End angle":dbl, "Scan points":u16, "pos_x":dbl, "pos_y":dbl, "pos_h":dbl, "Mounting position x":dbl, "Mounting position y":dbl, "Mounting position z":dbl, "Reserved":u16}, "Scan points":cluster{"flags":u8, "Echo":u8, "Radial distance":dbl, "Horizontal angle":dbl, "Vertical angle":dbl, "Echo pulse width":u16, "Reserved":u16}[]}
  T25 = cluster{"hash":i64, "sys time":i64, "time":dbl, "x":dbl, "y":dbl, "h":dbl, "numSV":i32, "postype":i32, "lag":i32, "hordev":dbl, "lat":dbl, "lon":dbl, "hgt":dbl, "map_idx":i32}
  T26 = cluster{"hash":i64, "sys time":i64, "time":dbl, "speed":dbl, "heading":dbl, "lat":dbl, "lon":dbl}
  T27 = cluster{"hash":i64, "sys time":i64, "Auto":bool, "Run":bool, "Solenoid":bool, "T lim":bool, "brk_enc":u8, "B PWM":u16, "T PWM":u16, "ref_vel":dbl, "ref_bkr_enc":dbl, "ref_apv":dbl, "ref_steer":dbl}
  T28 = cluster{"hash":i64, "sys time":i64, "mobileye":u8[]}
diagram:
